vi "TC.vi"() -> ()   [LabVIEW 2013]
uses:
  lib/Lib.llb/CS mode.ctl
  lib/Lib.llb/R.ctl
  lib/Lib.llb/T.ctl
  lib/Lib.llb/Calibrations.ctl
  lib/Lib.llb/CS.lvclass
  lib/Lib.llb/PID Settings.ctl
  lib/Lib.llb/AVS_exc_n_ranges.ctl
  lib/Lib.llb/AVS_excitation.ctl
  lib/Lib.llb/AVS47_range.ctl
  lib/Lib.llb/Ch descriptions.ctl
  lib/Lib.llb/Cursor Controls.ctl
  lib/Lib.llb/DataArray.ctl
  lib/Lib.llb/Unit.ctl
  lib/Lib.llb/Control 6.ctl
  lib/Lib.llb/Control 4.ctl
  lib/Lib.llb/Control 8.ctl
  lib/Lib.llb/VI FPO Ref.ctl
  lib/Lib.llb/Class ID ENUM.ctl
  lib/Lib.llb/Type Descriptor Enumeration__ogtk.ctl
  lib/Lib.llb/Refnum Subtype Enum__ogtk.ctl
  lib/Lib.llb/Waveform Subtype Enum__ogtk.ctl
  lib/Lib.llb/LV Data cluster.ctl
  lib/Lib.llb/Action.ctl
  Leiden to DSC/TC to DSC/Typedefs/TC-cluster.ctl
  lib/Lib.llb/TCS.lvclass
  lib/Lib.llb/QCS.lvclass
  lib/Lib.llb/CS Emulation.lvclass
  lib/Lib.llb/PCS.lvclass
  lib/Lib.llb/Byte Params.ctl
panel:
  out "R_array":dbl[](array[numeric])
  out "SetControl":T1
  out "ControlNames":string[](array[string])
  out "VIRef":T2 {"Array DataType" format="%.0x"; "WaveForm Type" format="%.0x"; "RefNum Type" format="%.0x"; "DataType" format="%.0x"}
  out "zConfig":path=path "C:/Users/Sasha/Dropbox/Labview/LC Software/ImpSoft-V5.2.2-multithreaded/ImpBridgeLabview/ImpBridgeDll.dll"
  out "VI called?":bool=TRUE
  out "Error code":u8
  out "Set #":u8 caption="zBridge set nr."
  out "zDll":path=path "C:/Users/Sasha/Dropbox/Labview/LC Software/ImpSoft-V5.2.2-multithreaded/ImpBridgeLabview/ImpBridgeDll.dll"
  in  "String":string="^ Click the Run button to start the program "
  in  "Toolbar":enum32{"Page 1", "Page 2"}(tab)
  in  "Load config":bool
  in  "Start":bool
  in  "Load Data":bool
  in  "Pause":bool
  in  "Stop":bool
  in  "Copy to Clipboard":bool
  in  "Save to Cal Log":bool
  in  "Save config":bool
  in  "Clear all plots":bool
  in  "ColorBox":enum32{"Page 1", "Page 2"}(tab)
  in  "Colors":picture
  out "Color":u32(colorbox)
  in  "LogFileCreationTime":timestamp=timestamp(2742897600 s since 1904-01-01)
  out "Calib path":path=path "C:/avs-47/aaaa"
  out "Log path":path
  out "TCS port":i32(ring)=3 items=["COM1", "COM2", "COM3", "COM4", "COM5", "COM6", "COM7", "COM8", "COM9", "PRN1", "PRN2", "PRN3", "PRN4"]
  out "AVS VISA session":refnum<visa-resource-name>="COM3"
  in  "Minimize 2":bool
  out "Revision":string="TC" caption="V"
  in  "Minimize":bool
  out "Current1flow":bool
  out "Current2flow":bool
  in  "Tab Control":enum32{"AVS"}(tab)
  in  "Graph controls":enum32{"Page 1"}(tab)
  in  "Mode Buttons":T7
  in  "Erase all":bool
  in  "Plot-Save All":bool
  in  "Plot-save-screen":bool
  in  "Channel Controls":T8(tab)=enum."All"
  out "T0":dbl=nan caption="T" format="%#.2p"
  out "R0":dbl caption="R" format="%.3p"
  out "R-Plot 0":cluster{dbl[], dbl[]}(graph) caption="R-Plot"
  out "T1":dbl=nan caption="T" format="%#.2p"
  out "R1":dbl caption="R" format="%.3p"
  out "R-Plot 1":cluster{dbl[], dbl[]}(graph) caption="R-Plot"
  out "T2":dbl=nan caption="T" format="%#.2p"
  out "R2":dbl caption="R" format="%.3p"
  out "R-Plot 2":cluster{dbl[], dbl[]}(graph) caption="R-Plot"
  out "T3":dbl=nan caption="T" format="%#.2p"
  out "R3":dbl caption="R" format="%.3p"
  out "R-Plot 3":cluster{dbl[], dbl[]}(graph) caption="R-Plot"
  out "T4":dbl=nan caption="T" format="%#.2p"
  out "R4":dbl caption="R" format="%.3p"
  out "R-Plot 4":cluster{dbl[], dbl[]}(graph) caption="R-Plot"
  out "T5":dbl=nan caption="T" format="%#.2p"
  out "R5":dbl caption="R" format="%.3p"
  out "R-Plot 5":cluster{dbl[], dbl[]}(graph) caption="R-Plot"
  out "T6":dbl=nan caption="T" format="%#.2p"
  out "R6":dbl caption="R" format="%.3p"
  out "R-Plot 6":cluster{dbl[], dbl[]}(graph) caption="R-Plot"
  out "T7":dbl=nan caption="T" format="%#.2p"
  out "R7":dbl caption="R" format="%.3p"
  out "R-Plot 7":cluster{dbl[], dbl[]}(graph) caption="R-Plot"
  out "T8":dbl=nan caption="T" format="%#.2p"
  out "R8":dbl caption="R" format="%.3p"
  out "R-Plot 8":cluster{dbl[], dbl[]}(graph) caption="R-Plot"
  out "T9":dbl=nan caption="T" format="%#.2p"
  out "R9":dbl caption="R" format="%.3p"
  out "R-Plot 9":cluster{dbl[], dbl[]}(graph) caption="R-Plot"
  out "T":T9 {"T0 3" format="%.2p"; "T0 2" format="%.2p"; "T0" format="%.2p"; "T0" format="%.2p"; "T0" format="%.2p"; "T0" format="%.2p"; "T0" format="%.2p"; "T0" format="%.2p"; "T0" format="%.2p"; "T0" format="%.2p"}
  in  "AVS names":T10={"AVS Name 0"="3K", "AVS Name 1"="Still", "AVS Name 2"="50 mK", "AVS Name 3"="MC", "AVS Name 4"="MC", "AVS Name 5"="", "AVS Name 6"="", "AVS Name 7"="", "AVS Name 8"="", "AVS Name 9"=""}
  in  "Edit Calibrations":T11
  in  "Thermometer":T12 {"Select sensor 10" items=["No Calibration.vi"]; "Select sensor 9" items=["No Calibration.vi"]; "Select sensor 8" items=["No Calibration.vi"]; "Select sensor 7" items=["No Calibration.vi"]; "Select sensor 6" items=["No Calibration.vi"]; "Select sensor 5" items=["No Calibration.vi"]; "Select sensor 4" items=["No Calibration.vi"]; "Select sensor 3" items=["No Calibration.vi"]; "Select sensor 2" items=["No Calibration.vi"]; "Select sensor 1" items=["No Calibration.vi"]}
  out "Units":T13
  out "R":T14={"R0"=0.0, "R1"=0.0, "R2"=-0.0, "R3"=0.0, "R4"=0.0, "R5"=0.0, "R6"=0.0, "R7"=0.0, "R6 2"=0.0, "R7 2"=0.0} {"R7 2" format="%.3p"; "R6 2" format="%.3p"; "R7" format="%.3p"; "R6" format="%.3p"; "R5" format="%.3p"; "R4" format="%.3p"; "R3" format="%.3p"; "R2" format="%.3p"; "R1" format="%.3p"; "R0" format="%.3p"}
  in  "Scan Parameters":enum32{"Page 1", "Page 2"}(tab)
  in  "Exc&Ranges":T15={"Excitationl 0"=4, "Excitationl 0"=4, "Excitationl 0"=3, "Excitationl 0"=3, "Excitationl 0"=3, "Excitationl 0"=3, "Excitationl 0"=3, "Excitationl 0"=3, "Range 0"=5, "Range 0"=5, "Range 0"=5, "Range 0"=5, "Range 0"=5, "Range 0"=5, "Range 0"=5, "Range 0"=5} {"Range 0" items=["n.a."=-1, "open"=0, "2 Ohm"=1, "20 Ohm"=2, "200 Ohm"=3, "2k Ohm"=4, "20k Ohm"=5, "200k Ohm"=6, "2M Ohm"=7]; "Range 0" items=["n.a."=-1, "open"=0, "2 Ohm"=1, "20 Ohm"=2, "200 Ohm"=3, "2k Ohm"=4, "20k Ohm"=5, "200k Ohm"=6, "2M Ohm"=7]; "Range 0" items=["n.a."=-1, "open"=0, "2 Ohm"=1, "20 Ohm"=2, "200 Ohm"=3, "2k Ohm"=4, "20k Ohm"=5, "200k Ohm"=6, "2M Ohm"=7]; "Range 0" items=["n.a."=-1, "open"=0, "2 Ohm"=1, "20 Ohm"=2, "200 Ohm"=3, "2k Ohm"=4, "20k Ohm"=5, "200k Ohm"=6, "2M Ohm"=7]; "Range 0" items=["n.a."=-1, "open"=0, "2 Ohm"=1, "20 Ohm"=2, "200 Ohm"=3, "2k Ohm"=4, "20k Ohm"=5, "200k Ohm"=6, "2M Ohm"=7]; "Range 0" items=["n.a."=-1, "open"=0, "2 Ohm"=1, "20 Ohm"=2, "200 Ohm"=3, "2k Ohm"=4, "20k Ohm"=5, "200k Ohm"=6, "2M Ohm"=7]; "Range 0" items=["n.a."=-1, "open"=0, "2 Ohm"=1, "20 Ohm"=2, "200 Ohm"=3, "2k Ohm"=4, "20k Ohm"=5, "200k Ohm"=6, "2M Ohm"=7]; "Range 0" items=["n.a."=-1, "open"=0, "2 Ohm"=1, "20 Ohm"=2, "200 Ohm"=3, "2k Ohm"=4, "20k Ohm"=5, "200k Ohm"=6, "2M Ohm"=7]; "Excitationl 0" items=["none", "3 µV", "10 µV", "30 µV", "100 µV", "300 µV", "1 mV", "3 mV"]; "Excitationl 0" items=["none", "3 µV", "10 µV", "30 µV", "100 µV", "300 µV", "1 mV", "3 mV"]; "Excitationl 0" items=["none", "3 µV", "10 µV", "30 µV", "100 µV", "300 µV", "1 mV", "3 mV"]; "Excitationl 0" items=["none", "3 µV", "10 µV", "30 µV", "100 µV", "300 µV", "1 mV", "3 mV"]; "Excitationl 0" items=["none", "3 µV", "10 µV", "30 µV", "100 µV", "300 µV", "1 mV", "3 mV"]; "Excitationl 0" items=["none", "3 µV", "10 µV", "30 µV", "100 µV", "300 µV", "1 mV", "3 mV"]; "Excitationl 0" items=["none", "3 µV", "10 µV", "30 µV", "100 µV", "300 µV", "1 mV", "3 mV"]; "Excitationl 0" items=["none", "3 µV", "10 µV", "30 µV", "100 µV", "300 µV", "1 mV", "3 mV"]}
  out "Status":T18
  out "zBridge params":T19
  out "uPlots":T20
  in  "Autorange":bool=TRUE
  out "Active":T21={"active Channel 0"=TRUE, "active Channel 1"=TRUE, "active Channel 2"=TRUE, "active Channel 3"=FALSE, "active Channel 4"=FALSE, "active Channel 5"=FALSE, "active Channel 6"=FALSE, "active Channel 7"=FALSE, "active Channel 8"=FALSE, "active Channel 9"=FALSE}
  out "Waveform Chart":T22(graph)
  in  "HW Address":u32
  in  "Edit calibration":bool
  in  "Convert":bool
  out "T7":dbl caption="T=" format="%#.2p"
  in  "QuickR":dbl caption="R=" format="%_6g"
  in  "Select sensor 1":u16(ring) items=["No Calibration.vi"]
  out "I_list[i]":T23[](array[typedef]) min=-1.0
  out "I_in":T23[](array[typedef]) min=-1.0
  in  "Tab Control 5":enum32{"Page 1", "Page 2"}(tab)
  in  "Data History":enum32{"History", "Settings"}(tab)=enum."Settings"
  out "AVS names small":T10={"AVS Name 0"="3K", "AVS Name 1"="Still", "AVS Name 2"="50 mK", "AVS Name 3"="MC", "AVS Name 4"="MC", "AVS Name 5"="", "AVS Name 6"="", "AVS Name 7"="", "AVS Name 8"="", "AVS Name 9"=""}
  out "Active channel":T24
  out "Small T":T25 caption="T" {"R1" format="%#.2p"; "R1" format="%#.2p"; "R1" format="%#.2p"; "R1" format="%#.2p"; "R1" format="%#.2p"; "R1" format="%#.2p"; "R1" format="%#.2p"; "R1" format="%#.2p"; "R1" format="%#.2p"; "R1" format="%#.2p"}
  out "Small R":T26 caption="R" {"R1 2" format="%#_5p"; "R1 2" format="%#_5p"; "R1 2" format="%#_5p"; "R1 2" format="%#_5p"; "R1 2" format="%#_5p"; "R1 2" format="%#_5p"; "R1 2" format="%#_5p"; "R1 2" format="%#_5p"; "R1 2" format="%#_5p"; "R1 2" format="%#_5p"}
  out "Time":dbl format="%<%X\n%x>T"
  in  "Runtime Settings":T27={"Read AVS channels from"=0, "Last Channel"=7, "Delay Between Scans"=0, "Stabilisation Delay"=5.0, "Averages"=2, "Data Memory"=25000, "Filter graphs:"=FALSE, "Y_min"=0.0, "Y_max"=2000000.0, "Plot type"=enum."T vs Time", "Allow neg R"=TRUE, "Data Memory 2"=30.0} {"Data Memory 2" min=0.0; "Delay Between Scans" format="%.0f s"; "Averages" min=1 max=1000; "Stabilisation Delay" min=0.5; "Last Channel" min=0 max=7 step=1; "Read AVS channels from" min=0 max=7 step=1; "Y_max" format="%#_6f"; "Y_min" min=0.0 format="%#_6f"; "Data Memory" min=3 max=30000}
  in  "Numeric":dbl
  out "I":dbl[](array[numeric])
  in  "Data":T28=[{"R"=[], "T"=[], "Time"=[]}, {"R"=[0.0, 2.0], "T"=[], "Time"=[]}]
  out "Int":dbl=10.0 format="%#.2f"
  out "T_array":dbl[](array[numeric])
  in  "Data array":dbl[](array[numeric])
  out "I3_SetPnt":dbl
  out "Currents changed":bool
  in  "Excitations":T29={"Excitationl 0"=4, "Excitation 1"=4, "Excitation 2"=3, "Excitation 3"=3, "Excitation 4"=3, "Excitation 5"=3, "Excitation 6"=3, "Excitation 7"=3} {"Excitation 7" items=["none", "3 µV", "10 µV", "30 µV", "100 µV", "300 µV", "1 mV", "3 mV"]; "Excitation 6" items=["none", "3 µV", "10 µV", "30 µV", "100 µV", "300 µV", "1 mV", "3 mV"]; "Excitation 5" items=["none", "3 µV", "10 µV", "30 µV", "100 µV", "300 µV", "1 mV", "3 mV"]; "Excitation 4" items=["none", "3 µV", "10 µV", "30 µV", "100 µV", "300 µV", "1 mV", "3 mV"]; "Excitation 3" items=["none", "3 µV", "10 µV", "30 µV", "100 µV", "300 µV", "1 mV", "3 mV"]; "Excitation 2" items=["none", "3 µV", "10 µV", "30 µV", "100 µV", "300 µV", "1 mV", "3 mV"]; "Excitation 1" items=["none", "3 µV", "10 µV", "30 µV", "100 µV", "300 µV", "1 mV", "3 mV"]; "Excitationl 0" items=["none", "3 µV", "10 µV", "30 µV", "100 µV", "300 µV", "1 mV", "3 mV"]}
  in  "Ranges":T29={"Excitationl 0"=5, "Excitation 1"=5, "Excitation 2"=5, "Excitation 3"=5, "Excitation 4"=5, "Excitation 5"=5, "Excitation 6"=5, "Excitation 7"=5} {"Excitation 7" items=["n.a."=-1, "open"=0, "2 Ohm"=1, "20 Ohm"=2, "200 Ohm"=3, "2k Ohm"=4, "20k Ohm"=5, "200k Ohm"=6, "2M Ohm"=7]; "Excitation 6" items=["n.a."=-1, "open"=0, "2 Ohm"=1, "20 Ohm"=2, "200 Ohm"=3, "2k Ohm"=4, "20k Ohm"=5, "200k Ohm"=6, "2M Ohm"=7]; "Excitation 5" items=["n.a."=-1, "open"=0, "2 Ohm"=1, "20 Ohm"=2, "200 Ohm"=3, "2k Ohm"=4, "20k Ohm"=5, "200k Ohm"=6, "2M Ohm"=7]; "Excitation 4" items=["n.a."=-1, "open"=0, "2 Ohm"=1, "20 Ohm"=2, "200 Ohm"=3, "2k Ohm"=4, "20k Ohm"=5, "200k Ohm"=6, "2M Ohm"=7]; "Excitation 3" items=["n.a."=-1, "open"=0, "2 Ohm"=1, "20 Ohm"=2, "200 Ohm"=3, "2k Ohm"=4, "20k Ohm"=5, "200k Ohm"=6, "2M Ohm"=7]; "Excitation 2" items=["n.a."=-1, "open"=0, "2 Ohm"=1, "20 Ohm"=2, "200 Ohm"=3, "2k Ohm"=4, "20k Ohm"=5, "200k Ohm"=6, "2M Ohm"=7]; "Excitation 1" items=["n.a."=-1, "open"=0, "2 Ohm"=1, "20 Ohm"=2, "200 Ohm"=3, "2k Ohm"=4, "20k Ohm"=5, "200k Ohm"=6, "2M Ohm"=7]; "Excitationl 0" items=["n.a."=-1, "open"=0, "2 Ohm"=1, "20 Ohm"=2, "200 Ohm"=3, "2k Ohm"=4, "20k Ohm"=5, "200k Ohm"=6, "2M Ohm"=7]}
  out "CS ref":refnum<class "CS.lvclass">
  out "start 2":bool
  in  "Current indicators":enum32{"Page 1", "Page 2"}(tab)
  out "Automatic mode 0":bool
  out "Automatic mode 1":bool
  out "Map Channel 0 to 2":T30(ring) caption="Output to"
  in  "uA 0":u32
  in  "CS Names":T31={"CS Name 0"="N.C.", "CS Name 1"="3K", "CS Name 2"="Still", "CS Name 3"="MC"}
  out "I0":T32={"uA"="000", "ON"=FALSE, "Gated"=FALSE, "current flows"=FALSE, "Error"=FALSE} caption="Ch0 -"
  in  "uA 3":u32
  in  "uA 2":u32
  in  "uA 1":u32
  out "Automatic mode 3":bool
  out "Automatic mode 2":bool
  out "I3":T32={"uA"="000", "ON"=FALSE, "Gated"=FALSE, "current flows"=FALSE, "Error"=FALSE} caption="Chn 3"
  out "I2":T32={"uA"="000", "ON"=FALSE, "Gated"=FALSE, "current flows"=FALSE, "Error"=FALSE} caption="Chn 2"
  out "I1":T32={"uA"="000", "ON"=FALSE, "Gated"=FALSE, "current flows"=FALSE, "Error"=FALSE} caption="Chn 1"
  out "I_0":dbl=10.0
  out "vi reference":refnum<vi>
  out "Small I":cluster{"I1":dbl, "I2":dbl, "I3":dbl, "I4":dbl} caption="I" {"I1" format="%#.2f"; "I2" format="%#.2p"; "I3" format="%#.2p"; "I4" format="%#.2p"}
  out "Actual I":dbl[](array[numeric])
  in  "Save Data 2":bool
  in  "Show PID graph?":bool
  in  "Set Color":bool
  out "Unit":string
  out "Par/Err":string caption="zBridge params/Error"
  out "CurCalibrations":T33
  out "LMB Down":bool
  in  "Tab Control 2":T34(tab)
  in  "Refresh Calibrations":bool
  in  "zBridge settings":bool
  out "ID":string
  out "CS status":errorcluster
  out "General":errorcluster caption="General status"
  in  "Bridge settings":T35={"AVS type"=enum."AVS47A (GPIB interface)", "AVS_SPort"="COM5", "Address"="GPIB0::20::INSTR", "AVS_CalFolder"=path "E:/Dropbox/Labview/LC Software/All Calibrations"}
  in  "Current source settings":T36={"TCS_Port"="COM1", "TCS_Imax"=5, "CS type"=enum."TCS", "QCS/PCS Device"=0}
  in  "Data logging":T37={"AVS_Path"=path "C:/avs-47", "AVS_FName"="LogAVS", "CAL_FName"="calibration", "Filenames suffix"="_%Y-%m-%d-%H-%M-%S", "Delimeter"="\t", "NewFevery"=7, "Time Units"=enum."Days", "Date/Time Format"="%Y-%m-%d %H:%M:%S", "External VI path"=path "C:/Users/User1/Dropbox/Labview/LC Software/TempControl/OnTempStabilized Ext VI Laurens.vi", "Ask on start?"=FALSE, "Run description"="\n"}
  out "Bridge status":errorcluster
  in  "I0 output to":T38(ring) caption="Set Channel 0 output to"
  in  "CS Mode":T39 caption="CS mode"
  out "Time Old":dbl format="%#_16g"
  in  "CS modes":T40(tab)=enum."Automatic 1"
  in  "C_I0 4":T41={"Toggle ON/OFF"=FALSE, "Toggle Gated"=FALSE, "I"=0, "Range"=enum."x1 uA"} caption="Chn 3" {"I" max=100000 step=1}
  in  "C_I0 3":T41={"Toggle ON/OFF"=FALSE, "Toggle Gated"=FALSE, "I"=0, "Range"=enum."x1 uA"} caption="Chn 2" {"I" max=100000 step=1}
  in  "C_I0 2":T41={"Toggle ON/OFF"=FALSE, "Toggle Gated"=FALSE, "I"=0, "Range"=enum."x1 uA"} caption="Chn 1" {"I" max=100000 step=1}
  in  "C_I0":T41={"Toggle ON/OFF"=FALSE, "Toggle Gated"=FALSE, "I"=0, "Range"=enum."x1 uA"} caption="Chn 0" {"I" max=100000 step=1}
  in  "Mode1 ON":bool
  in  "I_list":T23[][](array[typedef]) min=-1.0
  out "T Channel":T42[](array[typedef])
  out "I_selection":T43[](array[typedef])=[TRUE, FALSE, FALSE, FALSE, FALSE, FALSE, FALSE, FALSE, FALSE, FALSE]
  out "SP reached?":bool
  out "Error":dbl=10.0 format="%#_6f"
  out "Slope":dbl format="%#_3g %"
  out "Timer":dbl format="%<%H:%M:%S>t"
  out "I_list_idx_max":i32=10 caption="/"
  out "I_list_idx":i32=10 caption="Point #"
  in  "Next step":bool
  in  "Reset PID":bool
  in  "PID setup":T44={"Current limit, [uA]"=10000.0, "Proportional Gain"=3.0, "Integral Gain"=3.0, "Derivative Gain"=1.0, "SP tolerance"=0.1, "Feed Fwd Gain [uA/mK]"=0.0, "Integral Gain Bandwidth"=10.0, "Integral Gain Background"=1.0, "FB on 2"=enum."1"} {"Integral Gain Background" format="%#.6g"; "Integral Gain Bandwidth" format="%#.6g"; "Feed Fwd Gain [uA/mK]" format="%#.5g"; "SP tolerance" format="%#.5g"; "Derivative Gain" format="%#.6g"; "Integral Gain" format="%#.6g"; "Proportional Gain" format="%#.6g"; "Current limit, [uA]" format="%#.5g"}
  in  "Automode 2":bool=TRUE caption="Enable automatic sweeping/list iteration"
  in  "Automode Settings 2":T45={"AVS Channel"=0, "N averages"=10, "Delay Time"=10.0, "T stability"=0.3, "FB on"=enum."Temperature"} {"Delay Time" min=0.0 format="%#_g min"; "AVS Channel" min=-1 max=9 step=1}
  in  "Call ext. VI":bool
  out "- state":T46(ring)
  in  "Trigger other running TC instances":bool
  in  "I_prev":bool
  in  "I_next":bool
  in  "I_tofirst":bool
  in  "Save to file":bool
  in  "Load from file":bool
  in  "Write to log":bool
  in  "I3 as temp":cluster{"I3 as temp 2":bool}
  in  "I_Clear":bool
  in  "Mode2 ON":bool
  in  "FB on":enum16{"Resistance", "Temperature"}(ring)=enum."Temperature" caption="Read"
  in  "AVS Channel":i32 caption="on channel" min=-1 max=9 step=1
  in  "Add Range":bool
  in  "Array":dbl[](array[numeric])=[0.0, 0.0, 0.0, 0.0, 0.0, 0.0] caption="New range" min=-1.0
  in  "I_list 2":dbl[][](array[numeric])=[[0.0, 0.0, 0.0, 0.0, 0.0, inf]] min=-1.0
  out "I_selection 2":T43[](array[typedef])=[TRUE, FALSE, FALSE, FALSE, FALSE, FALSE, FALSE, FALSE, FALSE, FALSE]
  in  "CS Ch3 mode":enum32{"Page 1", "Page 2"}(tab)=enum."Page 2"
  in  "T Sweep":T47={"Start value"=200.0, "End value"=250.0, "Step"=10.0, "Current"=0.0, "I_next"=FALSE, "I_prev"=FALSE, "Interrrupt Sweep"=FALSE, "Start"=FALSE, "Boolean"=TRUE} {"Step" min=0.0; "End value" min=0.0; "Start value" min=0.0}
  # "Quick convert R->T:"
  # "Ohm"
  # "mK"
  # "Ch#"
  # "Miniplot"
  # "Channel parameters"
  # "Impedance"
  # "Unit"
  # "Type of sensor"
  # "T [mK]"
  # "Description"
  # "0"
  # "1"
  # "2"
  # "3"
  # "4"
  # "5"
  # "6"
  # "7"
  # "8"
  # "9"
  # "0"
  # "1"
  # "2"
  # "3"
  # "4"
  # "5"
  # "7"
  # "8"
  # "9"
  # "6"
  # "auto"
  # "auto"
  # "auto"
  # "auto"
  # "gated"
  # "gated"
  # "gated"
  # "gated"
  # "Status"
  # "Current source mode"
  # "Current source manual control"
  # "Current source automatic mode #1"
  # "Currents List"
  # "Settings"
  # "I0"
  # "I1"
  # "I2"
  # "I3"
  # "Status"
  # "On temperature stabilized"
  # "Current source automatic mode #2"
  # "Currents List"
  # "Settings"
  # "T0"
  # "T1"
  # "I0"
  # "I1"
  # "I2"
  # "I3"
  # "T0"
  # "T1"
  # "I0"
  # "I1"
  # "I2"
  # "I3"
  # "Ch3"
types:
  T1 = typedef "LV Data cluster.ctl" = cluster{"Name":string, "Scalar":string, "Array":string[][]}
  T2 = typedef "VI FPO Ref.ctl" = cluster{"Control Ref ID":refnum<vi>[], "Full Name":string[], "ClassID":T3[], "Short Name":string[], "DataType":T4[], "RefNum Type":T5[], "WaveForm Type":T6[], "Parent":i32[], "Array DataType":T4[], "Owning VI":refnum<vi>[], "Active?":bool[]}
  T3 = typedef "Class ID ENUM.ctl" = enum16{"<Null>", "1", "2", "Generic", "Decoration", "Text", "Control", "ColorBox", "Boolean", "RefNum", "Variant", "Path", "ListBox", "Table", "Array", "Picture", "ActiveXContainer", "Numeric", "Digital", "NamedNumeric", "ColorRamp", "Slide", "GraphOrChart", "WaveformChart", "WaveformGraph", "IntensityChart", "IntensityGraph", "String", "IOName", "ComboBox", "Cluster", "Panel", "Knob", "NumWithScale", "Ring", "Enum", "GObject", "Plot", "Cursor", "NumericText", "Scale", "ColorScale", "GraphScale", "ColorGraphScale", "TypedRefNum", "OldKnobScale", "MCListbox", "MeasureData", "BVTag", "DAQName", "VISAName", "IVIName", "SlideScale", "TabControl", "Page", "TabArrayTabControl", "ConPane", "57", "58", "59", "60", "61", "62", "63", "64", "SubPanel", "TreeControl", "67", "68", "69", "70", "71", "72", "73", "74", "75", "SplitterBar"}
  T4 = typedef "Type Descriptor Enumeration__ogtk.ctl" = enum8{"<Null>", "I8", "I16", "I32", "I64", "U8", "U16", "U32", "U64", "SGL", "DBL", "EXT", "CSG", "CDB", "CXT", "0x0F", "0x10", "0x11", "0x12", "0x13", "0x14", "Enum U8", "Enum U16", "Enum U32", "Enum U64", "SGL PQ", "DBL PQ", "EXT PQ", "CSG PQ", "CDB PQ", "CXT PQ", "0x1F", "0x20", "Boolean", "0x22", "0x23", "0x24", "0x25", "0x26", "0x27", "0x28", "0x29", "0x2A", "0x2B", "0x2C", "0x2D", "0x2E", "0x2F", "String", "0x31", "Path", "Pict", "0x34", "0x35", "0x36", "DAQ", "0x38", "0x39", "0x3A", "0x3B", "0x3C", "0x3D", "0x3E", "0x3F", "Array", "0x41", "0x42", "0x43", "0x44", "0x45", "0x46", "0x47", "0x48", "0x49", "0x4A", "0x4B", "0x4C", "0x4D", "0x4E", "0x4F", "Cluster", "0x51", "0x52", "Variant", "Waveform", "0x55", "0x56", "0x57", "0x58", "0x59", "0x5A", "0x5B", "0x5C", "0x5D", "0x5E", "0x5F", "0x60", "0x61", "0x62", "0x63", "0x64", "0x65", "0x66", "0x67", "0x68", "0x69", "0x6A", "0x6B", "0x6C", "0x6D", "0x6E", "0x6F", "Refnum"}
  T5 = typedef "Refnum Subtype Enum__ogtk.ctl" = enum8{"Generic", "Datalog File Refnum", "Byte Stream File Refnum", "Device Refnum", "Occurence Refnum", "TCP Connection Refnum", "VISA Refnum (Obsolete)", "Automation Renum", "VI Server Refnum", "Menu Refnum", "IVI Refnum (Obsolete)", "IMAQ Session", "0x0C", "Datasocket Refnum", "VISA Resource", "IVI Logical Name", "UDP Connection Refnum", "Notifier Refnum", "Queue Refnum", "IrDA Refnum", "Hardware Plugin Refnum", "Hardware Plugin Tag Refnum", "DAQmx Refnum", "Event Registration Refnum", ".NET Refnum", "User Event Refnum", "0x1A", "Event Callback", "0x1C", "0x1D", "Only Used Internal to LabVIEW", "Bluetooth", "Data Value References", "RT FIFO", "TDM Streaming"}
  T6 = typedef "Waveform Subtype Enum__ogtk.ctl" = enum8{"<Not a Waveform Type>", "0x01", "Analog 16-bit signed", "Analog Double-Precision", "0x04", "Analog Single Precision", "Timestamp", "Digital Data", "Digital Waveform", "Dynamic Data", "Analog Extended-Precision", "Analog 8-bit unsigned", "Analog 16-bit unsigned", "Analog 32-bit unsigned", "Analog 8-bit signed", "Analog 32-bit signed", "Analog Complex Single-Precision", "Analog Complex Double-Precision", "Analog Complex Extended Precision", "Analog 64-bit signed", "Analog 64-bit unsigned"}
  T7 = typedef "Cursor Controls.ctl" = enum32{"No Selection", "Cursor mode", "Erase point", "Erase range"}
  T8 = enum32{"0", "1", "2", "3", "4", "5", "6", "7", "8", "9", "All", "PID loop"}
  T9 = typedef "T.ctl" = cluster{"T0":dbl, "T0":dbl, "T0":dbl, "T0":dbl, "T0":dbl, "T0":dbl, "T0":dbl, "T0":dbl, "T0 2":dbl, "T0 3":dbl}
  T10 = typedef "Ch descriptions.ctl" = cluster{"AVS Name 0":string, "AVS Name 1":string, "AVS Name 2":string, "AVS Name 3":string, "AVS Name 4":string, "AVS Name 5":string, "AVS Name 6":string, "AVS Name 7":string, "AVS Name 8":string, "AVS Name 9":string}
  T11 = cluster{"Boolean":bool, "Boolean 2":bool, "Boolean 3":bool, "Boolean 4":bool, "Boolean 5":bool, "Boolean 6":bool, "Boolean 7":bool, "Boolean 8":bool, "Boolean 9":bool, "Boolean 10":bool}
  T12 = typedef "Calibrations.ctl" = cluster{"Select sensor 1":u16, "Select sensor 2":u16, "Select sensor 3":u16, "Select sensor 4":u16, "Select sensor 5":u16, "Select sensor 6":u16, "Select sensor 7":u16, "Select sensor 8":u16, "Select sensor 9":u16, "Select sensor 10":u16}
  T13 = typedef "Unit.ctl" = cluster{"AVS Name 0":string, "AVS Name 1":string, "AVS Name 2":string, "AVS Name 3":string, "AVS Name 4":string, "AVS Name 5":string, "AVS Name 6":string, "AVS Name 7":string, "AVS Name 8":string, "AVS Name 9":string}
  T14 = typedef "R.ctl" = cluster{"R0":dbl, "R1":dbl, "R2":dbl, "R3":dbl, "R4":dbl, "R5":dbl, "R6":dbl, "R7":dbl, "R6 2":dbl, "R7 2":dbl}
  T15 = typedef "AVS_exc_n_ranges.ctl" = cluster{"Excitationl 0":T16, "Excitationl 0":T16, "Excitationl 0":T16, "Excitationl 0":T16, "Excitationl 0":T16, "Excitationl 0":T16, "Excitationl 0":T16, "Excitationl 0":T16, "Range 0":T17, "Range 0":T17, "Range 0":T17, "Range 0":T17, "Range 0":T17, "Range 0":T17, "Range 0":T17, "Range 0":T17}
  T16 = typedef "AVS_excitation.ctl" = i16
  T17 = typedef "AVS47_range.ctl" = i16
  T18 = cluster{"Numeric":dbl, "Numeric":dbl, "Numeric":dbl, "Numeric":dbl, "Numeric":dbl, "Numeric":dbl, "Numeric":dbl, "Numeric":dbl, "Numeric":dbl, "Numeric":dbl}
  T19 = cluster{"AVS Name 0":string, "AVS Name 1":string, "AVS Name 2":string, "AVS Name 3":string, "AVS Name 4":string, "AVS Name 5":string, "AVS Name 6":string, "AVS Name 7":string, "AVS Name 8":string, "AVS Name 9":string}
  T20 = cluster{"uPlot 0":cluster{dbl[], dbl[]}, "uPlot 1":cluster{dbl[], dbl[]}, "uPlot 2":cluster{dbl[], dbl[]}, "uPlot 3":cluster{dbl[], dbl[]}, "uPlot 4":cluster{dbl[], dbl[]}, "uPlot 5":cluster{dbl[], dbl[]}, "uPlot 6":cluster{dbl[], dbl[]}, "uPlot 7":cluster{dbl[], dbl[]}, "uPlot 8":cluster{dbl[], dbl[]}, "uPlot 9":cluster{dbl[], dbl[]}}
  T21 = cluster{"active Channel 0":bool, "active Channel 1":bool, "active Channel 2":bool, "active Channel 3":bool, "active Channel 4":bool, "active Channel 5":bool, "active Channel 6":bool, "active Channel 7":bool, "active Channel 8":bool, "active Channel 9":bool}
  T22 = cluster{"Ip":dbl, "Ii":dbl, "Id":dbl, "Iff":dbl, "I_tot":dbl}
  T23 = typedef "Control 4.ctl" = dbl
  T24 = cluster{"Boolean 5":bool, "Boolean 5":bool, "Boolean 5":bool, "Boolean 5":bool, "Boolean 5":bool, "Boolean 5":bool, "Boolean 5":bool, "Boolean 5":bool, "Boolean 5":bool, "Boolean 5":bool}
  T25 = cluster{"R1":dbl, "R1":dbl, "R1":dbl, "R1":dbl, "R1":dbl, "R1":dbl, "R1":dbl, "R1":dbl, "R1":dbl, "R1":dbl}
  T26 = cluster{"R1 2":dbl, "R1 2":dbl, "R1 2":dbl, "R1 2":dbl, "R1 2":dbl, "R1 2":dbl, "R1 2":dbl, "R1 2":dbl, "R1 2":dbl, "R1 2":dbl}
  T27 = cluster{"Read AVS channels from":i8, "Last Channel":i8, "Delay Between Scans":u32, "Stabilisation Delay":dbl, "Averages":u16, "Data Memory":u16, "Filter graphs:":bool, "Y_min":dbl, "Y_max":dbl, "Plot type":enum16{"R vs Time", "T vs Time"}, "Allow neg R":bool, "Data Memory 2":dbl}
  T28 = typedef "DataArray.ctl" = cluster{"R":dbl[], "T":dbl[], "Time":dbl[]}[]
  T29 = cluster{"Excitationl 0":i16, "Excitation 1":i16, "Excitation 2":i16, "Excitation 3":i16, "Excitation 4":i16, "Excitation 5":i16, "Excitation 6":i16, "Excitation 7":i16}
  T30 = enum16{"Chn 0", "Aux 0", "Aux 1", "Aux 2", "Aux 3"}
  T31 = cluster{"CS Name 0":string, "CS Name 1":string, "CS Name 2":string, "CS Name 3":string}
  T32 = cluster{"uA":string, "ON":bool, "Gated":bool, "current flows":bool, "Error":bool}
  T33 = cluster{"[0]":string, "[1]":string, "[2]":string, "[3]":string, "[4]":string, "[5]":string, "[6]":string, "[7]":string, "[8]":string, "[9]":string}
  T34 = enum32{"Devices Settings", "Current source control"}
  T35 = cluster{"AVS type":enum16{"AVS47A (GPIB interface)", "AVS47B (RS232 interface)", "AVS48SI (RS232 interface)", "AVS Emulation", "Impedance Bridge", "Disabled"}, "AVS_SPort":refnum<visa-resource-name>, "Address":refnum<visa-resource-name>, "AVS_CalFolder":path}
  T36 = cluster{"TCS_Port":refnum<visa-resource-name>, "TCS_Imax":i32, "CS type":enum16{"TCS", "QCS v1", "PCS (n.a.)", "CS Emulation", "Disabled"}, "QCS/PCS Device":u16}
  T37 = cluster{"AVS_Path":path, "AVS_FName":string, "CAL_FName":string, "Filenames suffix":string, "Delimeter":string, "NewFevery":u32, "Time Units":enum16{"Minutes", "Hours", "Days"}, "Date/Time Format":string, "External VI path":path, "Ask on start?":bool, "Run description":string}
  T38 = enum16{"Channel 0", "Aux 0", "Aux 1", "Aux 2", "Aux 3"}
  T39 = typedef "CS mode.ctl" = enum16{"Manual", "Mode 1", "Mode2"}
  T40 = enum32{"Manual", "Automatic 1", "Automatic 2", "Automatic 3"}
  T41 = cluster{"Toggle ON/OFF":bool, "Toggle Gated":bool, "I":u32, "Range":enum8{"Auto", "x1 uA", "x10 uA", "x100 uA", "x1 mA"}}
  T42 = typedef "Control 8.ctl" = bool
  T43 = typedef "Control 6.ctl" = bool
  T44 = typedef "PID Settings.ctl" = cluster{"Current limit, [uA]":dbl, "Proportional Gain":dbl, "Integral Gain":dbl, "Derivative Gain":dbl, "SP tolerance":dbl, "Feed Fwd Gain [uA/mK]":dbl, "Integral Gain Bandwidth":dbl, "Integral Gain Background":dbl, "FB on 2":enum16{"0", "1", "2", "3"}}
  T45 = cluster{"AVS Channel":i32, "N averages":i32, "Delay Time":dbl, "T stability":dbl, "FB on":enum16{"Resistance", "Temperature"}}
  T46 = enum32{"Bad", "Idle", "Run top level", "Running"}
  T47 = cluster{"Start value":dbl, "End value":dbl, "Step":dbl, "Current":dbl, "I_next":bool, "I_prev":bool, "Interrrupt Sweep":bool, "Start":bool, "Boolean":bool}
  T48 = cluster{"UpdateChannelInfo":refnum<user-event>, "UpdateValuesAVS":refnum<user-event>, "UpdateCalibrations":refnum<user-event>, "UpdateLogFilePath":refnum<user-event>, "TempStabilized":refnum<user-event>, "Reset PID loop":refnum<user-event>, "UpdateValuesZBridge":refnum<user-event>, "CS Automode":refnum<user-event>, "CallExtVI":refnum<user-event>, "Data Array":refnum<user-event>}
  T49 = enum32{"Page Enabled", "Page Disabled", "Page Disabled & Grayed"}
  T50 = cluster{"error":bool, "code":i32, "source":string}
  T51 = typedef "Action.ctl" = enum16{"Init", "Write", "Read"}
  T52 = enum16{"AVS47A (GPIB interface)", "AVS47B (RS232 interface)", "AVS48", "AVS Emulation", "Impedance Bridge", "Disabled"}
  T53 = typedef "TC-cluster.ctl" = cluster{"R":dbl[], "T":dbl[], "I":dbl[], "AVS type":enum16{"AVS47A (GPIB interface)", "AVS47B (RS232 interface)", "AVS48", "AVS Emulation", "Impedance Bridge", "Disabled"}, "AVS names":cluster{"AVS Name 0":string, "AVS Name 1":string, "AVS Name 2":string, "AVS Name 3":string, "AVS Name 4":string, "AVS Name 5":string, "AVS Name 6":string, "AVS Name 7":string, "AVS Name 8":string, "AVS Name 9":string}, "Calibration":refnum<vi>[]}
  T54 = enum32{"No Selection", "Cursor mode", "Erase point", "Erase range"}
  T55 = enum16{"TCS", "QCS v1", "PCS (n.a.)", "CS Emulation", "Disabled"}
  T56 = enum8{"Auto", "x1 uA", "x10 uA", "x100 uA", "x1 mA"}
  T57 = cluster{"Cluster":cluster{"Time":dbl[], "T":dbl[]}, "Cluster":cluster{"Time":dbl[], "T":dbl[]}, "Cluster":cluster{"Time":dbl[], "T":dbl[]}, "Cluster":cluster{"Time":dbl[], "T":dbl[]}, "Cluster":cluster{"Time":dbl[], "T":dbl[]}, "Cluster":cluster{"Time":dbl[], "T":dbl[]}, "Cluster":cluster{"Time":dbl[], "T":dbl[]}, "Cluster":cluster{"Time":dbl[], "T":dbl[]}, "Cluster":cluster{"Time":dbl[], "T":dbl[]}, "Cluster":cluster{"Time":dbl[], "T":dbl[]}}
  T58 = enum32{"HKEY_CLASSES_ROOT", "HKEY_CURRENT_USER", "HKEY_LOCAL_MACHINE", "HKEY_USERS", "HKEY_PERFORMANCE_DATA", "HKEY_CURRENT_CONFIG", "HKEY_DYN_DATA"}
  T59 = enum32{"invalid app kind", "Development System", "Run Time System", "Student Edition", "Embedded LabVIEW", "Evaluation", "Custom"}
  T60 = enum16{"AVS47A (GPIB interface)", "AVS47B (RS232 interface)", "AVS48SI (RS232 interface)", "AVS Emulation", "Impedance Bridge", "Disabled"}
  T61 = cluster{"[0]":dbl, "[1]":dbl, "[2]":dbl, "[3]":dbl, "[4]":dbl, "[5]":dbl, "[6]":dbl, "[7]":dbl, "[8]":dbl, "[9]":dbl}
  T62 = cluster{"Temperature[0]":dbl, "Temperature[1]":dbl, "Temperature[2]":dbl, "Temperature[3]":dbl, "Temperature[4]":dbl, "Temperature[5]":dbl, "Temperature[6]":dbl, "Temperature[7]":dbl, "Temperature[8]":dbl, "Temperature[9]":dbl}
  T63 = cluster{"Current Time (double)":dbl, "R":dbl[], "T":dbl[]}
  T64 = typedef "File Info Record__ogtk.ctl" = cluster{"type":string, "creator":string, "permissions":i32, "data size":i32, "res size":i32, "creation date":u32, "modification date":u32, "bFolder":bool, "bInvisible":bool, "location":cluster{"vertical":i16, "horizontal":i16}, "owner":string, "group":string}
  T65 = cluster{"Units[0]":string, "Units[1]":string, "Units[2]":string, "Units[3]":string, "Units[4]":string, "Units[5]":string, "Units[6]":string, "Units[7]":string, "Units[8]":string, "Units[9]":string}
  T66 = cluster{"zBridge params[0]":string, "zBridge params[1]":string, "zBridge params[2]":string, "zBridge params[3]":string, "zBridge params[4]":string, "zBridge params[5]":string, "zBridge params[6]":string, "zBridge params[7]":string, "zBridge params[8]":string, "zBridge params[9]":string}
  T67 = cluster{"date/time string":string, "Value":dbl[], "Value":dbl[], "Value":dbl[]}
  T68 = typedef "imagedata.ctl" = cluster{"image type":i32, "image depth":i32, "image":u8[], "mask":u8[], "colors":u32[], "Rectangle":cluster{"left":i16, "top":i16, "right":i16, "bottom":i16}}
  T69 = typedef "LVPoint32TypeDef.ctl" = cluster{"Horizontal":i32, "Vertical":i32}
  T70 = cluster{"Shift":bool, "Ctrl":bool, "Alt":bool, "Cmd":bool, "Opt":bool}
  T71 = cluster{"Output Array":dbl[], "array w/ subset deleted":dbl[], "array w/ subset deleted":dbl[]}
  T72 = typedef "LVRectTypeDef.ctl" = cluster{"Left":i16, "Top":i16, "Right":i16, "Bottom":i16}
  T73 = typedef "Exc_n_Ranges.ctl" = cluster{"Excitationl 0":i16, "Excitation 1":i16, "Excitation 2":i16, "Excitation 3":i16, "Excitation 4":i16, "Excitation 5":i16, "Excitation 6":i16, "Excitation 7":i16, "Range 0":i16, "Range 1":i16, "Range 2":i16, "Range 3":i16, "Range 4":i16, "Range 5":i16, "Range 6":i16, "Range 7":i16}
  T74 = typedef "Byte Params.ctl" = enum8{"Active", "Channel Type", "Channel No", "Reference No", "RLC select", "Save Data", "L Inverted", "Menu Active"}
  T75 = typedef "LVPositionTypeDef.ctl" = cluster{"Left":i32, "Top":i32}
  T76 = cluster{"Range 0":i16, "Range 1":i16, "Range 2":i16, "Range 3":i16, "Range 4":i16, "Range 7":i16, "Range 5":i16, "Range 6":i16}
  T77 = cluster{"Range 0":i16, "Range 1":i16, "Range 2":i16, "Range 3":i16, "Range 4":i16, "Range 5":i16, "Range 6":i16, "Range 7":i16}
  T78 = cluster{"RANGE 0":u16, "RANGE 1":u16, "RANGE 2":u16, "RANGE 3":u16, "RANGE 4":u16, "RANGE 5":u16, "RANGE 6":u16, "RANGE 7":u16}
  T79 = typedef "LCR Channel parameters.ctl" = cluster{"Set_number":u8, "Set_char":u16, "Ch_number":u8, "Ch_type":u8, "Freq":dbl, "T_int":dbl, "I_exc":dbl, "V_exc":dbl, "SNR":dbl, "Vnoise":dbl, "P_diss":dbl}
  T80 = typedef "CS Data.ctl" = cluster{"Range":u8, "Current":dbl, "Current (string)":string, "On?":bool, "G?":bool, "I?":bool, "Err?":bool}
  T81 = typedef "TCS indicator.ctl" = cluster{"uA":string, " ON":bool, "Gated":bool, "current flows":bool, "Error":bool}
  T82 = cluster{"Toggle ON/OFF":bool, "Toggle Gated":bool}
  T83 = cluster{"Current":u32, "Range":enum16{"Auto", "x1 uA", "x10 uA", "x100 uA", "x1 mA"}}
  T84 = typedef "TCS manual control.ctl" = cluster{"Toggle ON/OFF":bool, "Toggle Gated":bool, "Current":u32, "Range":enum8{"Auto", "x1 uA", "x10 uA", "x100 uA", "x1 mA"}}
  T85 = cluster{"Status[0]":i32, "Status[1]":i32, "Status[2]":i32, "Status[3]":i32, "Status[4]":i32, "Status[5]":i32, "Status[6]":i32, "Status[7]":i32, "Status[8]":i32, "Status[9]":i32}
  T86 = cluster{"Active":bool, "Active":bool, "Active":bool, "Active":bool, "Active":bool, "Active":bool, "Active":bool, "Active":bool, "Active":bool, "Active":bool}
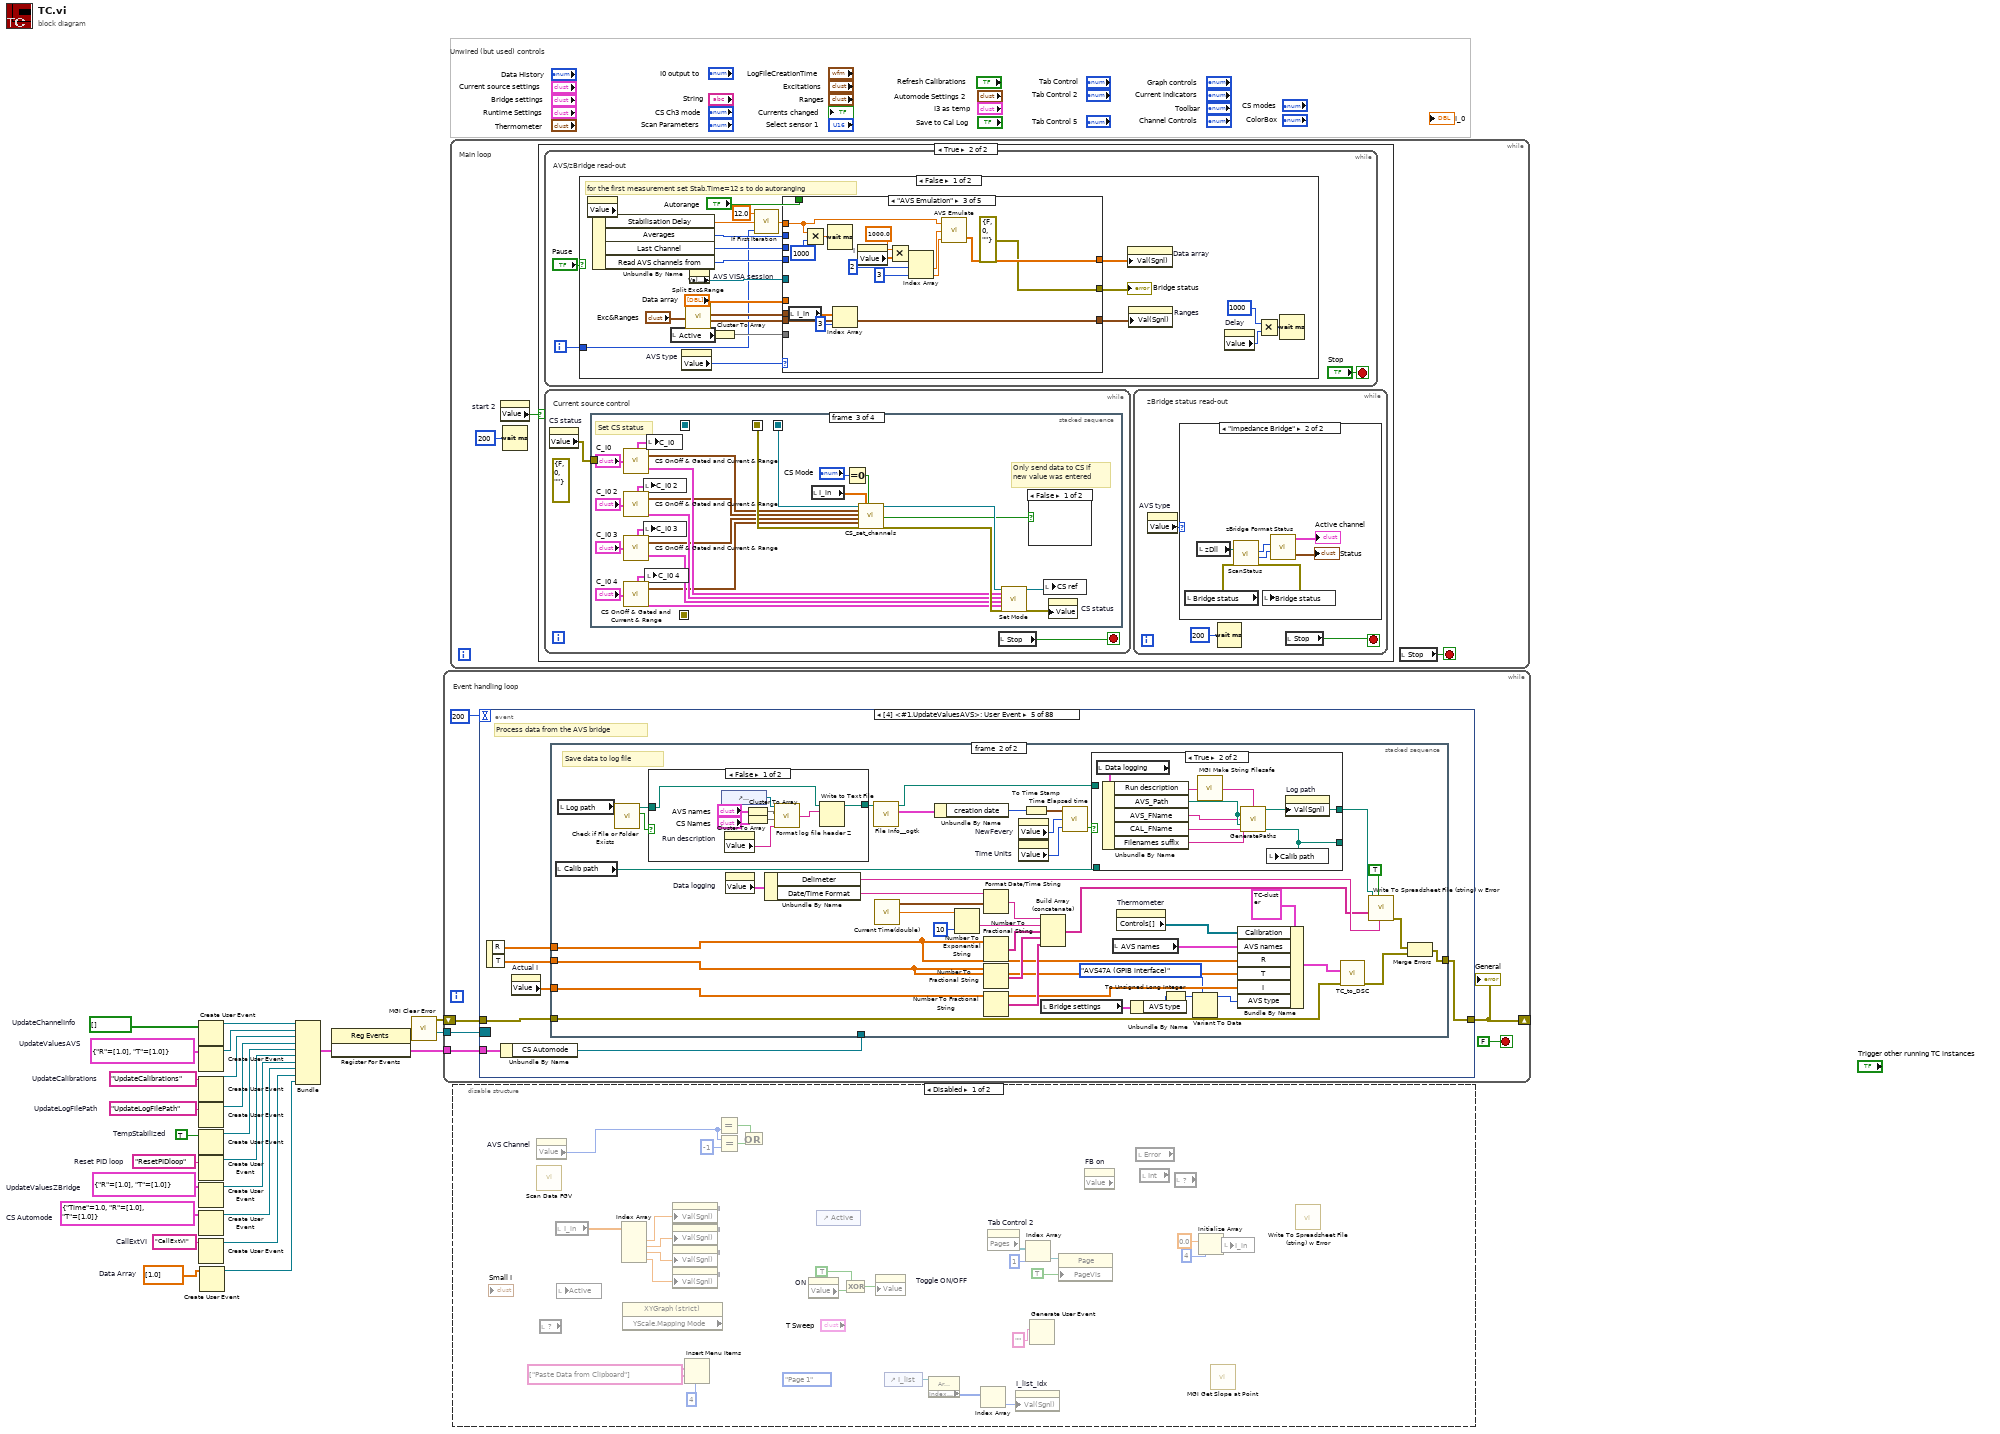
[diagram p0: block diagram]
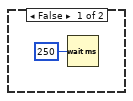
[diagram p3: hidden frame]
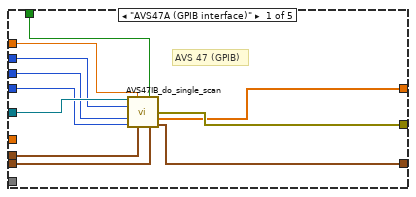
[diagram p5: hidden frame]
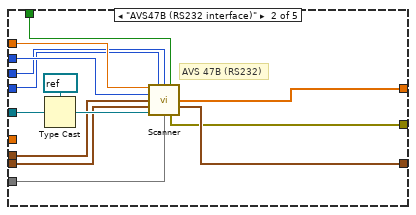
[diagram p6: hidden frame]
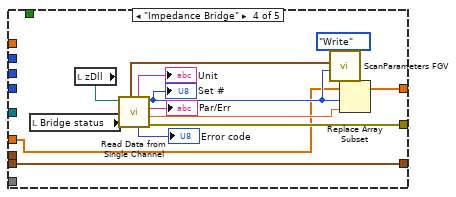
[diagram p7: hidden frame]
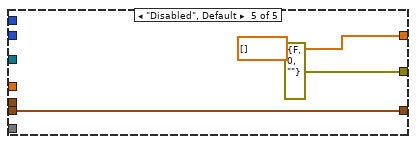
[diagram p8: hidden frame]
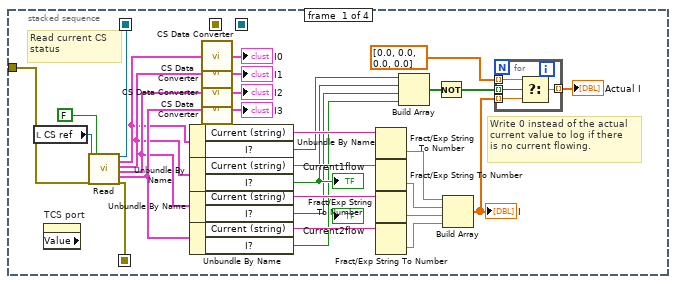
[diagram p10: hidden frame]
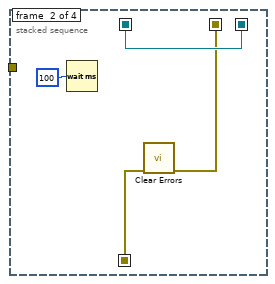
[diagram p11: hidden frame]
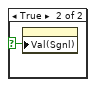
[diagram p12: hidden frame]
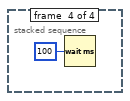
[diagram p13: hidden frame]
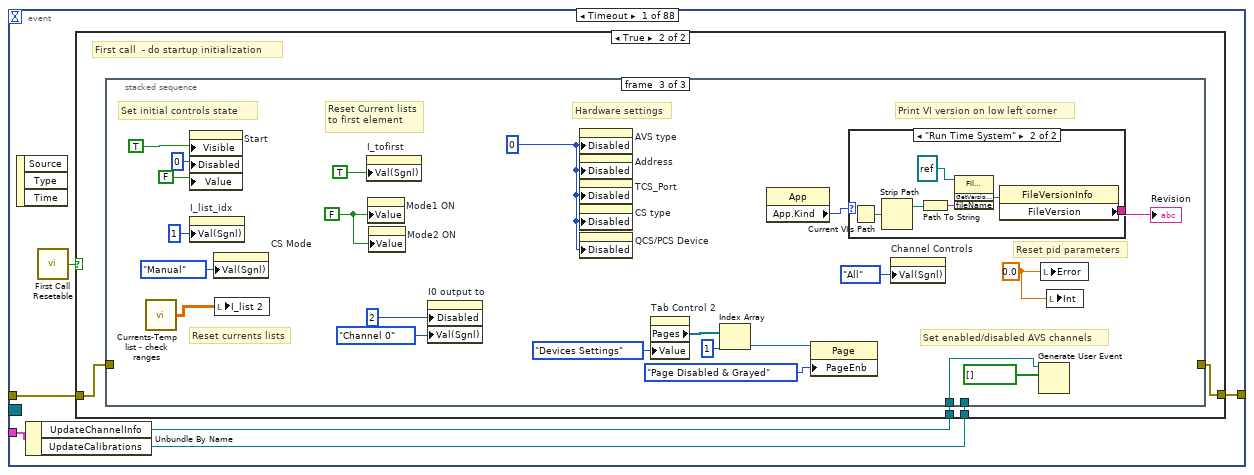
[diagram p14: hidden frame]
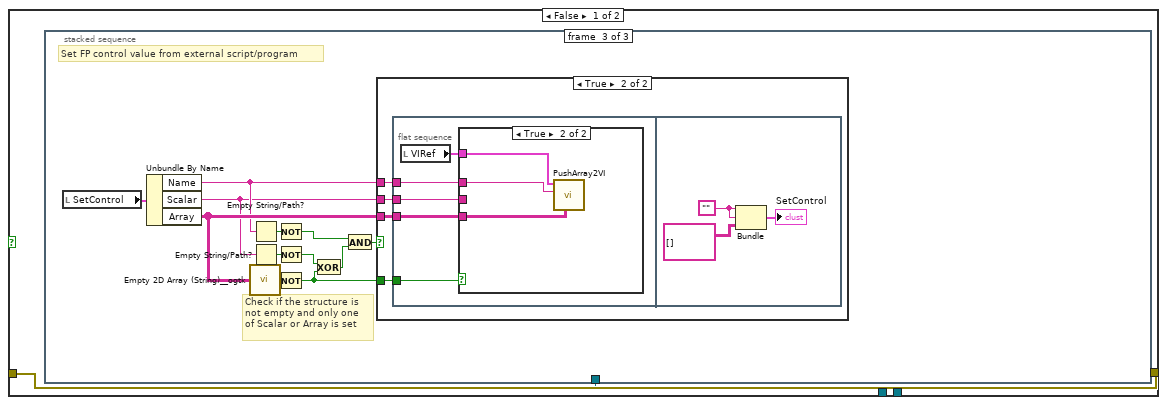
[diagram p15: hidden frame]
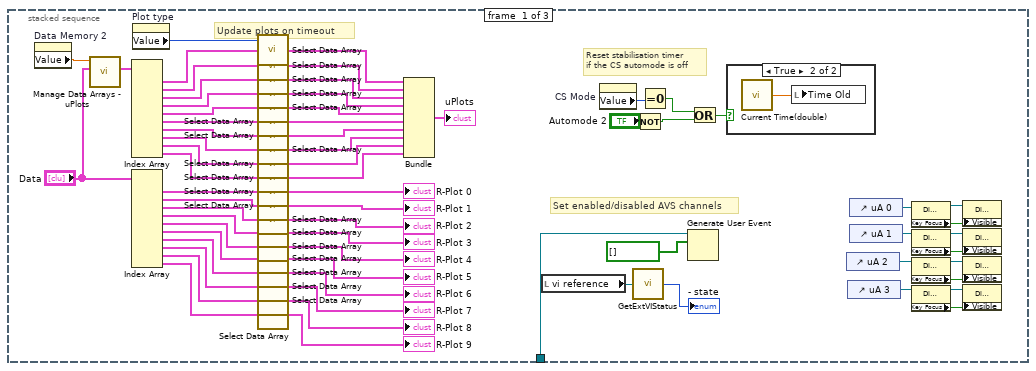
[diagram p16: hidden frame]
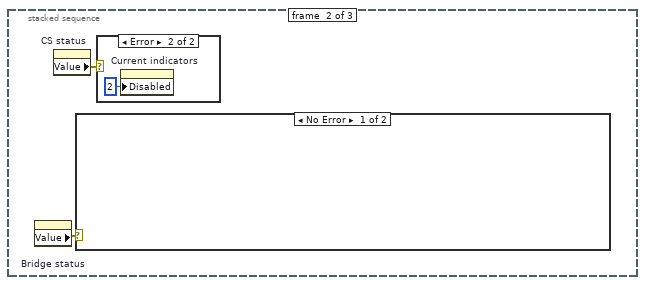
[diagram p18: hidden frame]
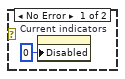
[diagram p19: hidden frame]
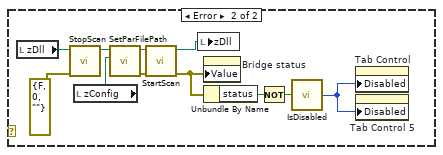
[diagram p20: hidden frame]
diagram:
  w1 = dbl[] [1.0]  # Data Array
  w15 = "CallExtVI"  # CallExtVI
  w16 = bool[] []  # UpdateChannelInfo
  w17 = cluster{"Time":dbl, "R":dbl[], "T":dbl[]} {"Time"=1.0, "R"=[1.0], "T"=[1.0]}  # CS Automode
  w18 = cluster{"R":dbl[], "T":dbl[]} {"R"=[1.0], "T"=[1.0]}  # UpdateValuesAVS
  w19 = cluster{"R":dbl[], "T":dbl[]} {"R"=[1.0], "T"=[1.0]}  # UpdateValuesZBridge
  w20 = "ResetPIDloop"  # Reset PID loop
  w21 = TRUE  # TempStabilized
  w22 = "UpdateLogFilePath"  # UpdateLogFilePath
  w23 = "UpdateCalibrations"  # UpdateCalibrations
  # "Unwired (but used) controls"
  n1 = Create User Event(user event datatype=w16) -> (user event=w13:refnum<user-event>)  [unwired: 1 in, 1 out]
  n2 = Create User Event(user event datatype=w18) -> (user event=w12:refnum<user-event>)  [unwired: 1 in, 1 out]
  n3 = Create User Event(user event datatype=w23) -> (user event=w11:refnum<user-event>)  [unwired: 1 in, 1 out]
  n4 = Create User Event(user event datatype=w22) -> (user event=w10:refnum<user-event>)  [unwired: 1 in, 1 out]
  n5 = Create User Event ("TempStabilized")(user event datatype=w21) -> (user event=w9:refnum<user-event>)  [unwired: 1 in, 1 out]
  n6 = Create User Event(user event datatype=w20) -> (user event=w8:refnum<user-event>)  [unwired: 1 in, 1 out]
  n7 = Create User Event(user event datatype=w19) -> (user event=w7:refnum<user-event>)  [unwired: 1 in, 1 out]
  n8 = Create User Event(user event datatype=w17) -> (user event=w6:refnum<user-event>)  [unwired: 1 in, 1 out]
  n9 = Create User Event(user event datatype=w15) -> (user event=w5:refnum<user-event>)  [unwired: 1 in, 1 out]
  n10 = Create User Event(user event datatype=w1) -> (user event=w2:refnum<user-event>)  [unwired: 1 in, 1 out]
  n11 = Bundle("UpdateChannelInfo"=w13, "UpdateValuesAVS"=w12, "UpdateCalibrations"=w11, "UpdateLogFilePath"=w10, "TempStabilized"=w9, "Reset PID loop"=w8, "UpdateValuesZBridge"=w7, "CS Automode"=w6, "CallExtVI"=w5, "Data Array"=w2) -> (w4:T48)  [unwired: 1 in]
  n12 = register-events(w4) -> (reference out=w14:refnum<event-registration>)  [unwired: 2 in, 1 out]
  n13 = call "MGI Clear Error.vi"() -> ("Error Out"=w3:errorcluster)  [unwired: 7 in]
  n14 = while {
    tunnel: w14 -> [w28]
    shift-right: [w25] -> _
    shift-left: w3 -> [w26]
    tunnel: w4 -> [w24]
    stop <- FALSE stop-if-true
    # "Event handling loop"
    n15 = event shown="[4] <#1.UpdateValuesAVS>: User Event" {
      selector: w28 -> [_ _ _ _ _ _ _ _ _ _ _ _ _ _ _ _ _ _ _ _ _ _ _ _ _ _ _ _ _ _ _ _ _ _ _ _ _ _ _ _ _ _ _ _ _ _ _ _ _ _ _ _ _ _ _ _ _ _ _ _ _ _ _ _ _ _ _ _ _ _ _ _ _ _ _ _ _ _ _ _ _ _ _ _ _ _ _ _]
      dyn-events: _ -> [_ _ _ _ _ _ _ _ _ _ _ _ _ _ _ _ _ _ _ _ _ _ _ _ _ _ _ _ _ _ _ _ _ _ _ _ _ _ _ _ _ _ _ _ _ _ _ _ _ _ _ _ _ _ _ _ _ _ _ _ _ _ _ _ _ _ _ _ _ _ _ _ _ _ _ _ _ _ _ _ _ _ _ _ _ _ _ _]
      timeout: 200 -> [_ _ _ _ _ _ _ _ _ _ _ _ _ _ _ _ _ _ _ _ _ _ _ _ _ _ _ _ _ _ _ _ _ _ _ _ _ _ _ _ _ _ _ _ _ _ _ _ _ _ _ _ _ _ _ _ _ _ _ _ _ _ _ _ _ _ _ _ _ _ _ _ _ _ _ _ _ _ _ _ _ _ _ _ _ _ _ _]
      tunnel: w26 -> [w35 _ _ w444 w492 w574 _ _ w772 _ _ w869 w877 _ _ _ _ _ _ _ _ _ w1115 _ w1122 _ _ _ _ _ _ _ _ _ w1221 _ _ _ _ _ _ _ _ _ _ _ _ _ _ _ _ _ _ _ _ _ _ _ _ _ _ _ w1663 w1682 _ _ _ _ _ w1815 _ _ _ _ _ _ _ _ _ _ _ _ _ _ _ _ _ _]
      tunnel: [w34 _ _ w447 w491 w569 _ _ w770 _ _ w868 w877 _ _ _ _ _ _ _ _ _ w1115 _ w1122 _ _ _ _ _ _ _ _ _ w1221 _ _ _ _ _ _ _ _ _ _ _ _ _ _ _ _ _ _ _ _ _ _ _ _ _ _ _ w1662 w1681 _ _ _ _ _ w1815 _ _ _ _ _ _ _ _ _ _ _ _ _ _ _ _ _ _] -> w25
      tunnel: w24 -> [w32 _ _ w429 w487 w571 w666 w752 _ _ _ _ _ _ _ _ _ _ _ _ _ _ _ _ _ w1152 w1173 _ _ _ _ _ w1209 _ w1219 _ w1252 _ _ _ _ _ w1350 _ _ _ _ _ _ _ _ _ w1529 _ _ _ _ _ _ _ _ _ _ w1676 _ w1753 w1766 _ _ _ w1817 _ _ _ _ _ _ _ _ _ _ _ w1887 _ _ _ _ _]
      event Timeout {
        n16 = event-data() -> ()  [unwired: 1 in, 3 out]
        n17 = Unbundle By Name(w32) -> ("UpdateChannelInfo"=w30:refnum<user-event>, "UpdateCalibrations"=w31:refnum<user-event>)
        n18 = call "First Call Resetable.vi"() -> ("First Call?"=w33:bool)
        n19 = case shown="True" w33 {
          tunnel: w35 -> [w37 w153]
          tunnel: [w37 w151] -> w34
          tunnel: w31 -> [_ w152]
          tunnel: w30 -> [w36 w150]
          frame False {
            n20 = stacked-sequence {
              tunnel: w36 -> [w38 _ _]
              frame #0 {
                # "Update plots on timeout"
                # "Set enabled/disabled AVS channels"
                # "Reset stabilisation timer\nif the CS automode is off"
                n21 = property on="Data Memory 2" class="DigNum (strict)"() -> ("Value"=w99:dbl)  [unwired: 2 in, 2 out]
                n22 = call "Manage Data Arrays - uPlots.vi"("Data In"="Data", "Data Memory"=w99) -> ("Data Out"=w54:T28)  [unwired: 7 in]
                n23 = Index Array(array=w54) -> (element #1=w69:cluster{"R":dbl[], "T":dbl[], "Time":dbl[]}, element #2=w70:cluster{"R":dbl[], "T":dbl[], "Time":dbl[]}, element #3=w71:cluster{"R":dbl[], "T":dbl[], "Time":dbl[]}, element #4=w72:cluster{"R":dbl[], "T":dbl[], "Time":dbl[]}, element #5=w73:cluster{"R":dbl[], "T":dbl[], "Time":dbl[]}, element #6=w74:cluster{"R":dbl[], "T":dbl[], "Time":dbl[]}, element #7=w75:cluster{"R":dbl[], "T":dbl[], "Time":dbl[]}, element #8=w76:cluster{"R":dbl[], "T":dbl[], "Time":dbl[]}, element #9=w77:cluster{"R":dbl[], "T":dbl[], "Time":dbl[]}, element #10=w78:cluster{"R":dbl[], "T":dbl[], "Time":dbl[]})  [unwired: 10 in]
                n24 = Index Array(array="Data") -> (element #1=w98:cluster{"R":dbl[], "T":dbl[], "Time":dbl[]}, element #2=w97:cluster{"R":dbl[], "T":dbl[], "Time":dbl[]}, element #3=w96:cluster{"R":dbl[], "T":dbl[], "Time":dbl[]}, element #4=w95:cluster{"R":dbl[], "T":dbl[], "Time":dbl[]}, element #5=w94:cluster{"R":dbl[], "T":dbl[], "Time":dbl[]}, element #6=w93:cluster{"R":dbl[], "T":dbl[], "Time":dbl[]}, element #7=w92:cluster{"R":dbl[], "T":dbl[], "Time":dbl[]}, element #8=w91:cluster{"R":dbl[], "T":dbl[], "Time":dbl[]}, element #9=w90:cluster{"R":dbl[], "T":dbl[], "Time":dbl[]}, element #10=w89:cluster{"R":dbl[], "T":dbl[], "Time":dbl[]})  [unwired: 10 in]
                n25 = property on="Plot type" class="Enum (strict)"() -> ("Value"=w57:enum16{"R vs Time", "T vs Time"})  [unwired: 2 in, 2 out]
                n26 = call "Select Data Array.vi"("Cluster 2"=w69, "Value"=w57) -> ("Cluster"=w79:cluster{"Time":dbl[], "T":dbl[]})
                n27 = call "Select Data Array.vi"("Cluster 2"=w70, "Value"=w57) -> ("Cluster"=w80:cluster{"Time":dbl[], "T":dbl[]})
                n28 = call "Select Data Array.vi"("Cluster 2"=w71, "Value"=w57) -> ("Cluster"=w81:cluster{"Time":dbl[], "T":dbl[]})
                n29 = call "Select Data Array.vi"("Cluster 2"=w72, "Value"=w57) -> ("Cluster"=w82:cluster{"Time":dbl[], "T":dbl[]})
                n30 = call "Select Data Array.vi"("Cluster 2"=w73, "Value"=w57) -> ("Cluster"=w88:cluster{"Time":dbl[], "T":dbl[]})
                n31 = call "Select Data Array.vi"("Cluster 2"=w74, "Value"=w57) -> ("Cluster"=w83:cluster{"Time":dbl[], "T":dbl[]})
                n32 = call "Select Data Array.vi"("Cluster 2"=w75, "Value"=w57) -> ("Cluster"=w84:cluster{"Time":dbl[], "T":dbl[]})
                n33 = call "Select Data Array.vi"("Cluster 2"=w76, "Value"=w57) -> ("Cluster"=w85:cluster{"Time":dbl[], "T":dbl[]})
                n34 = call "Select Data Array.vi"("Cluster 2"=w77, "Value"=w57) -> ("Cluster"=w86:cluster{"Time":dbl[], "T":dbl[]})
                n35 = call "Select Data Array.vi"("Cluster 2"=w78, "Value"=w57) -> ("Cluster"=w87:cluster{"Time":dbl[], "T":dbl[]})
                n36 = call "Select Data Array.vi"("Cluster 2"=w98, "Value"=w57) -> ("Cluster"=→"R-Plot 0":cluster{"Time":dbl[], "T":dbl[]})
                n37 = call "Select Data Array.vi"("Cluster 2"=w97, "Value"=w57) -> ("Cluster"=→"R-Plot 1":cluster{"Time":dbl[], "T":dbl[]})
                n38 = call "Select Data Array.vi"("Cluster 2"=w96, "Value"=w57) -> ("Cluster"=→"R-Plot 2":cluster{"Time":dbl[], "T":dbl[]})
                n39 = call "Select Data Array.vi"("Cluster 2"=w95, "Value"=w57) -> ("Cluster"=→"R-Plot 3":cluster{"Time":dbl[], "T":dbl[]})
                n40 = call "Select Data Array.vi"("Cluster 2"=w94, "Value"=w57) -> ("Cluster"=→"R-Plot 4":cluster{"Time":dbl[], "T":dbl[]})
                n41 = call "Select Data Array.vi"("Cluster 2"=w93, "Value"=w57) -> ("Cluster"=→"R-Plot 5":cluster{"Time":dbl[], "T":dbl[]})
                n42 = call "Select Data Array.vi"("Cluster 2"=w92, "Value"=w57) -> ("Cluster"=→"R-Plot 6":cluster{"Time":dbl[], "T":dbl[]})
                n43 = call "Select Data Array.vi"("Cluster 2"=w91, "Value"=w57) -> ("Cluster"=→"R-Plot 7":cluster{"Time":dbl[], "T":dbl[]})
                n44 = call "Select Data Array.vi"("Cluster 2"=w90, "Value"=w57) -> ("Cluster"=→"R-Plot 8":cluster{"Time":dbl[], "T":dbl[]})
                n45 = call "Select Data Array.vi"("Cluster 2"=w89, "Value"=w57) -> ("Cluster"=→"R-Plot 9":cluster{"Time":dbl[], "T":dbl[]})
                n46 = Bundle("Cluster"=w79, "Cluster"=w80, "Cluster"=w81, "Cluster"=w82, "Cluster"=w88, "Cluster"=w83, "Cluster"=w84, "Cluster"=w85, "Cluster"=w86, "Cluster"=w87) -> (→"uPlots":T57)  [unwired: 1 in]
                n47 = local read "vi reference"() -> (w53:refnum<vi>)
                n48 = property on="CS Mode" class="Enum (strict)"() -> ("Value"=w102:T39)  [unwired: 2 in, 2 out]
                n49 = call "GetExtVIStatus.vi"("vi reference in"=w53) -> ("Exec.State"=→"- state":T46)  [unwired: 2 out]
                n50 = Not(x="Automode 2") -> (.not. x?=w101:bool)
                n51 = Equal To 0?(x=w102) -> (x = 0?=w51:bool)
                n52 = Generate User Event(user event=w38, event data cluster=bool[] [] ("event data")) -> ()  [unwired: 2 in, 2 out]
                n53 = Or(x=w51, y=w101) -> (x .or. y?=w100:bool)
                n54 = case shown="True" w100 {
                  frame False {
                  }
                  frame True {
                    n55 = call "Current Time(double).vi"() -> ("Current Time (double)"=w104:dbl)  [unwired: 6 in, 1 out]
                    n56 = local write "Time Old"(w104) -> ()
                  }
                }
                n57 = control-ref of="uA 2"() -> (w39:refnum<vi>)
                n58 = control-ref of="uA 3"() -> (w40:refnum<vi>)
                n59 = control-ref of="uA 0"() -> (w50:refnum<vi>)
                n60 = control-ref of="uA 1"() -> (w46:refnum<vi>)
                n61 = property class="DigNum (strict)"(reference=w50) -> (reference out=w49:refnum<vi>, "Key Focus"=w48:bool)  [unwired: 1 in, 1 out]
                n62 = property class="DigNum (strict)"(reference=w46) -> (reference out=w47:refnum<vi>, "Key Focus"=w45:bool)  [unwired: 1 in, 1 out]
                n63 = property class="DigNum (strict)"(reference=w39) -> (reference out=w41:refnum<vi>, "Key Focus"=w42:bool)  [unwired: 1 in, 1 out]
                n64 = property class="DigNum (strict)"(reference=w40) -> (reference out=w43:refnum<vi>, "Key Focus"=w44:bool)  [unwired: 1 in, 1 out]
                n65 = property class="DigNum (strict)"(reference=w49, "Visible"=w48) -> ()  [unwired: 1 in, 2 out]
                n66 = property class="DigNum (strict)"(reference=w47, "Visible"=w45) -> ()  [unwired: 1 in, 2 out]
                n67 = property class="DigNum (strict)"(reference=w41, "Visible"=w42) -> ()  [unwired: 1 in, 2 out]
                n68 = property class="DigNum (strict)"(reference=w43, "Visible"=w44) -> ()  [unwired: 1 in, 2 out]
              }
              frame #1 {
                n69 = property on="Bridge status" class="Clust (strict)"() -> ("Value"=w106:errorcluster)  [unwired: 2 in, 2 out]
                n70 = property on="CS status" class="Clust (strict)"() -> ("Value"=w105:errorcluster)  [unwired: 2 in, 2 out]
                n71 = case shown="No Error" w106 {
                  frame No Error {
                  }
                  frame Error {
                    n72 = local read "zDll"() -> (w119:path)
                    n73 = call "StopScan.vi"("error in (no error)"=errorcluster {"status"=FALSE, "code"=0, "source"=""}, "path in"=w119) -> ("path out"=w115:path)  [unwired: 8 in, 1 out]
                    n74 = local read "zConfig"() -> (w118:path)
                    n75 = call "SetParFilePath.vi"("path"=w118, "zDll"=w115) -> ("error out"=w117:errorcluster, "zDll out"=w116:path)  [unwired: 8 in]
                    n76 = call "StartScan.vi"("error in (no error)"=w117, "path in"=w116) -> ("error out"=w112:errorcluster, "path out"=w113:path)  [unwired: 8 in]
                    n77 = local write "zDll"(w113) -> ()
                    n78 = property on="Bridge status" class="Clust (strict)"("Value"=w112) -> ()  [unwired: 2 in, 2 out]
                    n79 = Unbundle By Name(w112) -> ("status"=w110:bool)
                    n80 = Not(x=w110) -> (.not. x?=w111:bool)
                    n81 = call "IsDisabled.vi"("Enabled?"=w111) -> ("Numeric"=w109:i16)
                    n82 = property on="Tab Control" class="TabCtl (strict)"("Disabled"=w109) -> ()  [unwired: 2 in, 2 out]
                    n83 = property on="Tab Control 5" class="TabCtl (strict)"("Disabled"=w109) -> ()  [unwired: 2 in, 2 out]
                  }
                }
                n84 = case shown="Error" w105 {
                  frame No Error {
                    n85 = property on="Current indicators" class="TabCtl (strict)"("Disabled"=u8 0) -> ()  [unwired: 2 in, 2 out]
                  }
                  frame Error {
                    n86 = property on="Current indicators" class="TabCtl (strict)"("Disabled"=u8 2) -> ()  [unwired: 2 in, 2 out]
                  }
                }
              }
              frame #2 {
                # "Check if the structure is \nnot empty and only one\nof Scalar or Array is set"
                # "Set FP control value from external script/program"
                n87 = local read "SetControl"() -> (w120:T1)
                n88 = Unbundle By Name(w120) -> ("Name"=w122:string, "Scalar"=w121:string, "Array"=w130:string[][])
                n89 = call "Empty 2D Array (String)__ogtk.vi"("Array"=w130) -> ("Empty Array?"=w127:bool)  [unwired: 8 in]
                n90 = Empty String/Path?(string/path=w122) -> (empty?=w126:bool)
                n91 = Empty String/Path?(string/path=w121) -> (empty?=w125:bool)
                n92 = Not(x=w126) -> (.not. x?=w124:bool)
                n93 = Not(x=w125) -> (.not. x?=w128:bool)
                n94 = Not(x=w127) -> (.not. x?=w131:bool)
                n95 = Exclusive Or(1:w131, 2:w128) -> (0:w129:bool)
                n96 = And(x=w124, y=w129) -> (x .and. y?=w123:bool)
                n97 = case shown="True" w123 {
                  tunnel: w122 -> [_ w135]
                  tunnel: w121 -> [_ w134]
                  tunnel: w130 -> [_ w133]
                  tunnel: w131 -> [_ w132]
                  frame False {
                  }
                  frame True {
                    n98 = flat-sequence {
                      tunnel: w135 -> [w139]
                      tunnel: w134 -> [w138]
                      tunnel: w133 -> [w136]
                      tunnel: w132 -> [w137]
                      frame #0 {
                        n99 = local read "VIRef"() -> (w140:T2)
                        n100 = case shown="True" w137 {
                          tunnel: w140 -> [w143 w146]
                          tunnel: w139 -> [w142 w145]
                          tunnel: w138 -> [w141 _]
                          tunnel: w136 -> [_ w144]
                          frame False {
                            n101 = call "Push2VI.vi"("New Value"=w141, "element"=w142, "VIRef"=w143) -> ()  [unwired: 8 in, 1 out]
                          }
                          frame True {
                            n102 = call "PushArray2VI.vi"("Str"=w144, "element"=w145, "VIRef"=w146) -> ()  [unwired: 8 in, 1 out]
                          }
                        }
                      }
                      frame #1 {
                        w148 = ""
                        n103 = Bundle(w148, w148, "Array"=string[][] []) -> (→"SetControl":cluster{string, string, "Array":string[][]})  [unwired: 1 in]
                      }
                    }
                  }
                }
              }
            }
          }
          frame True {
            # "First call  - do startup initialization"
            n104 = stacked-sequence {
              tunnel: w153 -> [_ w179 _]
              tunnel: [_ w170 _] -> w151
              tunnel: w152 -> [_ w169 _]
              tunnel: w150 -> [_ _ w233]
              frame #0 {
                w154 = u8 0 ("Disabled")
                n105 = property on="Tab Control 5" class="TabCtl (strict)"("Disabled"=w154) -> ()  [unwired: 2 in, 2 out]
                n106 = property on="Tab Control" class="TabCtl (strict)"("Disabled"=w154) -> ()  [unwired: 2 in, 2 out]
                n107 = property on="Current indicators" class="TabCtl (strict)"("Disabled"=w154) -> ()  [unwired: 2 in, 2 out]
                n108 = property on="Tab Control 2" class="TabCtl (strict)"("Disabled"=w154) -> ()  [unwired: 2 in, 2 out]
                n109 = property on="Toolbar" class="TabCtl (strict)"("Disabled"=w154) -> ()  [unwired: 2 in, 2 out]
                n110 = call "Current VIs Reference__ogtk.vi"() -> ("Current VI's reference"=w157:refnum<vi>)  [unwired: 5 in]
                n111 = call "Current VIs Parent Directory__ogtk.vi"("Relative path (.)"=path "Calibrations" ("Library Path")) -> ("Parent Directory (+ Relative)"=w162:path)  [unwired: 4 in]
                n112 = call "Current VIs Parent Directory__ogtk.vi"("Relative path (.)"=path "data/Temp Control.lvlib" ("Library Path")) -> ("Parent Directory (+ Relative)"=w164:path)  [unwired: 4 in]
                n113 = call "Current VIs Parent Directory__ogtk.vi"("Relative path (.)"=path "data/ImpBridgeDll.dll" ("Library Path")) -> ("Parent Directory (+ Relative)"=→"zDll":path)  [unwired: 4 in]
                n114 = call "Current VIs Parent Directory__ogtk.vi"("Relative path (.)"=path "data" ("Library Path")) -> ("Parent Directory (+ Relative)"=→"zConfig":path)  [unwired: 4 in]
                n115 = call "GetFrontPanelControls.vi"("Ref to VI"=w157) -> ("VIRef"=w156:T2)  [unwired: 9 in, 1 out]
                "VIRef" <- w156
                n116 = property on="AVS_CalFolder" class="Path"("Value"=w162) -> ()  [unwired: 2 in, 2 out]
                n117 = invoke class="App" method="Library.Deploy Library"("libPath"=w164) -> ()  [unwired: 4 in, 5 out]
                n118 = Unbundle By Name(w156) -> ("Full Name"=→"ControlNames":string[])
                n119 = property on="String" class="Str"("Visible"=FALSE) -> ()  [unwired: 2 in, 2 out]
                n120 = property on="I_0" class="DigNum (strict)"("Value"=0.0 ("I3")) -> ()  [unwired: 2 in, 2 out]
                n121 = disable-structure shown="Enabled" {
                  frame Enabled {
                    n122 = property on="Minimize" class="Bool (strict)"("Val(Sgnl)"=FALSE ("Value (Signaling)")) -> ()  [unwired: 2 in, 2 out]
                  }
                  frame Disabled {
                  }
                }
              }
              frame #1 {
                # "Read settings from registry"
                n123 = flat-sequence {
                  tunnel: [w193] -> w178
                  tunnel: w179 -> [w192]
                  tunnel: [w190] -> w177
                  tunnel: w178 -> [w199]
                  tunnel: [w199] -> w176
                  tunnel: [w197] -> w175
                  tunnel: w177 -> [w197]
                  tunnel: [w204] -> w174
                  tunnel: w176 -> [w203]
                  tunnel: [w201] -> w173
                  tunnel: w175 -> [w201]
                  tunnel: w174 -> [w210]
                  tunnel: [w210] -> w172
                  tunnel: [w208] -> w171
                  tunnel: w173 -> [w208]
                  tunnel: w172 -> [w214]
                  tunnel: [w213] -> w170
                  tunnel: w171 -> [w212]
                  tunnel: w169 -> [w211]
                  frame #0 {
                    n124 = call "Current VIs Parent Directory__ogtk.vi"("Relative path (.)"=path "data/config.ini") -> ("Parent Directory (+ Relative)"=w190:path)  [unwired: 4 in]
                    n125 = control-ref of="Active"() -> (w182:refnum<vi>)
                    n126 = control-ref of="Automode Settings 2"() -> (w180:refnum<vi>)
                    n127 = control-ref of="Current source settings"() -> (w183:refnum<vi>)
                    n128 = control-ref of="Bridge settings"() -> (w194:refnum<vi>)
                    n129 = control-ref of="Runtime Settings"() -> (w189:refnum<vi>)
                    n130 = control-ref of="I3 as temp"() -> (w181:refnum<vi>)
                    n131 = control-ref of="Data logging"() -> (w188:refnum<vi>)
                    n132 = control-ref of="PID setup"() -> (w187:refnum<vi>)
                    n133 = control-ref of="CS Names"() -> (w186:refnum<vi>)
                    n134 = control-ref of="CurCalibrations"() -> (w184:refnum<vi>)
                    n135 = control-ref of="AVS names"() -> (w185:refnum<vi>)
                    n136 = Build Array(w182, w183, w194, w189, w188, w187, w186, w185, w184, w181, w180) -> (w196:refnum<vi>[])
                    n137 = call "Save Load Settings to File by Ref with path.vi"("Array of Cluster References"=w196, "Action"=enum8{"Load", "Save"}."Load", "error in (no error)"=w192, "configuration file path"=w190) -> ("error out"=w193:errorcluster)  [unwired: 5 in]
                  }
                  frame #1 {
                    n138 = Wait (ms)(milliseconds to wait=250) -> ()  [unwired: 1 out]
                  }
                  frame #2 {
                    n139 = control-ref of="Thermometer"() -> (w202:refnum<vi>)
                    n140 = control-ref of="CurCalibrations"() -> (w200:refnum<vi>)
                    n141 = control-ref of="CurCalibrations"() -> ()  [unwired: 1 out]
                    n142 = control-ref of="AVS_CalFolder"() -> (w206:refnum<vi>)
                    n143 = control-ref of="Select sensor 1"() -> (w207:refnum<vi>)
                    n144 = control-ref of="Select sensor 1"() -> (w205:refnum<vi>)
                    n145 = call "ReloadCalibrations.vi"("error in (no error)"=w203, "Quick convert sensors"=w205, "CurCalibrations"=w200, "Calibration files path"=w206, "Channel1 sensors"=w207, "Channels list"=w202) -> ("error out"=w204:errorcluster)  [unwired: 1 in]
                  }
                  frame #3 {
                    n146 = Wait (ms)(milliseconds to wait=250) -> ()  [unwired: 1 out]
                  }
                  frame #4 {
                    n147 = disable-structure shown="Disabled" {
                      disable-tunnel: w214 -> [w217 w222]
                      disable-tunnel: [w216 w224] -> w213
                      disable-tunnel: w212 -> [w215 _]
                      disable-tunnel: w211 -> [_ w221]
                      frame Disabled {
                        (unwired) "SOFTWARE\\Leiden Cryogenics\\TC" ("subkey 2")
                        (unwired) T58."HKEY_CURRENT_USER" ("root key (HKEY_LOCAL_MACHINE) 2")
                        n148 = control-ref of="Thermometer"() -> (w219:refnum<vi>)
                        n149 = Build Array(w219) -> (w218:refnum<vi>[])
                        n150 = call "Save Load Settings to File by Ref with path.vi"("Array of Cluster References"=w218, "Action"=enum8{"Load", "Save"}."Load", "error in (no error)"=w217, "configuration file path"=w215) -> ("error out"=w216:errorcluster)  [unwired: 5 in]
                      }
                      frame Enabled {
                        n151 = Generate User Event(user event=w221, event data cluster="" ("event data"), error in=w222) -> (error out=w224:errorcluster)  [unwired: 1 in, 1 out]
                      }
                    }
                  }
                }
              }
              frame #2 {
                w225 = FALSE ("Mode1 ON")
                w235 = 0.0 ("T_error")
                w243 = u8 0 ("Disabled")
                # "Set enabled/disabled AVS channels"
                # "Reset pid parameters"
                # "Print VI version on low left corner"
                # "Reset Current lists\nto first element"
                # "Hardware settings"
                # "Reset currents lists"
                # "Set initial controls state"
                n152 = call "Currents-Temp list - check ranges.vi"() -> ("I_list out"=w236:dbl[][])  [unwired: 5 in]
                n153 = property on="Start" class="Bool (strict)"("Visible"=TRUE, "Disabled"=u8 0, "Value"=FALSE ("start")) -> ()  [unwired: 2 in, 2 out]
                n154 = property on="I_list_idx" class="DigNum (strict)"("Val(Sgnl)"=1 ("Value (Signaling)")) -> ()  [unwired: 2 in, 2 out]
                n155 = property on="CS Mode" class="Enum (strict)"("Val(Sgnl)"=CS_mode."Manual" ("CS Mode")) -> ()  [unwired: 2 in, 2 out]
                n156 = local write "I_list 2"(w236) -> ()
                n157 = property on="I_tofirst" class="Bool (strict)"("Val(Sgnl)"=TRUE ("Value (Signaling)")) -> ()  [unwired: 2 in, 2 out]
                n158 = property on="Mode1 ON" class="Bool (strict)"("Value"=w225) -> ()  [unwired: 2 in, 2 out]
                n159 = property on="Mode2 ON" class="Bool (strict)"("Value"=w225) -> ()  [unwired: 2 in, 2 out]
                n160 = property on="I0 output to" class="Enum (strict)"("Disabled"=u8 2, "Val(Sgnl)"=T38."Channel 0" ("Map Channel 0 to")) -> ()  [unwired: 2 in, 2 out]
                n161 = property on="AVS type" class="Enum (strict)"("Disabled"=w243) -> ()  [unwired: 2 in, 2 out]
                n162 = property on="Address" class="VISAName"("Disabled"=w243) -> ()  [unwired: 2 in, 2 out]
                n163 = property on="TCS_Port" class="VISAName"("Disabled"=w243) -> ()  [unwired: 2 in, 2 out]
                n164 = property on="CS type" class="Enum (strict)"("Disabled"=w243) -> ()  [unwired: 2 in, 2 out]
                n165 = property on="QCS/PCS Device" class="DigNum (strict)"("Disabled"=w243) -> ()  [unwired: 2 in, 2 out]
                n166 = property on="Tab Control 2" class="TabCtl (strict)"("Value"=T34."Devices Settings" ("Tab Control 2")) -> ("Pages"=w230:refnum<vi>[])  [unwired: 2 in, 2 out]
                n167 = Index Array(array=w230, index=1) -> (element=w227:refnum<vi>)
                n168 = property class="App"() -> ("App.Kind"=w239:T59)  [unwired: 2 in, 2 out]
                n169 = property class="Page"(reference=w227, "PageEnb"=T49."Page Disabled & Grayed" ("Page Enabled State")) -> ()  [unwired: 1 in, 2 out]
                n170 = case shown="\"Run Time System\"" w239 {
                  tunnel: [w248 w259] -> w240
                  frame "invalid app kind", Default {
                    n171 = control-ref of="This VI"() -> (w255:refnum<vi>)
                    n172 = property class="VI"(reference=w255) -> ("Hist.Revision"=w254:u32)  [unwired: 1 in, 2 out]
                    n173 = Divide(x=w254, y=1000.0 ("x")) -> (x/y=w250:dbl)
                    n174 = Number To Fractional String(use system decimal point (T)=FALSE, number=w250, precision (6)=i16 2) -> (F-format string=w249:string)  [unwired: 1 in]
                    n175 = Concatenate Strings("" ("string"), w249) -> (w248:string)
                  }
                  frame "Run Time System" {
                    n176 = Current VI's Path() -> (path=w261:path)
                    n177 = Strip Path(path=w261) -> (stripped path=w260:path)  [unwired: 1 out]
                    n178 = Path To String(path=w260) -> (string=w258:string)
                    n179 = invoke class="FileVersionInfo" method="GetVersionInfo"(reference=refnum<k24> refnum (".NET object"), "fileName"=w258) -> ("GetVersionInfo"=w257:refnum<k24>)  [unwired: 2 in, 3 out]
                    n180 = property class="FileVersionInfo"(reference=w257) -> ("FileVersion"=w259:string)  [unwired: 1 in, 2 out]
                  }
                }
                "Revision" <- w240
                n181 = property on="Channel Controls" class="TabCtl (strict)"("Val(Sgnl)"=T8."All" ("Value (Signaling)")) -> ()  [unwired: 2 in, 2 out]
                n182 = Generate User Event(user event=w233, event data cluster=bool[] [] ("event data")) -> ()  [unwired: 2 in, 2 out]
                n183 = local write "Error"(w235) -> ()
                n184 = local write "Int"(w235) -> ()
              }
            }
          }
        }
      }
      event "Start": Value Change {
        # "\"Start\" button clicked -> start measuring"
        n185 = event-data() -> ()  [unwired: 1 in, 6 out]
        n186 = stacked-sequence {
          frame #0 {
            n187 = property on="Run description" class="Str"() -> ("Value"=w264:string)  [unwired: 2 in, 2 out]
            n188 = property on="Ask on start?" class="Bool (strict)"() -> ("Value"=w263:bool)  [unwired: 2 in, 2 out]
            n189 = Not(x=w263) -> (.not. x?=w262:bool)
            n190 = call "Run Reference DLG.vi"("Enable"=w263, "Run Reference"=w264, "Dont' ask again"=w262) -> ("Dont' ask again"=w266:bool, "Run Reference"=w267:string, "OK"=w268:bool)  [unwired: 13 in, 1 out]
            n191 = Not(x=w266) -> (.not. x?=w265:bool)
            n192 = case shown="True" w268 {
              tunnel: w267 -> [_ w270]
              tunnel: w265 -> [_ w269]
              frame False {
              }
              frame True {
                n193 = property on="Run description" class="Str"("Val(Sgnl)"=w270) -> ()  [unwired: 2 in, 2 out]
                n194 = property on="Ask on start?" class="Bool (strict)"("Val(Sgnl)"=w269) -> ()  [unwired: 2 in, 2 out]
              }
            }
          }
          frame #1 {
            (unwired) T58."HKEY_CURRENT_USER" ("root key (HKEY_LOCAL_MACHINE) 2")
            # "Save new settings to config file"
            n195 = control-ref of="Active"() -> (w274:refnum<vi>)
            n196 = control-ref of="I3 as temp"() -> (w273:refnum<vi>)
            n197 = control-ref of="Automode Settings 2"() -> (w272:refnum<vi>)
            n198 = control-ref of="Automode Settings 2"() -> (w271:refnum<vi>)
            n199 = control-ref of="CS Names"() -> (w279:refnum<vi>)
            n200 = control-ref of="AVS names"() -> (w278:refnum<vi>)
            n201 = control-ref of="CurCalibrations"() -> (w275:refnum<vi>)
            n202 = control-ref of="Bridge settings"() -> (w285:refnum<vi>)
            n203 = control-ref of="Runtime Settings"() -> (w286:refnum<vi>)
            n204 = control-ref of="Current source settings"() -> (w284:refnum<vi>)
            n205 = control-ref of="Thermometer"() -> (w287:refnum<vi>)
            n206 = control-ref of="PID setup"() -> (w288:refnum<vi>)
            n207 = control-ref of="Data logging"() -> (w283:refnum<vi>)
            n208 = Build Array(w274, w285, w286, w284, w283, w287, w288, w279, w278, w275, w273, w272, w271) -> (w281:refnum<vi>[])
            n209 = call "Current VIs Parent Directory__ogtk.vi"("Relative path (.)"=path "data/config.ini") -> ("Parent Directory (+ Relative)"=w276:path)  [unwired: 4 in]
            n210 = call "Save Load Settings to File by Ref with path.vi"("Array of Cluster References"=w281, "subkey"="SOFTWARE\\Leiden Cryogenics\\TC" ("subkey 2"), "Action"=enum8{"Load", "Save"}."Save", "configuration file path"=w276) -> ()  [unwired: 5 in, 1 out]
          }
          frame #2 {
            w304 = u8 2 ("Disabled")
            # "Reset stop button"
            # "Hide Disable Start button"
            # "Load external calibration VI"
            # "Set controls\nInitialize data for run"
            # "Lock hardware settings"
            n211 = property on="AVS type" class="Enum (strict)"("Disabled"=w304) -> ()  [unwired: 2 in, 2 out]
            n212 = property on="Address" class="VISAName"("Disabled"=w304) -> ()  [unwired: 2 in, 2 out]
            n213 = property on="AVS_SPort" class="VISAName"("Disabled"=w304) -> ()  [unwired: 2 in, 2 out]
            n214 = property on="TCS_Port" class="VISAName"("Disabled"=w304) -> ()  [unwired: 2 in, 2 out]
            n215 = property on="CS type" class="Enum (strict)"("Disabled"=w304) -> ()  [unwired: 2 in, 2 out]
            n216 = property on="QCS/PCS Device" class="DigNum (strict)"("Disabled"=w304) -> ()  [unwired: 2 in, 2 out]
            n217 = property on="I0 output to" class="Enum (strict)"("Disabled"=u8 0) -> ()  [unwired: 2 in, 2 out]
            n218 = call "Current Time(double).vi"() -> ("Current Time (double)"=w293:dbl)  [unwired: 6 in, 1 out]
            n219 = local write "Time Old"(w293) -> ()
            n220 = property on="External VI path" class="Path"() -> ("Value"=w303:path)  [unwired: 2 in, 2 out]
            n221 = vi-ref "OnTempStabilizedRef.vi"() -> (w302:refnum<vi>)
            n222 = Open VI Reference(type specifier VI Refnum (for type only)=w302, vi path=w303) -> (vi reference=→"vi reference":refnum<vi>)  [unwired: 4 in, 1 out]
            n223 = local write "VI called?"(FALSE ("VI called?")) -> ()
            n224 = property on="Start" class="Bool (strict)"("Visible"=TRUE, "Disabled"=u8 2) -> ()  [unwired: 2 in, 2 out]
            n225 = Initialize Array(cluster{"R":dbl[], "T":dbl[], "Time":dbl[]} {"R"=[], "T"=[], "Time"=[]}, 10 ("dimension size")) -> (w297:cluster{"R":dbl[], "T":dbl[], "Time":dbl[]}[])
            n226 = disable-structure shown="Enabled" {
              frame Enabled {
                n227 = property on="Stop" class="Bool (strict)"("Value"=FALSE ("MainStopButton")) -> ()  [unwired: 2 in, 2 out]
              }
              frame Disabled {
              }
            }
            n228 = local write "Data"(w297) -> ()
            n229 = property on="Tab Control 2" class="TabCtl (strict)"() -> ("Pages"=w292:refnum<vi>[])  [unwired: 2 in, 2 out]
            n230 = Index Array(array=w292, index=1) -> (element=w290:refnum<vi>)
            n231 = property class="Page"(reference=w290, "PageEnb"=T49."Page Enabled" ("Page Enabled State")) -> ()  [unwired: 1 in, 2 out]
          }
          frame #3 {
            # "Initialize CS"
            n232 = local read "CS ref"() -> (w316:refnum<class "CS.lvclass">)
            n233 = call-dynamic "Initialize.vi"("CS in"=w316, "HW Address"="HW Address", "error in (no error)"=T50 {"error"=FALSE, "code"=0, "source"=""} ("error in")) -> ("CS out"=w309:refnum<class "CS.lvclass">, "Instrument ID"=→"ID":string, "error out"=w308:errorcluster)  [unwired: 10 in]
            n234 = call-dynamic "Get Currents & Ranges.vi"("CS.lvclass in"=w309, "error in (no error)"=w308) -> ("CS.lvclass out"=w317:refnum<class "CS.lvclass">, "I0"=w318:cluster{"Value":dbl, "Range":dbl}, "I1"=w310:cluster{"Value":dbl, "Range":dbl}, "I2"=w311:cluster{"Value":dbl, "Range":dbl}, "I3"=w312:cluster{"Value":dbl, "Range":dbl}, "error out"=w314:errorcluster)  [unwired: 12 in]
            "CS status" <- w314
            n235 = local write "CS ref"(w317) -> ()
            n236 = Unbundle By Name(w314) -> ("status"=w306:bool)
            n237 = case shown="False" w306 {
              tunnel: w310 -> [w330 _]
              tunnel: w311 -> [w329 _]
              tunnel: w312 -> [w328 _]
              tunnel: w318 -> [w322 _]
              frame False {
                n238 = Unbundle By Name(w322) -> ("Value"=w321:dbl, "Range"=w320:dbl)
                n239 = Unbundle By Name(w330) -> ("Value"=w327:dbl, "Range"=w326:dbl)
                n240 = Unbundle By Name(w329) -> ("Value"=w325:dbl, "Range"=w324:dbl)
                n241 = Unbundle By Name(w328) -> ("Value"=w319:dbl, "Range"=w323:dbl)
                n242 = property on="I" class="DigNum (strict)"("Value"=w321) -> ()  [unwired: 2 in, 2 out]
                n243 = property on="I" class="DigNum (strict)"("Value"=w327) -> ()  [unwired: 2 in, 2 out]
                n244 = property on="I" class="DigNum (strict)"("Value"=w325) -> ()  [unwired: 2 in, 2 out]
                n245 = property on="I" class="DigNum (strict)"("Value"=w319) -> ()  [unwired: 2 in, 2 out]
                n246 = property on="Range" class="Enum (strict)"("Value"=w320) -> ()  [unwired: 2 in, 2 out]
                n247 = property on="Range" class="Enum (strict)"("Value"=w326) -> ()  [unwired: 2 in, 2 out]
                n248 = property on="Range" class="Enum (strict)"("Value"=w324) -> ()  [unwired: 2 in, 2 out]
                n249 = property on="Range" class="Enum (strict)"("Value"=w323) -> ()  [unwired: 2 in, 2 out]
                n250 = property on="I_0" class="DigNum (strict)"("Value"=w319) -> ()  [unwired: 2 in, 2 out]
              }
              frame True {
              }
            }
          }
          frame #4 {
            # "Initialize AVS/zBridge"
            n251 = property on="AVS type" class="Enum (strict)"() -> ("Value"=w335:T60)  [unwired: 2 in, 2 out]
            n252 = case shown="\"Impedance Bridge\"" w335 {
              tunnel: [w343 w352 w369 refnum<visa-resource-name> refnum ("dup VISA session") refnum<visa-resource-name> refnum ("dup VISA session")] -> w334
              tunnel: [w342 w355 _ w378 errorcluster {"status"=FALSE, "code"=0, "source"=""} ("error out")] -> w333
              tunnel: [TRUE ("start 2") TRUE ("start 2") TRUE ("start 2") TRUE ("start 2") TRUE ("start 2")] -> w336
              tunnel: [_ _ w368 _ _] -> _
              frame "AVS47A (GPIB interface)" {
                # "Set default Parameters,\n enable Autoranging"
                n253 = property on="Address" class="VISAName"() -> ("Value"=w337:refnum<visa-resource-name>)  [unwired: 2 in, 2 out]
                n254 = call "AVS47IB Initialize.vi"("Instr. Descriptor (GPIB::)"=w337) -> ("VISA session"=w351:refnum<visa-resource-name>, "error out"=w338:errorcluster)  [unwired: 13 in]
                n255 = call "AVS47IB Stop.vi"("VISA session"=w351, "error in (no error)"=w338) -> ("dup VISA session"=w349:refnum<visa-resource-name>, "error out"=w341:errorcluster)  [unwired: 12 in]
                n256 = call "AVS47IB Go Remote.vi"("VISA session"=w349, "error in (no error)"=w341) -> ("dup VISA session"=w350:refnum<visa-resource-name>, "error out"=w340:errorcluster)  [unwired: 12 in]
                n257 = call "AVS47IB Configure 47IB.vi"("VISA session"=w350, "Printer Enabled (-1:no change)"=i8 0, "Buffer Enabled (-1:no change)"=i8 0, "Message Headers Included  (-1:no change)"=i8 0, "Autoranging Enabled (-1:no change)"=i8 1, "Stabilisation Delay (-1:no change)"=i8 15, "error in (no error)"=w340) -> ("dup VISA session"=w343:refnum<visa-resource-name>, "error out"=w342:errorcluster)  [unwired: 7 in]
              }
              frame "AVS47B (RS232 interface)" {
                n258 = property on="Bridge settings" class="Clust (strict)"() -> ("Value"=w360:T35)  [unwired: 2 in, 2 out]
                n259 = Unbundle By Name(w360) -> ("AVS_SPort"=w359:refnum<visa-resource-name>)
                n260 = call "InitPort_b.vi"("VISA resource"=w359) -> ("error out"=w354:errorcluster, "dup VISA resource"=w358:refnum<visa-resource-name>)  [unwired: 5 in]
                n261 = Type Cast(type=refnum<visa-resource-name> refnum ("dup VISA session"), x=w358) -> (*(type *) &x=w353:refnum<visa-resource-name>)
                n262 = case shown="Error" w354 {
                  selector: w354 -> [w361 w364]
                  tunnel: w353 -> [w362 w366]
                  tunnel: [w361 w365] -> w355
                  tunnel: [w362 refnum<visa-resource-name> refnum ("dup VISA session")] -> w352
                  frame No Error {
                  }
                  frame Error {
                    n263 = VISA Close(VISA resource name=w366, error in (no error)=w364) -> (error out=w365:errorcluster)
                  }
                }
              }
              frame "AVS48SI (RS232 interface)" {
                n264 = property on="Bridge settings" class="Clust (strict)"() -> ("Value"=w373:T35)  [unwired: 2 in, 2 out]
                n265 = Unbundle By Name(w373) -> ("AVS_SPort"=w370:refnum<visa-resource-name>)
                n266 = call "Configure Hardware.vi"("VISA RESOURCE NAME"=w370) -> ("THREAD OUT"=w367:string)  [unwired: 14 in]
                n267 = call "Configure Sensor Wiring of CHs.vi"("THREAD IN"=w367) -> ("THREAD OUT"=w368:string)  [unwired: 10 in]
                n268 = Type Cast(type=refnum<visa-resource-name> refnum ("dup VISA session"), x=w370) -> (*(type *) &x=w369:refnum<visa-resource-name>)
              }
              frame "Impedance Bridge" {
                n269 = local read "zConfig"() -> (w377:path)
                n270 = local read "zDll"() -> (w374:path)
                n271 = call "SetParFilePath.vi"("path"=w377, "zDll"=w374) -> ("error out"=w376:errorcluster, "zDll out"=w375:path)  [unwired: 8 in]
                n272 = call "StartScan.vi"("error in (no error)"=w376, "path in"=w375) -> ("error out"=w378:errorcluster)  [unwired: 8 in, 1 out]
              }
              frame "Disabled", Default {
              }
            }
            "AVS VISA session" <- w334
            "start 2" <- w336
            n273 = property on="Bridge status" class="Clust (strict)"("Value"=w333) -> ()  [unwired: 2 in, 2 out]
            n274 = property on="Data array" class="Arr (strict)"("Value"=dbl[] [0.0, 0.0, 0.0, 0.0, 0.0, 0.0, 0.0, 0.0, 0.0, 0.0] ("R_array")) -> ()  [unwired: 2 in, 2 out]
            n275 = call "ScanParameters FGV.vi"("Action"=Action."Init") -> ()  [unwired: 10 in, 1 out]
          }
          frame #5 {
            # "Generate paths for log files"
            n276 = Unbundle By Name("Data logging") -> ("Run description"=w387:string, "Filenames suffix"=w388:string, "AVS_Path"=w385:path, "AVS_FName"=w391:string, "CAL_FName"=w390:string)
            n277 = call "Create Dir if Non-Existant__ogtk.vi"("Directory Path"=w385) -> ("dup Directory Path"=w384:path)  [unwired: 8 in, 2 out]
            n278 = call "MGI Make String Filesafe.vi"("String In"=w387) -> ("Filesafe String Out"=w386:string)
            n279 = call "GeneratePaths.vi"("Filename Suffix"=w388, "Run description"=w386, "AVS_Path"=w384, "AVS_FName"=w391, "CAL_Path"=w384, "CAL_FName"=w390) -> ("Generated Log path"=w389:path, "Generated Calib path"=→"Calib path":path)  [unwired: 8 in]
            n280 = property on="Log path" class="Path"("Val(Sgnl)"=w389) -> ()  [unwired: 2 in, 2 out]
          }
        }
      }
      event "Stop": Value Change; Application Instance Close {
        # "\"Stop\" button pressed -> Stop measuring."
        n281 = event-data() -> ()  [unwired: 1 in, 3 out]
        n282 = flat-sequence {
          frame #0 {
            (unwired) T58."HKEY_CURRENT_USER" ("root key (HKEY_LOCAL_MACHINE) 2")
            # "Save settings to config file"
            n283 = control-ref of="Active"() -> (w396:refnum<vi>)
            n284 = control-ref of="Bridge settings"() -> (w405:refnum<vi>)
            n285 = control-ref of="Runtime Settings"() -> (w404:refnum<vi>)
            n286 = control-ref of="Current source settings"() -> (w406:refnum<vi>)
            n287 = control-ref of="Data logging"() -> (w407:refnum<vi>)
            n288 = control-ref of="Thermometer"() -> (w403:refnum<vi>)
            n289 = control-ref of="PID setup"() -> (w402:refnum<vi>)
            n290 = control-ref of="CS Names"() -> (w401:refnum<vi>)
            n291 = control-ref of="AVS names"() -> (w400:refnum<vi>)
            n292 = control-ref of="CurCalibrations"() -> (w397:refnum<vi>)
            n293 = control-ref of="I3 as temp"() -> (w395:refnum<vi>)
            n294 = control-ref of="Automode Settings 2"() -> (w394:refnum<vi>)
            n295 = call "Current VIs Parent Directory__ogtk.vi"("Relative path (.)"=path "data/config.ini") -> ("Parent Directory (+ Relative)"=w398:path)  [unwired: 4 in]
            n296 = Build Array(w396, w405, w404, w406, w407, w403, w402, w401, w400, w397, w395, w394) -> (w409:refnum<vi>[])
            n297 = call "Save Load Settings to File by Ref with path.vi"("Array of Cluster References"=w409, "subkey"="SOFTWARE\\Leiden Cryogenics\\TC" ("subkey 2"), "Action"=enum8{"Load", "Save"}."Save", "configuration file path"=w398) -> ()  [unwired: 5 in, 1 out]
          }
          frame #1 {
            # "Free serial ports"
            n298 = control-ref of="AVS VISA session"() -> (w412:refnum<vi>)
            n299 = control-ref of="TCS_Port"() -> (w417:refnum<vi>)
            n300 = local read "zDll"() -> (w411:path)
            n301 = call "StopScan.vi"("path in"=w411) -> ()  [unwired: 9 in, 2 out]
            n302 = property class="VISAName"(reference=w412) -> (error out=w414:errorcluster, "Value"=w413:refnum<visa-resource-name>)  [unwired: 1 in, 1 out]
            n303 = property class="VISAName"(reference=w417) -> (error out=w415:errorcluster, "Value"=w416:refnum<visa-resource-name>)  [unwired: 1 in, 1 out]
            n304 = VISA Close(VISA resource name=w413, error in (no error)=w414) -> ()  [unwired: 1 out]
            n305 = VISA Close(VISA resource name=w416, error in (no error)=w415) -> ()  [unwired: 1 out]
          }
          frame #2 {
            w420 = u8 0 ("Disabled")
            # "Reset controls state"
            n306 = property on="AVS type" class="Enum (strict)"("Disabled"=w420) -> ()  [unwired: 2 in, 2 out]
            n307 = property on="Address" class="VISAName"("Disabled"=w420) -> ()  [unwired: 2 in, 2 out]
            n308 = property on="AVS_SPort" class="VISAName"("Disabled"=w420) -> ()  [unwired: 2 in, 2 out]
            n309 = property on="TCS_Port" class="VISAName"("Disabled"=w420) -> ()  [unwired: 2 in, 2 out]
            n310 = property on="CS type" class="Enum (strict)"("Disabled"=w420) -> ()  [unwired: 2 in, 2 out]
            n311 = property on="QCS/PCS Device" class="DigNum (strict)"("Disabled"=w420) -> ()  [unwired: 2 in, 2 out]
            n312 = property on="Start" class="Bool (strict)"("Visible"=TRUE, "Disabled"=u8 0, "Value"=FALSE ("start")) -> ()  [unwired: 2 in, 2 out]
            n313 = property on="Stop" class="Bool (strict)"("Value"=FALSE ("MainStopButton")) -> ()  [unwired: 2 in, 2 out]
            n314 = property on="start 2" class="Bool (strict)"("Value"=FALSE ("start 2")) -> ()  [unwired: 2 in, 2 out]
          }
          frame #3 {
            w424 = u8 2 ("Disabled")
            # "Disable UI"
            n315 = property on="Toolbar" class="TabCtl (strict)"("Disabled"=w424) -> ()  [unwired: 2 in, 2 out]
            n316 = property on="Tab Control" class="TabCtl (strict)"("Disabled"=w424) -> ()  [unwired: 2 in, 2 out]
            n317 = property on="Current indicators" class="TabCtl (strict)"("Disabled"=w424) -> ()  [unwired: 2 in, 2 out]
            n318 = property on="Tab Control 2" class="TabCtl (strict)"("Disabled"=w424) -> ()  [unwired: 2 in, 2 out]
            n319 = property on="Tab Control 5" class="TabCtl (strict)"("Disabled"=w424) -> ()  [unwired: 2 in, 2 out]
            n320 = property on="String" class="Str"("Visible"=TRUE) -> ()  [unwired: 2 in, 2 out]
          }
          frame #4 {
            # "Stop execution"
            n321 = Stop(stop? (T)=TRUE) -> ()
          }
        }
      }
      event "Data array": Value Change {
        # "Convert 8 elements AVS\narray to 10 elements"
        # "Received new data from AVS/zBridge. Do general tasks - update indicators, calculate temperature and pass the data further to \nAVS/zBridge specific processing"
        n322 = event-data() -> ("NewVal"=w441:dbl[])  [unwired: 1 in]
        n323 = Unbundle By Name(w429) -> ("UpdateValuesAVS"=w427:refnum<user-event>, "UpdateValuesZBridge"=w428:refnum<user-event>)
        n324 = for {
          tunnel: w441 -> [w471] mode=indexing
          tunnel: [w469] -> w437 mode=indexing
          n325 = Less?(x=w471, y=1e+25) -> (x < y?=w472:bool)
          n326 = Select(t=w471, s=w472, f=inf) -> (s? t:f=w469:dbl)
        }
        n327 = Index Array(array=w437) -> (element #1=→"R0":dbl, element #2=→"R1":dbl, element #3=→"R2":dbl, element #4=→"R3":dbl, element #5=→"R4":dbl, element #6=→"R5":dbl, element #7=→"R6":dbl, element #8=→"R7":dbl, element #9=→"R8":dbl, element #10=→"R9":dbl)  [unwired: 10 in]
        n328 = Array To Cluster(array=w437) -> (cluster=w431:T61)
        "R" <- w431
        n329 = Cluster To Array(cluster=w431) -> (array=w430:dbl[])
        n330 = Absolute Value(x=w430) -> (abs(x)=w438:dbl[])
        n331 = property on="Allow neg R" class="Bool (strict)"() -> ("Value"=w436:bool)  [unwired: 2 in, 2 out]
        n332 = Select(t=w430, s=w436, f=w438) -> (s? t:f=w435:dbl[])
        "R_array" <- w435
        n333 = local read "CurCalibrations"() -> (w443:T33)
        n334 = property on="AVS_CalFolder" class="Path"() -> ("Value"=w451:path)  [unwired: 2 in, 2 out]
        n335 = Cluster To Array(cluster=w443) -> (array=w442:string[])
        n336 = call "Resistance to Temp no Ext.vi"("error in"=w444, "Path"=w451, "CurCalibrations"=w442, "Resistance"=w435) -> ("Temperature"=w433:dbl[])  [unwired: 1 in, 3 out]
        "T_array" <- w433
        n337 = Array To Cluster(array=w433) -> (cluster=w449:T62)
        "T" <- w449
        n338 = Unbundle(w449) -> ("Temperature[0]"=→"T0":dbl, "Temperature[1]"=→"T1":dbl, "Temperature[2]"=→"T2":dbl, "Temperature[3]"=→"T3":dbl, "Temperature[4]"=→"T4":dbl, "Temperature[5]"=→"T5":dbl, "Temperature[6]"=→"T6":dbl, "Temperature[7]"=→"T7":dbl, "Temperature[8]"=→"T8":dbl, "Temperature[9]"=→"T9":dbl)
        n339 = property on="Mode Buttons" class="RadioBtnsControl (strict)"() -> ("Value"=w448:T7)  [unwired: 2 in, 2 out]
        n340 = Array To Cluster(array=w435) -> (cluster=w434:T61)
        n341 = Array To Cluster(array=w433) -> (cluster=w432:T62)
        n342 = case shown="\"No Selection\", Default" w448 {
          tunnel: w432 -> [w484 _]
          tunnel: w434 -> [w485 _]
          frame "No Selection", Default {
            n343 = call "Current Time(double).vi"() -> ("Current Time (double)"=→"Time":dbl)  [unwired: 6 in, 1 out]
            "Small R" <- w485
            "Small T" <- w484
          }
          frame "Cursor mode" {
          }
        }
        n344 = Bundle(w435, "Temperature"=w433) -> (w446:cluster{dbl[], "Temperature":dbl[]})  [unwired: 1 in]
        n345 = property on="AVS type" class="Enum (strict)"() -> ("Value"=w445:T60)  [unwired: 2 in, 2 out]
        n346 = case shown="\"AVS47B (RS232 interface)\", Default" w445 {
          tunnel: [w477 w478 w481] -> w447
          tunnel: w444 -> [w476 w478 w482]
          tunnel: w446 -> [w475 _ w480]
          tunnel: w428 -> [_ _ w479]
          tunnel: w427 -> [w474 _ _]
          frame "AVS47B (RS232 interface)", Default {
            n347 = Generate User Event(user event=w474, event data cluster=w475, error in=w476) -> (error out=w477:errorcluster)  [unwired: 1 in, 1 out]
          }
          frame "Disabled" {
          }
          frame "Impedance Bridge" {
            n348 = Generate User Event(user event=w479, event data cluster=w480, error in=w482) -> (error out=w481:errorcluster)  [unwired: 1 in, 1 out]
          }
        }
      }
      event User Event {
        # "Process data from the AVS bridge"
        n349 = event-data() -> ("R"=w489:dbl[], "T"=w488:dbl[])  [unwired: 1 in]
        n350 = Unbundle By Name(w487) -> ("CS Automode"=w486:refnum<user-event>)
        n351 = property on="Actual I" class="Arr (strict)"() -> ("Value"=w490:dbl[])  [unwired: 2 in, 2 out]
        n352 = stacked-sequence {
          tunnel: w492 -> [_ w515]
          tunnel: [_ w537] -> w491
          tunnel: w490 -> [_ w518]
          tunnel: w489 -> [w496 w520]
          tunnel: w488 -> [w495 w519]
          tunnel: w486 -> [w493 _]
          frame #0 {
            # "Filter data and add it to the data array. \nDo PID"
            n353 = property on="Runtime Settings" class="Clust (strict)"() -> ("Value"=w500:T27)  [unwired: 2 in, 2 out]
            n354 = Unbundle By Name(w500) -> ("Y_max"=w503:dbl, "Y_min"=w502:dbl, "Filter graphs:"=w501:bool)
            n355 = local read "Data"() -> (w498:T28)
            n356 = property on="Data Memory" class="DigNum (strict)"() -> ("Value"=w505:u16)  [unwired: 2 in, 2 out]
            n357 = call "Current Time(double).vi"() -> ("Current Time (double)"=w494:dbl)  [unwired: 6 in, 1 out]
            n358 = call "Manage Data Arrays - AVS.vi"("Y_max"=w503, "Y_min"=w502, "Filter Graph Results"=w501, "Append New Data"=TRUE, "Data In"=w498, "Curr R"=w496, "Curr T"=w495, "Curr Time"=w494, "Data Memory"=w505) -> ("Data Out"=w499:T28)  [unwired: 10 in]
            n359 = Bundle("Current Time (double)"=w494, "R"=w496, "T"=w495) -> (w506:T63)  [unwired: 1 in]
            n360 = local write "Data"(w499) -> ()
            n361 = Generate User Event(user event=w493, event data cluster=w506) -> ()  [unwired: 2 in, 2 out]
            n362 = local write "Units"(T19 {"AVS Name 0"="O\u0000h\u0000m\u0000\u0000\u0000\u0000\u0000\u0000\u0000\u0000\u0000\u0000\u0000\u0000\u0000\u0000\u0000", "AVS Name 1"="O\u0000h\u0000m\u0000\u0000\u0000\u0000\u0000\u0000\u0000\u0000\u0000\u0000\u0000\u0000\u0000\u0000\u0000", "AVS Name 2"="O\u0000h\u0000m\u0000\u0000\u0000\u0000\u0000\u0000\u0000\u0000\u0000\u0000\u0000\u0000\u0000\u0000\u0000", "AVS Name 3"="O\u0000h\u0000m\u0000\u0000\u0000\u0000\u0000\u0000\u0000\u0000\u0000\u0000\u0000\u0000\u0000\u0000\u0000", "AVS Name 4"="O\u0000h\u0000m\u0000\u0000\u0000\u0000\u0000\u0000\u0000\u0000\u0000\u0000\u0000\u0000\u0000\u0000\u0000", "AVS Name 5"="O\u0000h\u0000m\u0000\u0000\u0000\u0000\u0000\u0000\u0000\u0000\u0000\u0000\u0000\u0000\u0000\u0000\u0000", "AVS Name 6"="O\u0000h\u0000m\u0000\u0000\u0000\u0000\u0000\u0000\u0000\u0000\u0000\u0000\u0000\u0000\u0000\u0000\u0000", "AVS Name 7"="O\u0000h\u0000m\u0000\u0000\u0000\u0000\u0000\u0000\u0000\u0000\u0000\u0000\u0000\u0000\u0000\u0000\u0000", "AVS Name 8"="O\u0000h\u0000m\u0000\u0000\u0000\u0000\u0000\u0000\u0000\u0000\u0000\u0000\u0000\u0000\u0000\u0000\u0000", "AVS Name 9"="O\u0000h\u0000m\u0000\u0000\u0000\u0000\u0000\u0000\u0000\u0000\u0000\u0000\u0000\u0000\u0000\u0000\u0000"} ("Units")) -> ()
          }
          frame #1 {
            # "Save data to log file"
            n363 = local read "Calib path"() -> (w536:path)
            n364 = local read "Log path"() -> (w535:path)
            n365 = call <vilib>:"Check if File or Folder Exists.vi"("path"=w535) -> ("file or folder exists?"=w527:bool, "dup path"=w528:path)  [unwired: 8 in, 1 out]
            n366 = case shown="False" w527 {
              tunnel: w528 -> [w561 w568]
              tunnel: [w561 w568] -> w529
              frame False {
                n367 = control-ref of="Thermometer"() -> (w564:refnum<vi>)
                n368 = property on="Run description" class="Str"() -> ("Value"=w560:string)  [unwired: 2 in, 2 out]
                n369 = Cluster To Array(cluster="AVS names") -> (array=w566:string[])
                n370 = Cluster To Array(cluster="CS Names") -> (array=w567:string[])
                n371 = call "Format log file header Z.vi"("Thermometer"=w564, "AVS names"=w566, "CS Names"=w567, "Run description"=w560) -> ("String"=w562:string)  [unwired: 1 in]
                n372 = Write to Text File(file (use dialog)=w561, text=w562) -> ()  [unwired: 2 in, 3 out]
              }
              frame True {
              }
            }
            n373 = property on="Data logging" class="Clust (strict)"() -> ("Value"=w547:T37)  [unwired: 2 in, 2 out]
            n374 = Unbundle By Name(w547) -> ("Delimeter"=w548:string, "Date/Time Format"=w546:string)
            n375 = call "File Info__ogtk.vi"("file"=w529) -> ("file info"=w525:T64, "file out"=w534:path)  [unwired: 5 in, 1 out]
            n376 = call "Current Time(double).vi"() -> ("Current Time"=w522:timestamp, "Current Time (double)"=w523:dbl)  [unwired: 6 in]
            n377 = Unbundle By Name(w525) -> ("creation date"=w526:u32)
            n378 = Number To Exponential String(number=w523, precision (6)=i16 10) -> (E-format string=w540:string)  [unwired: 2 in]
            n379 = Format Date/Time String(time format string (%c)=w546, seconds (now)=w522) -> (date/time string=w543:string)  [unwired: 1 in]
            n380 = Number To Fractional String(number=w520) -> (F-format string=w545:string[])  [unwired: 3 in]
            n381 = Number To Fractional String(number=w519) -> (F-format string=w544:string[])  [unwired: 3 in]
            n382 = Number To Fractional String(number=w518) -> (F-format string=w542:string[])  [unwired: 3 in]
            n383 = property on="NewFevery" class="DigNum (strict)"() -> ("Value"=w530:u32)  [unwired: 2 in, 2 out]
            n384 = property on="Time Units" class="Enum (strict)"() -> ("Value"=w531:enum16{"Minutes", "Hours", "Days"})  [unwired: 2 in, 2 out]
            n385 = To Time Stamp(1:w526) -> (0:w532:timestamp)
            n386 = Build Array (concatenate)(w543, w540, w545, w544, w542) -> (w512:string[])
            n387 = local read "Bridge settings"() -> (w516:T35)
            n388 = call "Time Elapsed time.vi"("Time Units"=w531, "Delay Time"=w530, "Time Old In"=w532) -> ("T>dT?"=w533:bool)  [unwired: 2 out]
            n389 = case shown="True" w533 {
              tunnel: [w550 w553] -> w524
              tunnel: [w549 w554] -> _
              tunnel: w534 -> [w550 _]
              tunnel: w536 -> [w549 _]
              frame False {
              }
              frame True {
                n390 = local read "Data logging"() -> (w555:T37)
                n391 = Unbundle By Name(w555) -> ("Run description"=w551:string, "AVS_Path"=w559:path, "AVS_FName"=w557:string, "CAL_FName"=w558:string, "Filenames suffix"=w556:string)
                n392 = call "MGI Make String Filesafe.vi"("String In"=w551) -> ("Filesafe String Out"=w552:string)
                n393 = call "GeneratePaths.vi"("Filename Suffix"=w556, "Run description"=w552, "AVS_Path"=w559, "AVS_FName"=w557, "CAL_Path"=w559, "CAL_FName"=w558) -> ("Generated Log path"=w553:path, "Generated Calib path"=w554:path)  [unwired: 8 in]
                n394 = local write "Calib path"(w554) -> ()
                n395 = property on="Log path" class="Path"("Val(Sgnl)"=w553) -> ()  [unwired: 2 in, 2 out]
              }
            }
            n396 = local read "AVS names"() -> (w517:T10)
            n397 = property on="Thermometer" class="Clust (strict)"() -> ("Controls[]"=w513:refnum<vi>[])  [unwired: 2 in, 2 out]
            n398 = Unbundle By Name(w516) -> ("AVS type"=w511:T60)
            n399 = To Unsigned Long Integer(number=w511) -> (unsigned 32bit integer=w508:u32)
            n400 = Variant To Data(type=T52."AVS47A (GPIB interface)" ("AVS type"), Variant=w508) -> (data=w509:T52)  [unwired: 1 in, 1 out]
            n401 = Bundle By Name(cluster=T53 {"R"=[], "T"=[], "I"=[], "AVS type"=enum."AVS47A (GPIB interface)", "AVS names"={"AVS Name 0"="", "AVS Name 1"="", "AVS Name 2"="", "AVS Name 3"="", "AVS Name 4"="", "AVS Name 5"="", "AVS Name 6"="", "AVS Name 7"="", "AVS Name 8"="", "AVS Name 9"=""}, "Calibration"=[]} ("TC Cluster"), "Calibration"=w513, "AVS names"=w517, "R"=w520, "T"=w519, "I"=w518, "AVS type"=w509) -> (w507:T53)
            n402 = call "TC_to_DSC.vi"("error in (no error)"=w515, "TC Cluster"=w507) -> ("error out"=w514:errorcluster)  [unwired: 9 in]
            n403 = call "Write To Spreadsheet File (string) w Error.vi"("delimiter (\\t)"=w548, "append to file? (new file:F)"=TRUE, "1D data"=w512, "file path (dialog if empty)"=w524) -> ("error out"=w538:errorcluster)  [unwired: 6 in, 1 out]
            n404 = Merge Errors(w538, w514) -> (w537:errorcluster)
          }
        }
      }
      event User Event {
        # "Process data from the zBridge bridge"
        n405 = event-data() -> ("R"=w577:dbl[], "T"=w576:dbl[])  [unwired: 1 in, 4 out]
        n406 = Unbundle By Name(w571) -> ("CS Automode"=w570:refnum<user-event>)
        n407 = local read "Par/Err"() -> (w572:string)
        n408 = local read "Set #"() -> (w578:u8)
        n409 = property on="Actual I" class="Arr (strict)"() -> ("Value"=w575:dbl[])  [unwired: 2 in, 2 out]
        n410 = local read "Unit"() -> (w573:string)
        n411 = stacked-sequence {
          tunnel: w572 -> [w599 _]
          tunnel: w578 -> [w584 w605]
          tunnel: w577 -> [w582 w631]
          tunnel: w576 -> [w581 w630]
          tunnel: w575 -> [_ w629]
          tunnel: w574 -> [_ w628]
          tunnel: [_ w627] -> w569
          tunnel: w573 -> [w586 _]
          tunnel: w570 -> [w583 _]
          frame #0 {
            # "Only do PID after measuring\non selected channel( or any \nchannel if -1 is selected)"
            n412 = local read "zBridge params"() -> (w585:T19)
            n413 = local read "Units"() -> (w587:T13)
            n414 = Cluster To Array(cluster=w587) -> (array=w590:string[])
            n415 = Cluster To Array(cluster=w585) -> (array=w600:string[])
            n416 = Replace Array Subset(array=w590, new element=w586, index=w584) -> (w589:string[])
            n417 = Replace Array Subset(array=w600, new element=w599, index=w584) -> (w601:string[])
            n418 = Array To Cluster(array=w589) -> (cluster=→"Units":T65)
            n419 = Array To Cluster(array=w601) -> (cluster=→"zBridge params":T66)
            n420 = property on="Runtime Settings" class="Clust (strict)"() -> ("Value"=w593:T27)  [unwired: 2 in, 2 out]
            n421 = Unbundle By Name(w593) -> ("Y_max"=w596:dbl, "Y_min"=w595:dbl, "Filter graphs:"=w594:bool)
            n422 = local read "Data"() -> (w591:T28)
            n423 = property on="Data Memory" class="DigNum (strict)"() -> ("Value"=w598:u16)  [unwired: 2 in, 2 out]
            n424 = call "Current Time(double).vi"() -> ("Current Time (double)"=w579:dbl)  [unwired: 6 in, 1 out]
            n425 = call "Manage Data Arrays - zBridge.vi"("Y_max"=w596, "Y_min"=w595, "Filter Graph Results"=w594, "Append New Data"=TRUE, "Data In"=w591, "Curr R"=w582, "Curr T"=w581, "Curr Time"=w579, "Channel"=w584, "Data Memory"=w598) -> ("Data Out"=w592:T28)  [unwired: 9 in]
            n426 = local write "Data"(w592) -> ()
            n427 = Bundle("Current Time (double)"=w579, "R"=w582, "T"=w581) -> (w580:T63)  [unwired: 1 in]
            n428 = Generate User Event(user event=w583, event data cluster=w580) -> ()  [unwired: 2 in, 2 out]
          }
          frame #1 {
            n429 = local read "Log path"() -> (w608:path)
            n430 = local read "Data logging"() -> (w626:T37)
            n431 = call "Strip Path Extension - Path__ogtk.vi"("path"=w608) -> ("root"=w609:string, "extension"=w612:string)
            n432 = Format Into String(format string="_%d", initial string=w609, w605) -> (resulting string=w610:string)  [unwired: 1 in, 1 out]
            n433 = Unbundle By Name(w626) -> ("Delimeter"=w642:string, "Date/Time Format"=w641:string)
            n434 = Concatenate Strings(w610, "." ("string"), w612) -> (w607:string)
            n435 = String To Path(string=w607) -> (path=w606:path)
            n436 = call <vilib>:"Check if File or Folder Exists.vi"("path"=w606) -> ("file or folder exists?"=w617:bool, "dup path"=w618:path)  [unwired: 8 in, 1 out]
            n437 = case shown="False" w617 {
              tunnel: w618 -> [w659 w662]
              tunnel: [w659 w662] -> w619
              frame False {
                n438 = local read "AVS names"() -> (w658:T10)
                n439 = local read "CS Names"() -> (w657:T31)
                n440 = control-ref of="Thermometer"() -> (w661:refnum<vi>)
                n441 = property on="Run description" class="Str"() -> ("Value"=w654:string)  [unwired: 2 in, 2 out]
                n442 = Cluster To Array(cluster=w658) -> (array=w655:string[])
                n443 = Cluster To Array(cluster=w657) -> (array=w656:string[])
                n444 = call "Format log file header Z.vi"("Thermometer"=w661, "AVS names"=w655, "CS Names"=w656, "Run description"=w654) -> ("String"=w660:string)  [unwired: 1 in]
                n445 = Write to Text File(file (use dialog)=w659, text=w660) -> ()  [unwired: 2 in, 3 out]
              }
              frame True {
              }
            }
            n446 = call "Current Time(double).vi"() -> ("Current Time"=w603:timestamp, "Current Time (double)"=w604:dbl)  [unwired: 6 in]
            n447 = Number To Exponential String(number=w604, precision (6)=i16 10) -> (E-format string=w634:string)  [unwired: 2 in]
            n448 = Format Date/Time String(time format string (%c)=w641, seconds (now)=w603) -> (date/time string=w638:string)  [unwired: 1 in]
            n449 = Number To Exponential String(number=w631) -> (E-format string=w640:string[])  [unwired: 3 in]
            n450 = Number To Engineering String(4:w630) -> (0:w639:string[])  [unwired: 3 in]
            n451 = Number To Fractional String(number=w629) -> (F-format string=w637:string[])  [unwired: 3 in]
            n452 = call "File Info__ogtk.vi"("file"=w619) -> ("file info"=w615:T64, "file out"=w624:path)  [unwired: 5 in, 1 out]
            n453 = Unbundle By Name(w615) -> ("creation date"=w616:u32)
            n454 = Build Array (concatenate)(w638, w634, w640, w639, w637) -> (w636:string[])
            n455 = local read "Calib path"() -> (w625:path)
            n456 = property on="NewFevery" class="DigNum (strict)"() -> ("Value"=w620:u32)  [unwired: 2 in, 2 out]
            n457 = property on="Time Units" class="Enum (strict)"() -> ("Value"=w621:enum16{"Minutes", "Hours", "Days"})  [unwired: 2 in, 2 out]
            n458 = To Time Stamp(1:w616) -> (0:w622:timestamp)
            n459 = call "Time Elapsed time.vi"("Time Units"=w621, "Delay Time"=w620, "Time Old In"=w622) -> ("T>dT?"=w623:bool)  [unwired: 2 out]
            n460 = case shown="True" w623 {
              tunnel: [w644 w647] -> w614
              tunnel: [w643 w649] -> _
              tunnel: w624 -> [w644 _]
              tunnel: w625 -> [w643 _]
              frame False {
              }
              frame True {
                n461 = local read "Data logging"() -> (w650:T37)
                n462 = Unbundle By Name(w650) -> ("Run description"=w646:string, "Filenames suffix"=w648:string, "AVS_Path"=w653:path, "AVS_FName"=w651:string, "CAL_FName"=w652:string)
                n463 = call "MGI Make String Filesafe.vi"("String In"=w646) -> ("Filesafe String Out"=w645:string)
                n464 = call "GeneratePaths.vi"("Filename Suffix"=w648, "Run description"=w645, "AVS_Path"=w653, "AVS_FName"=w651, "CAL_Path"=w653, "CAL_FName"=w652) -> ("Generated Log path"=w647:path, "Generated Calib path"=w649:path)  [unwired: 8 in]
                n465 = local write "Calib path"(w649) -> ()
                n466 = property on="Log path" class="Path"("Val(Sgnl)"=w647) -> ()  [unwired: 2 in, 2 out]
              }
            }
            n467 = call "Write To Spreadsheet File (string) w Error.vi"("delimiter (\\t)"=w642, "append to file? (new file:F)"=TRUE, "1D data"=w636, "file path (dialog if empty)"=w614) -> ("error out"=w632:errorcluster)  [unwired: 6 in, 1 out]
            n468 = Merge Errors(w632, w628) -> (w627:errorcluster)
          }
        }
      }
      event User Event {
        # "Current source automatic mode"
        n469 = event-data() -> ("R"=w668:dbl[], "T"=w669:dbl[], "Time"=w663:dbl)  [unwired: 1 in, 4 out]
        n470 = local read "CS Mode"() -> (w667:T39)
        n471 = Unbundle By Name(w666) -> ("CallExtVI"=w665:refnum<user-event>, "TempStabilized"=w664:refnum<user-event>)
        n472 = case shown="\"Mode 1\"" w667 {
          tunnel: w669 -> [_ w673 w746]
          tunnel: w668 -> [_ w674 w747]
          tunnel: w665 -> [_ w676 _]
          tunnel: w664 -> [_ w675 _]
          tunnel: w663 -> [_ w672 _]
          frame "Manual", Default {
          }
          frame "Mode 1" {
            n473 = call "MGI Change Detector (T).vi"("Value"="Mode1 ON") -> ("Changed?"=w670:bool)
            n474 = case shown="True" "Mode1 ON" {
              tunnel: w676 -> [_ w689]
              tunnel: w675 -> [_ w688]
              tunnel: w674 -> [_ w687]
              tunnel: w673 -> [_ w686]
              tunnel: w672 -> [_ w683]
              tunnel: w670 -> [_ w677]
              frame False {
              }
              frame True {
                # "Check if PID error (SP-PV)==0"
                # "Check if temperature\nis stabilized"
                # "T sabilized?"
                # "If TCS auto mode enabled and temperature is not changing => fire TempStabilized event to save log and set new CS point. Otherwise do PID (if enabled)."
                # "Check if stabilization delay time \nis elapsed"
                n475 = property on="R/T?" class="Enum (strict)"() -> ("Value"=w685:enum16{"Resistance", "Temperature"})  [unwired: 2 in, 2 out]
                n476 = case shown="\"Temperature\"" w685 {
                  tunnel: [w704 w705] -> w681
                  tunnel: w687 -> [w704 _]
                  tunnel: w686 -> [_ w705]
                  frame "Resistance", Default {
                  }
                  frame "Temperature" {
                  }
                }
                n477 = property on="AVS Channel" class="DigNum (strict)"() -> ("Value"=w680:i32)  [unwired: 2 in, 2 out]
                n478 = Index Array(array=w681, index=w680) -> (element=w679:dbl)
                n479 = local read "Error"() -> (w696:dbl)
                n480 = local read "Time Old"() -> (w702:dbl)
                n481 = local read "I_list[i]"() -> (w690:T23[])
                n482 = property on="Delay Time" class="DigNum (strict)"() -> ("Value"=w692:dbl)  [unwired: 2 in, 2 out]
                n483 = property on="N averages" class="DigNum (strict)"() -> ("Value"=w678:i32)  [unwired: 2 in, 2 out]
                n484 = property on="T stability" class="DigNum (strict)"() -> ("Value"=w691:dbl)  [unwired: 2 in, 2 out]
                n485 = property on="PID on Ch#" class="Enum (strict)"() -> ("Value"=w682:enum16{"0", "1", "2", "3"})  [unwired: 2 in, 2 out]
                n486 = Equal To 0?(x=w696) -> (x = 0?=w694:bool)
                n487 = call "Derivatives Pt by Pt.vi"("initialize"=w677, "accuracy (%)"=w691, "Time"=w683, "Data"=w679, "Points to avg"=w678) -> ("Stable?"=w695:bool, "Stability (%)"=→"Slope":dbl, "dt (s)"=w699:dbl)  [unwired: 2 in]
                n488 = Index Array(array=w690, index=w682) -> (element=w703:T23)
                n489 = call "Time Elapsed dbl.vi"("Delay Time"=w692, "Time Old In"=w702) -> ("T>dT?"=w684:bool, "Delta T"=→"Timer":dbl, "Time New Out"=w701:dbl)  [unwired: 1 in]
                n490 = Compound Arithmetic op=AND(w684, w694, w695) -> (w697:bool)
                "SP reached?" <- w697
                n491 = property on="Enable PID" class="Bool (strict)"() -> ("Value"=w693:bool)  [unwired: 2 in, 2 out]
                n492 = case shown="False" w697 {
                  tunnel: w701 -> [_ w725]
                  tunnel: w699 -> [w721 _]
                  tunnel: w693 -> [w710 _]
                  tunnel: w703 -> [w718 _]
                  tunnel: w690 -> [w715 _]
                  tunnel: w682 -> [w708 _]
                  tunnel: w689 -> [_ w723]
                  tunnel: w688 -> [_ w722]
                  tunnel: w679 -> [w707 _]
                  frame False {
                    # "Temperature is not stable. If enabled, do PID regulation"
                    n493 = local read "I"() -> (w712:dbl[])
                    n494 = Index Array(array=w712, index=w708) -> (element=w713:dbl)
                    n495 = Multiply(x=1000.0, y=w713) -> (x*y=w711:dbl)
                    n496 = call "PID control incremental.vi"("Process Variable"=w707, "dt"=w721, "Setpoint"=w718, "PID Settings"="PID setup", "I in"=w711, "PID Enabled"=w710) -> ("PID output I"=→"Waveform Chart":T22, "err out"=→"Error":dbl, "int out"=→"Int":dbl, "I out"=w717:dbl)  [unwired: 10 in]
                    n497 = Replace Array Subset(array=w715, new element=w717, index=w708) -> (→"I_in":T23[])
                  }
                  frame True {
                    # "Temperature is stable & automode is on"
                    n498 = case shown="False" "Call ext. VI" {
                      tunnel: w725 -> [w728 _]
                      tunnel: w723 -> [_ w729]
                      tunnel: w722 -> [w726 _]
                      frame False {
                        # "External VI call disabled -> proceed\nwith automode"
                        n499 = local write "Time Old"(w728) -> ()
                        n500 = Generate User Event(user event=w726, event data cluster=TRUE ("event data")) -> ()  [unwired: 2 in, 2 out]
                      }
                      frame True {
                        # "Call external VI"
                        n501 = Generate User Event(user event=w729, event data cluster="" ("event data")) -> ()  [unwired: 2 in, 2 out]
                      }
                    }
                  }
                }
              }
            }
          }
          frame "Mode2" {
            n502 = case shown="\"Resistance\", Default" "FB on" {
              tunnel: [w749 w750] -> w743
              tunnel: w747 -> [w749 _]
              tunnel: w746 -> [_ w750]
              frame "Resistance", Default {
              }
              frame "Temperature" {
              }
            }
            n503 = Index Array(array=w743, index="AVS Channel") -> (element=w742:dbl)
            n504 = local read "I_list 2"() -> (w741:dbl[][])
            n505 = call "Currents-Temp list  - T in range?.vi"("T0 index"=0, "T1 index"=1, "T"=w742, "List in"=w741) -> ("I_out"=w734:dbl[], "List index"=w735:i32)  [unwired: 1 out]
            n506 = case shown="True" "Mode2 ON" {
              tunnel: w734 -> [_ w748]
              frame False {
              }
              frame True {
                n507 = local write "I_in"(w748) -> ()
              }
            }
            n508 = Initialize Array(FALSE, 16 ("dimension size")) -> (w738:bool[])
            n509 = Replace Array Subset(array=w738, new element=TRUE ("new element/subarray"), index=w735) -> (→"I_selection 2":bool[])
          }
        }
      }
      event User Event {
        n510 = event-data() -> ()  [unwired: 1 in, 5 out]
        n511 = Unbundle By Name(w752) -> ("TempStabilized"=w751:refnum<user-event>)
        n512 = local read "vi reference"() -> (w756:refnum<vi>)
        n513 = call "GetExtVIStatus.vi"("vi reference in"=w756) -> ("vi reference out"=w753:refnum<vi>, "Exec.State"=w755:T46, "Finished?"=w754:bool)
        n514 = case shown="\"Idle\"" w755 {
          tunnel: w754 -> [_ _]
          tunnel: w753 -> [_ w758]
          tunnel: w751 -> [_ w757]
          frame "Bad", Default {
          }
          frame "Idle" {
            n515 = local read "VI called?"() -> (w759:bool)
            n516 = case shown="False" w759 {
              tunnel: w758 -> [w761 _]
              tunnel: w757 -> [_ w768]
              frame False {
                n517 = property on="Data array" class="Arr (strict)"() -> ("Value"=w764:dbl[])  [unwired: 2 in, 2 out]
                n518 = property on="T_array" class="Arr (strict)"() -> ("Value"=w765:dbl[])  [unwired: 2 in, 2 out]
                n519 = property on="I" class="Arr (strict)"() -> ("Value"=w766:dbl[])  [unwired: 2 in, 2 out]
                n520 = Format Date/Time String() -> (date/time string=w763:string)  [unwired: 3 in]
                n521 = Bundle("date/time string"=w763, "Value"=w764, "Value"=w765, "Value"=w766) -> (w762:T67)  [unwired: 1 in]
                n522 = call "CallExtVI.vi"("vi reference in"=w761, "Cluster"=w762) -> ()  [unwired: 1 out]
                "VI called?" <- TRUE ("VI called?")
              }
              frame True {
                n523 = call "Current Time(double).vi"() -> ("Current Time (double)"=w767:dbl)  [unwired: 6 in, 1 out]
                n524 = Generate User Event(user event=w768, event data cluster=TRUE ("event data")) -> ()  [unwired: 2 in, 2 out]
                n525 = local write "Time Old"(w767) -> ()
              }
            }
          }
        }
      }
      event User Event {
        # "CS automode\nT is stabilized"
        n526 = event-data() -> ("TempStabilized"=w771:bool)  [unwired: 1 in, 4 out]
        n527 = stacked-sequence {
          tunnel: w772 -> [w778 _]
          tunnel: [w779 _] -> w770
          tunnel: w771 -> [_ w799]
          frame #0 {
            # "Step1: Save R,T,I values to calibration file. Make screenshot when creating the calibration file."
            n528 = property on="Calib path" class="Path"() -> ("Value"=w774:path)  [unwired: 2 in, 2 out]
            n529 = call "File Exists - Scalar__ogtk.vi"("file path"=w774) -> ("exists"=w775:bool)  [unwired: 6 in, 1 out]
            n530 = case shown="False" w775 {
              tunnel: w774 -> [w788 w798]
              tunnel: [w788 w798] -> w773
              frame False {
                n531 = local read "AVS names"() -> (w795:T10)
                n532 = local read "CS Names"() -> (w794:T31)
                n533 = control-ref of="Thermometer"() -> (w797:refnum<vi>)
                n534 = property on="Run description" class="Str"() -> ("Value"=w791:string)  [unwired: 2 in, 2 out]
                n535 = Cluster To Array(cluster=w795) -> (array=w792:string[])
                n536 = Cluster To Array(cluster=w794) -> (array=w793:string[])
                n537 = call "Format log file header Z.vi"("Thermometer"=w797, "AVS names"=w792, "CS Names"=w793, "Run description"=w791) -> ("String"=w796:string)  [unwired: 1 in]
                n538 = Write to Text File(file (use dialog)=w788, text=w796) -> ()  [unwired: 2 in, 3 out]
                n539 = control-ref of="This VI"() -> (w790:refnum<vi>)
                n540 = invoke class="VI" method="FP.Get Image"(reference=w790) -> ("image data"=w789:T68)  [unwired: 5 in, 5 out]
                n541 = call "Convert File Extension (Path)__ogtk.vi"("new ending (none)"="png" ("name or relative path"), "file name"=w788) -> ("new filename"=w787:path)  [unwired: 1 out]
                n542 = call <vilib>:"Write PNG File.vi"("image data"=w789, "path to PNG file"=w787) -> ()  [unwired: 8 in, 2 out]
              }
              frame True {
              }
            }
            n543 = local write "VI called?"(FALSE ("VI called?")) -> ()
            n544 = property on="Data logging" class="Clust (strict)"() -> ("Value"=w782:T37)  [unwired: 2 in, 2 out]
            n545 = Unbundle By Name(w782) -> ("Date/Time Format"=w783:string, "Delimeter"=w780:string)
            n546 = property on="R" class="Clust (strict)"() -> ("Value"=w781:T14)  [unwired: 2 in, 2 out]
            n547 = property on="T" class="Clust (strict)"() -> ("Value"=w785:T9)  [unwired: 2 in, 2 out]
            n548 = property on="I" class="Arr (strict)"() -> ("Value"=w784:dbl[])  [unwired: 2 in, 2 out]
            n549 = call "Write to cal log file.vi"("Value 2"=w784, "Date/Time Format"=w783, "Value 3"=w785, "Value"=w781, "Delimeter"=w780, "Value 4"=w773) -> ("error out"=w777:errorcluster)  [unwired: 1 out]
            n550 = Merge Errors(w777, w778) -> (w779:errorcluster)
          }
          frame #1 {
            # "Step 2: Sweep through the currents list"
            n551 = case shown="True" w799 {
              frame False {
              }
              frame True {
                n552 = local read "I_list_idx_max"() -> (w801:i32)
                n553 = local read "I_list_idx"() -> (w802:i32)
                n554 = Less?(x=w802, y=w801) -> (x < y?=w800:bool)
                n555 = case shown="False" w800 {
                  frame False {
                    n556 = property on="CS Mode" class="Enum (strict)"("Val(Sgnl)"=CS_mode."Manual" ("CS Mode")) -> ()  [unwired: 2 in, 2 out]
                  }
                  frame True {
                    n557 = property on="I_next" class="Bool (strict)"("Val(Sgnl)"=TRUE) -> ()  [unwired: 2 in, 2 out]
                  }
                }
              }
            }
          }
        }
      }
      event User Event {
        # "Disable controls for disabled channels"
        n558 = event-data() -> ()  [unwired: 1 in, 5 out]
        n559 = property on="AVS type" class="Enum (strict)"() -> ("Value"=w812:T60)  [unwired: 2 in, 2 out]
        n560 = case shown="\"Impedance Bridge\"" w812 {
          tunnel: [w822 w833 w842] -> w811
          frame Default {
            n561 = property on="Runtime Settings" class="Clust (strict)"() -> ("Value"=w826:T27)  [unwired: 2 in, 2 out]
            n562 = Unbundle By Name(w826) -> ("Read AVS channels from"=w824:i8, "Last Channel"=w825:i8)
            n563 = for {
              N: 10 -> [_]
              tunnel: w825 -> [w828]
              tunnel: w824 -> [w829]
              tunnel: [w827] -> w822 mode=indexing
              i -> [w830]
              n564 = Less Or Equal?(x=w829, y=w830) -> (x <= y?=w832:bool)
              n565 = Less Or Equal?(x=w830, y=w828) -> (x <= y?=w831:bool)
              n566 = And(x=w832, y=w831) -> (x .and. y?=w827:bool)
            }
          }
          frame "Impedance Bridge" {
            n567 = local read "zDll"() -> (w834:path)
            n568 = for {
              N: 10 -> [_]
              tunnel: [w837] -> w835 mode=indexing
              tunnel: w834 -> [w838]
              i -> [w840]
              n569 = call "GetByteParam.vi"("ParNo"=u8 0, "SetNo"=w840, "zDll"=w838) -> ("return type"=w837:u8)  [unwired: 6 in, 2 out]
            }
            n570 = Greater Than 0?(x=w835) -> (x > 0?=w833:bool[])
          }
          frame "AVS47B (RS232 interface)" {
            n571 = local read "Active"() -> (w841:T21)
            n572 = Cluster To Array(cluster=w841) -> (array=w842:bool[])
          }
        }
        n573 = control-ref of="Active"() -> (w818:refnum<vi>)
        n574 = control-ref of="Exc&Ranges"() -> (w814:refnum<vi>)
        n575 = control-ref of="R"() -> (w819:refnum<vi>)
        n576 = control-ref of="Thermometer"() -> (w820:refnum<vi>)
        n577 = control-ref of="T"() -> (w821:refnum<vi>)
        n578 = control-ref of="uPlots"() -> (w815:refnum<vi>)
        n579 = control-ref of="AVS names"() -> (w813:refnum<vi>)
        n580 = control-ref of="zBridge params"() -> (w810:refnum<vi>)
        n581 = control-ref of="Status"() -> (w809:refnum<vi>)
        n582 = control-ref of="Units"() -> (w808:refnum<vi>)
        n583 = control-ref of="AVS names small"() -> (w807:refnum<vi>)
        n584 = control-ref of="Small R"() -> (w806:refnum<vi>)
        n585 = control-ref of="Small T"() -> (w805:refnum<vi>)
        n586 = Build Array(w818, w814, w819, w820, w821, w815, w813, w810, w809, w808, w807, w806, w805) -> (w816:refnum<vi>[])
        n587 = Array Size(array=w816) -> (size(s)=w817:i32)
        n588 = for {
          N: w817 -> [_]
          tunnel: w816 -> [w846] mode=indexing
          tunnel: w811 -> [w843]
          n589 = property class="Clust"(reference=w846) -> ("Controls[]"=w844:refnum<vi>[])  [unwired: 1 in, 2 out]
          n590 = Array Size(array=w844) -> (size(s)=w845:i32)
          n591 = for {
            N: w845 -> [_]
            tunnel: w844 -> [w848] mode=indexing
            tunnel: w843 -> [w847] mode=indexing
            n592 = case shown="True" w847 {
              tunnel: w848 -> [w849 w854]
              frame False {
                n593 = property class="Ctl"(reference=w849, "Disabled"=u8 2) -> ("ClassName"=w850:string)  [unwired: 1 in, 2 out]
                n594 = case shown="\"Boolean\"" w850 {
                  tunnel: w849 -> [_ w853 _]
                  frame "False", Default {
                  }
                  frame "Boolean" {
                    n595 = property class="Ctl"(reference=w853, "Value"=FALSE) -> ()  [unwired: 1 in, 2 out]
                  }
                  frame "Ring" {
                  }
                }
              }
              frame True {
                n596 = property class="Ctl"(reference=w854, "Disabled"=u8 0) -> ("ClassName"=w855:string)  [unwired: 1 in, 2 out]
                n597 = case shown="\"Boolean\"" w855 {
                  tunnel: w854 -> [_ w858]
                  frame "False", Default {
                  }
                  frame "Boolean" {
                    n598 = property class="Ctl"(reference=w858, "Value"=TRUE) -> ()  [unwired: 1 in, 2 out]
                  }
                }
              }
            }
          }
        }
      }
      event "Log path": Value Change {
        # "Modify window title to show measurement information"
        n599 = event-data() -> ("NewVal"=w865:path)  [unwired: 1 in, 5 out]
        n600 = property on="Run description" class="Str"() -> ("Value"=w859:string)  [unwired: 2 in, 2 out]
        n601 = property on="AVS type" class="Enum (strict)"() -> ("RingText.Text"=w860:string)  [unwired: 2 in, 2 out]
        n602 = property on="CS type" class="Enum (strict)"() -> ("RingText.Text"=w863:string)  [unwired: 2 in, 2 out]
        n603 = Path To String(path=w865) -> (string=w862:string)
        n604 = Format Into String(format string="%s - %s - %s   (%s)", w859, w860, w863, w862) -> (resulting string=w861:string)  [unwired: 2 in, 1 out]
        n605 = control-ref of="This VI"() -> (w866:refnum<vi>)
        n606 = property class="VI"(reference=w866, "Front Panel.Title"=w861) -> ()  [unwired: 1 in, 2 out]
      }
      event "Refresh Calibrations", "Bridge settings.AVS_CalFolder": Value Change {
        # "Refresh the list of calibration files"
        n607 = event-data() -> ()  [unwired: 1 in, 3 out]
        n608 = control-ref of="Thermometer"() -> (w873:refnum<vi>)
        n609 = control-ref of="CurCalibrations"() -> (w867:refnum<vi>)
        n610 = control-ref of="AVS_CalFolder"() -> (w871:refnum<vi>)
        n611 = control-ref of="Select sensor 1"() -> (w872:refnum<vi>)
        n612 = control-ref of="Select sensor 1"() -> (w870:refnum<vi>)
        n613 = call "ReloadCalibrations.vi"("error in (no error)"=w869, "Quick convert sensors"=w870, "CurCalibrations"=w867, "Calibration files path"=w871, "Channel1 sensors"=w872, "Channels list"=w873) -> ("error out"=w868:errorcluster)  [unwired: 1 in]
      }
      event Value Change {
        w879 = refnum<vi> refnum  # XYGraph
        # "Show cursor on plot is \"Cursor\" or \"Delete points\" mode is enabled"
        # "!!NOTE:This routine assumes that XY graph is control #0 on tab page!!"
        n614 = event-data() -> ("NewVal"=w875:T7)  [unwired: 1 in, 5 out]
        n615 = property on="Channel Controls" class="TabCtl (strict)"() -> ("Pages"=w883:refnum<vi>[], "Value"=w882:T8)  [unwired: 2 in, 2 out]
        n616 = Index Array(array=w883, index=w882) -> (element=w881:refnum<vi>)
        n617 = property class="Page"(reference=w881) -> ("ControlsOnPage"=w876:refnum<vi>[])  [unwired: 1 in, 2 out]
        n618 = Index Array(array=w876, index=0) -> (element=w880:refnum<vi>)
        n619 = Type Cast(type=w879, x=w880) -> (*(type *) &x=w874:refnum<vi>)
        n620 = case shown="\"Erase range\"" w875 {
          tunnel: w874 -> [w884 w893 w901 w909]
          frame "No Selection", Default {
            n621 = property class="XYGraph"(reference=w884, "Active Cursor"=u32 0, "Cursor.Visible"=FALSE) -> (reference out=w887:refnum<vi>)  [unwired: 1 in, 1 out]
            n622 = property class="XYGraph"(reference=w887, "Active Cursor"=u32 1, "Cursor.Visible"=FALSE) -> ()  [unwired: 1 in, 2 out]
          }
          frame "Erase range" {
            n623 = property class="XYGraph"(reference=w893, "Active Cursor"=u32 0, "Cursor.Visible"=TRUE, "Cursor.Cursor Color"=u32 16777062, "Cursor.Cursor Index"=0, "ActPaletteTool"=0 ("Palette:Active Tool")) -> (reference out=w896:refnum<vi>)  [unwired: 1 in, 1 out]
            n624 = property class="XYGraph"(reference=w896, "Active Cursor"=u32 1, "Cursor.Visible"=TRUE, "Cursor.Cursor Color"=u32 6618880) -> ()  [unwired: 1 in, 2 out]
          }
          frame "Cursor mode" {
            n625 = property class="XYGraph"(reference=w901, "Active Cursor"=u32 0, "Cursor.Visible"=TRUE, "Cursor.Cursor Color"=u32 6618880, "ActPaletteTool"=0 ("Palette:Active Tool")) -> (reference out=w904:refnum<vi>)  [unwired: 1 in, 1 out]
            n626 = property class="XYGraph"(reference=w904, "Active Cursor"=u32 1, "Cursor.Visible"=FALSE) -> ()  [unwired: 1 in, 2 out]
          }
          frame "Erase point" {
            n627 = property class="XYGraph"(reference=w909, "Active Cursor"=u32 0, "Cursor.Visible"=TRUE, "Cursor.Cursor Color"=u32 16777062, "ActPaletteTool"=0 ("Palette:Active Tool")) -> (reference out=w912:refnum<vi>)  [unwired: 1 in, 1 out]
            n628 = property class="XYGraph"(reference=w912, "Active Cursor"=u32 1, "Cursor.Visible"=FALSE) -> ()  [unwired: 1 in, 2 out]
          }
        }
      }
      event "R-Plot 0", "R-Plot 1", "R-Plot 2", "R-Plot 3", "R-Plot 4", "R-Plot 5", "R-Plot 6", "R-Plot 7", "R-Plot 8", "R-Plot 9": Mouse Down? {
        # "Disabled"
        n629 = event-data() -> ("CtlRef"=w917:refnum<vi>, "Button"=w922:u16, "Mods.Double Click"=w919:bool)  [unwired: 1 in, 5 out]
        n630 = Equal?(x=u16 1, y=w922) -> (x = y?=w920:bool)
        n631 = And(x=w920, y=w919) -> (x .and. y?=w918:bool)
        n632 = disable-structure shown="Disabled" {
          disable-tunnel: w918 -> [w925 _]
          disable-tunnel: w917 -> [w924 _]
          disable-tunnel: "Mode Buttons" -> [w923 _]
          frame Disabled {
            n633 = case shown="True" w925 {
              tunnel: w923 -> [_ w927]
              tunnel: w924 -> [_ w926]
              frame False {
              }
              frame True {
                n634 = case shown="\"Erase range\"" w927 {
                  tunnel: w926 -> [_ w928]
                  frame "No Selection", Default {
                  }
                  frame "Erase range" {
                    n635 = property class="XYGraph (strict)"(reference=w928, "ActPaletteTool"=0 ("Palette:Active Tool"), "Active Cursor"=u32 0, "Cursor.Visible"=TRUE) -> ()  [unwired: 1 in, 2 out]
                  }
                }
              }
            }
          }
          frame Enabled {
          }
        }
        n636 = event-data() -> ()  [unwired: 5 in, 1 out]
      }
      event "R-Plot 0", "R-Plot 1", "R-Plot 2", "R-Plot 3", "R-Plot 4", "R-Plot 5", "R-Plot 6", "R-Plot 7", "R-Plot 8", "R-Plot 9": Mouse Down {
        # "Process (double) click on plots in special modes (\"Cursor\", \"Erase\")"
        n637 = event-data() -> ("CtlRef"=w934:refnum<vi>, "Coords"=w937:T69, "Button"=w933:u16, "Mods.Double Click"=w936:bool, "PlatMods"=w932:T70)  [unwired: 1 in, 3 out]
        n638 = property on="Mode Buttons" class="RadioBtnsControl (strict)"() -> ("Value"=w935:T7)  [unwired: 2 in, 2 out]
        n639 = case shown="1" w933 {
          tunnel: w937 -> [_ _ w942]
          tunnel: w936 -> [_ _ w941]
          tunnel: w935 -> [_ _ w940]
          tunnel: w934 -> [_ _ w939]
          tunnel: w932 -> [_ _ _]
          frame 2 {
          }
          frame Default {
          }
          frame 1 {
            n640 = case shown="\"Erase range\"" w940 {
              tunnel: w939 -> [_ w945 w966 w974]
              tunnel: w942 -> [_ w944 w965 w976]
              tunnel: w941 -> [_ w943 w967 w975]
              frame "No Selection", Default {
              }
              frame "Cursor mode" {
                n641 = case shown="True" w943 {
                  tunnel: w945 -> [_ w955]
                  tunnel: w944 -> [_ w953]
                  frame False {
                  }
                  frame True {
                    n642 = invoke class="XYGraph (strict)" method="Map Coords To XY"(reference=w955, "Coords"=w953) -> (reference out=w954:refnum<vi>, "XY"=w952:cluster{"X":dbl, "Y":dbl})  [unwired: 5 in, 5 out]
                    n643 = Unbundle By Name(w952) -> ("X"=w950:dbl)
                    n644 = local read "Data"() -> (w951:T28)
                    n645 = property class="XYGraph (strict)"(reference=w954, "Active Cursor"=u32 0, "Cursor.Cursor Position"=w952) -> ()  [unwired: 1 in, 2 out]
                    n646 = for {
                      tunnel: w951 -> [w964] mode=indexing
                      tunnel: w950 -> [w962]
                      tunnel: [w958] -> w949 mode=indexing
                      tunnel: [w957] -> w948 mode=indexing
                      n647 = Unbundle By Name(w964) -> ("R"=w961:dbl[], "T"=w960:dbl[], "Time"=w963:dbl[])
                      n648 = Threshold 1D Array(2:w962, 3:w963) -> (0:w959:dbl)  [unwired: 1 in]
                      n649 = Index Array(array=w961, index=w959) -> (element=w958:dbl)
                      n650 = Index Array(array=w960, index=w959) -> (element=w957:dbl)
                    }
                    n651 = Array To Cluster(array=w948) -> (cluster=w946:T61)
                    n652 = Array To Cluster(array=w949) -> (cluster=w947:T61)
                    n653 = property on="Time" class="DigNum (strict)"("Value"=w950) -> ()  [unwired: 2 in, 2 out]
                    n654 = property on="Small R" class="Clust (strict)"("Value"=w947) -> ()  [unwired: 2 in, 2 out]
                    n655 = property on="Small T" class="Clust (strict)"("Value"=w946) -> ()  [unwired: 2 in, 2 out]
                  }
                }
              }
              frame "Erase range" {
                n656 = case shown="False" w967 {
                  tunnel: w966 -> [w971 _]
                  tunnel: w965 -> [w970 _]
                  frame False {
                    n657 = invoke class="XYGraph (strict)" method="Map Coords To XY"(reference=w971, "Coords"=w970) -> (reference out=w973:refnum<vi>, "XY"=w968:cluster{"X":dbl, "Y":dbl})  [unwired: 5 in, 5 out]
                    n658 = property class="XYGraph (strict)"(reference=w973, "Active Cursor"=u32 0, "Cursor.Cursor Position"=w968, "Active Cursor"=u32 1, "Cursor.Cursor Position"=w968) -> ()  [unwired: 1 in, 2 out]
                  }
                  frame True {
                  }
                }
              }
              frame "Erase point" {
                n659 = case shown="True" w975 {
                  tunnel: w974 -> [w981 w996]
                  tunnel: w976 -> [w980 _]
                  frame False {
                    n660 = invoke class="XYGraph (strict)" method="Map Coords To XY"(reference=w981, "Coords"=w980) -> (reference out=w979:refnum<vi>, "XY"=w978:cluster{"X":dbl, "Y":dbl})  [unwired: 5 in, 5 out]
                    n661 = property class="XYGraph (strict)"(reference=w979, "Active Cursor"=u32 0, "Cursor.Cursor Position"=w978) -> ()  [unwired: 1 in, 2 out]
                  }
                  frame True {
                    n662 = property class="XYGraph (strict)"(reference=w996, "Active Cursor"=u32 0) -> ("Cursor.Cursor X"=w984:dbl)  [unwired: 1 in, 2 out]
                    n663 = local read "Channel Controls"() -> (w983:T8)
                    n664 = local read "Data"() -> (w982:T28)
                    n665 = Index Array(array=w982, index=w983) -> (element=w989:cluster{"R":dbl[], "T":dbl[], "Time":dbl[]})
                    n666 = Unbundle By Name(w989) -> ("R"=w985:dbl[], "T"=w986:dbl[], "Time"=w987:dbl[])
                    n667 = Threshold 1D Array(2:w984, 3:w987) -> (0:w988:dbl)  [unwired: 1 in]
                    n668 = Delete From Array(array=w985, index=w988) -> (array with subset deleted=w992:dbl[])  [unwired: 1 in, 1 out]
                    n669 = Delete From Array(array=w986, index=w988) -> (array with subset deleted=w991:dbl[])  [unwired: 1 in, 1 out]
                    n670 = Delete From Array(array=w987, index=w988) -> (array with subset deleted=w990:dbl[])  [unwired: 1 in, 1 out]
                    n671 = Bundle By Name(cluster=w989, "R"=w992, "T"=w991, "Time"=w990) -> (w993:cluster{"R":dbl[], "T":dbl[], "Time":dbl[]})
                    n672 = Replace Array Subset(array=w982, new element=w993, index=w983) -> (w994:T28)
                    n673 = local write "Data"(w994) -> ()
                  }
                }
              }
            }
            "LMB Down" <- TRUE ("Mouse down")
          }
        }
      }
      event "R-Plot 0", "R-Plot 1", "R-Plot 2", "R-Plot 3", "R-Plot 4", "R-Plot 5", "R-Plot 6", "R-Plot 7", "R-Plot 8", "R-Plot 9": Mouse Move {
        # "Process mouse movement over plots in special modes (\"Cursor\", \"Erase\")"
        n674 = event-data() -> ("CtlRef"=w998:refnum<vi>, "Coords"=w999:T69)  [unwired: 1 in, 3 out]
        n675 = property on="Mode Buttons" class="RadioBtnsControl (strict)"() -> ("Value"=w1002:T7)  [unwired: 2 in, 2 out]
        n676 = local read "LMB Down"() -> (w1003:bool)
        n677 = Equal?(x=w1002, y=Cursor_Controls."Erase range" ("Mode Buttons")) -> (x = y?=w1000:bool)
        n678 = And(x=w1003, y=w1000) -> (x .and. y?=w1001:bool)
        n679 = case shown="True" w1001 {
          tunnel: w999 -> [_ w1005]
          tunnel: w998 -> [_ w1004]
          frame False {
          }
          frame True {
            n680 = invoke class="XYGraph (strict)" method="Map Coords To XY"(reference=w1004, "Coords"=w1005) -> (reference out=w1008:refnum<vi>, "XY"=w1007:cluster{"X":dbl, "Y":dbl})  [unwired: 5 in, 5 out]
            n681 = property class="XYGraph (strict)"(reference=w1008, "Active Cursor"=u32 1, "Cursor.Cursor Position"=w1007) -> ()  [unwired: 1 in, 2 out]
          }
        }
      }
      event "R-Plot 0", "R-Plot 1", "R-Plot 2", "R-Plot 3", "R-Plot 4", "R-Plot 5", "R-Plot 6", "R-Plot 7", "R-Plot 8", "R-Plot 9": Mouse Up {
        n682 = event-data() -> ("CtlRef"=w1011:refnum<vi>, "Button"=w1009:u16)  [unwired: 1 in, 6 out]
        n683 = property on="Mode Buttons" class="RadioBtnsControl (strict)"() -> ("Value"=w1012:T7)  [unwired: 2 in, 2 out]
        n684 = property class="XYGraph (strict)"(reference=w1011) -> ("ActPaletteTool"=w1010:i32)  [unwired: 1 in, 2 out]
        n685 = case shown="1" w1009 {
          tunnel: w1012 -> [_ w1016]
          tunnel: w1011 -> [_ w1015]
          tunnel: w1010 -> [_ w1014]
          frame Default {
          }
          frame 1 {
            n686 = local read "LMB Down"() -> (w1013:bool)
            n687 = case shown="0" w1014 {
              tunnel: w1016 -> [_ w1021]
              tunnel: w1015 -> [_ w1020]
              tunnel: w1013 -> [_ w1018]
              frame Default {
                n688 = property on="Mode Buttons" class="RadioBtnsControl (strict)"("Val(Sgnl)"=T54."No Selection" ("Value (Signaling)")) -> ()  [unwired: 2 in, 2 out]
              }
              frame 0 {
                n689 = Equal?(x=w1021, y=T54."Erase range") -> (x = y?=w1024:bool)
                n690 = And(x=w1018, y=w1024) -> (x .and. y?=w1023:bool)
                n691 = case shown="True" w1023 {
                  tunnel: w1020 -> [_ w1047]
                  frame False {
                  }
                  frame True {
                    n692 = local read "Channel Controls"() -> (w1046:T8)
                    n693 = property class="XYGraph (strict)"(reference=w1047, "Active Cursor"=u32 0, "Active Cursor"=u32 1) -> ("Cursor.Cursor X"=w1044:dbl, "Cursor.Cursor X"=w1025:dbl)  [unwired: 1 in, 2 out]
                    n694 = local read "Data"() -> (w1041:T28)
                    n695 = Max & Min(x=w1044, y=w1025) -> (max(x,y)=w1034:dbl, min(x,y)=w1027:dbl)
                    n696 = Index Array(array=w1041, index=w1046) -> (element=w1037:cluster{"R":dbl[], "T":dbl[], "Time":dbl[]})
                    n697 = Unbundle By Name(w1037) -> ("R"=w1035:dbl[], "T"=w1036:dbl[], "Time"=w1033:dbl[])
                    n698 = Threshold 1D Array(2:w1034, 3:w1033) -> (0:w1031:dbl)  [unwired: 1 in]
                    n699 = Threshold 1D Array(2:w1027, 3:w1033) -> (0:w1032:dbl)  [unwired: 1 in]
                    n700 = Subtract(x=w1031, y=w1032) -> (x-y=w1030:dbl)
                    n701 = Delete From Array(array=w1035, length=w1030, index=w1032) -> (array with subset deleted=w1040:dbl[])  [unwired: 1 out]
                    n702 = Delete From Array(array=w1036, length=w1030, index=w1032) -> (array with subset deleted=w1039:dbl[])  [unwired: 1 out]
                    n703 = Delete From Array(array=w1033, length=w1030, index=w1032) -> (array with subset deleted=w1038:dbl[])  [unwired: 1 out]
                    n704 = Bundle By Name(cluster=w1037, "R"=w1040, "T"=w1039, "Time"=w1038) -> (w1042:cluster{"R":dbl[], "T":dbl[], "Time":dbl[]})
                    n705 = Replace Array Subset(array=w1041, new element=w1042, index=w1046) -> (w1043:T28)
                    n706 = local write "Data"(w1043) -> ()
                    n707 = property class="XYGraph (strict)"(reference=w1047, "Active Cursor"=u32 0, "Cursor.Cursor X"=w1027, "Active Cursor"=u32 1, "Cursor.Cursor X"=w1027) -> ()  [unwired: 1 in, 2 out]
                  }
                }
                n708 = local write "LMB Down"(FALSE ("Mouse down")) -> ()
              }
            }
          }
        }
      }
      event "R-Plot 0", "R-Plot 1", "R-Plot 2", "R-Plot 3", "R-Plot 4", "R-Plot 5", "R-Plot 6", "R-Plot 7", "R-Plot 8", "R-Plot 9": Mouse Leave {
        n709 = event-data() -> ()  [unwired: 1 in, 4 out]
        n710 = local write "LMB Down"(FALSE ("Mouse down")) -> ()
      }
      event "R-Plot 0", "R-Plot 1", "R-Plot 2", "R-Plot 3", "R-Plot 4", "R-Plot 5", "R-Plot 6", "R-Plot 7", "R-Plot 8", "R-Plot 9": Scale Range Change {
        w1050 = u8 0 ("X Scale.Scale Fit")
        # "Disable plot autoscaling if the user has changed the scale of the plot manualy"
        n711 = event-data() -> ("CtlRef"=w1049:refnum<vi>)  [unwired: 1 in, 7 out]
        n712 = property class="XYGraph (strict)"(reference=w1049, "XScale.ScaleFit"=w1050, "YScale.ScaleFit"=w1050) -> ()  [unwired: 1 in, 2 out]
      }
      event "R-Plot 0", "R-Plot 1", "R-Plot 2", "R-Plot 3", "R-Plot 4", "R-Plot 5", "R-Plot 6", "R-Plot 7", "R-Plot 8", "R-Plot 9": Shortcut Menu Activation? {
        w1058 = string[] ["Log Y"] ("item names")
        w1060 = string[] ["Zoom In to Last Data", "Autoscale XY"] ("item names")
        # "Add extra options to the plots context menu"
        n713 = event-data() -> ("MenuRef"=w1062:refnum<k9>, "CtlRef"=w1054:refnum<vi>)  [unwired: 1 in]
        n714 = Insert Menu Items(4:10, 7:w1060, 8:w1060, 9:w1062) -> (3:w1056:refnum<k9>)  [unwired: 2 in, 2 out]
        n715 = property class="XYGraph (strict)"(reference=w1054) -> ("YScale.Mapping Mode"=w1053:u8)  [unwired: 1 in, 2 out]
        n716 = Insert Menu Items(4:14, 7:w1058, 8:w1058, 9:w1056) -> (3:w1055:refnum<k9>)  [unwired: 2 in, 2 out]
        n717 = Not Equal To 0?(x=w1053) -> (x != 0?=w1052:bool)
        n718 = Set Menu Item Info(6:w1052, 7:"Log Y", 11:w1055) -> ()  [unwired: 4 in, 2 out]
        n719 = local read "LMB Down"() -> (w1059:bool)
        n720 = event-data("Discard?"=w1059) -> ()  [unwired: 1 in, 1 out]
      }
      event "R-Plot 0", "R-Plot 1", "R-Plot 2", "R-Plot 3", "R-Plot 4", "R-Plot 5", "R-Plot 6", "R-Plot 7", "R-Plot 8", "R-Plot 9": Shortcut Menu Selection (User) {
        # "Zoom in to last \"Miniplot points\". Zoom out a bit to have some space around the points"
        n721 = event-data() -> ("CtlRef"=w1066:refnum<vi>, "ItemTag"=w1064:string)  [unwired: 1 in]
        n722 = Type Cast(type=refnum<vi> refnum ("R-Plot 0"), x=w1066) -> (*(type *) &x=w1065:refnum<vi>)
        n723 = case shown="\"Zoom In to Last Data\"" w1064 {
          tunnel: w1065 -> [_ w1068 w1097 w1103]
          frame Default {
          }
          frame "Autoscale XY" {
            w1067 = u8 2 ("X Scale.Scale Fit")
            n724 = property class="XYGraph (strict)"(reference=w1068, "XScale.ScaleFit"=w1067, "YScale.ScaleFit"=w1067) -> ()  [unwired: 1 in, 2 out]
          }
          frame "Zoom In to Last Data" {
            w1093 = u8 0 ("Y Scale.Scale Fit")
            n725 = property on="Runtime Settings" class="Clust (strict)"() -> ("Value"=w1092:T27)  [unwired: 2 in, 2 out]
            n726 = property class="XYGraph (strict)"(reference=w1097) -> (reference out=w1094:refnum<vi>, "Value"=w1096:cluster{dbl[], dbl[]})  [unwired: 1 in, 1 out]
            n727 = Unbundle By Name(w1092) -> ("Data Memory 2"=w1091:dbl)
            n728 = Unbundle(w1096) -> (w1070:dbl[], w1095:dbl[])
            n729 = Multiply(x=w1091, y=60.0) -> (x*y=w1087:dbl)
            n730 = Reverse 1D Array(array=w1070) -> (reversed array=w1075:dbl[])
            n731 = Reverse 1D Array(array=w1095) -> (reversed array=w1083:dbl[])
            n732 = Index Array(array=w1075) -> (element=w1089:dbl)  [unwired: 1 in]
            n733 = Multiply(x=0.5, y=w1087) -> (x*y=w1088:dbl)
            n734 = Add(x=w1088, y=w1089) -> (x+y=w1086:dbl)
            n735 = Subtract(x=w1089, y=w1087) -> (x-y=w1084:dbl)
            n736 = call "Improved Threshold Detector.71.vi"("Threshold"=w1084, "Array"=w1070) -> ("Positive transition indices"=w1071:i32[])  [unwired: 8 in, 1 out]
            n737 = Index Array(array=w1071) -> (element=w1098:i32)  [unwired: 1 in]
            n738 = Array Size(array=w1070) -> (size(s)=w1073:i32)
            n739 = Index Array(array=w1070, index=w1098) -> (element=w1069:dbl)
            n740 = Subtract(x=w1073, y=w1098) -> (x-y=w1072:i32)
            n741 = Array Subset(array=w1083, length=w1072) -> (w1082:dbl[])  [unwired: 1 in]
            n742 = Array Max & Min(array=w1082) -> (max value=w1079:dbl, min value=w1078:dbl)  [unwired: 2 out]
            n743 = Subtract(x=w1079, y=w1078) -> (x-y=w1081:dbl)
            n744 = Divide(x=w1081, y=2.0) -> (x/y=w1077:dbl)
            n745 = Add(x=w1079, y=w1077) -> (x+y=w1074:dbl)
            n746 = Subtract(x=w1078, y=w1077) -> (x-y=w1076:dbl)
            n747 = property class="XYGraph (strict)"(reference=w1094, "XScale.ScaleFit"=w1093, "YScale.ScaleFit"=w1093, "XScale.Maximum"=w1086, "XScale.Minimum"=w1069, "YScale.Maximum"=w1074, "YScale.Minimum"=w1076) -> ()  [unwired: 1 in, 2 out]
          }
          frame "Log Y" {
            n748 = property class="XYGraph (strict)"(reference=w1103) -> (reference out=w1102:refnum<vi>, "YScale.Mapping Mode"=w1101:u8)  [unwired: 1 in, 1 out]
            n749 = Equal To 0?(x=w1101) -> (x = 0?=w1100:bool)
            n750 = Boolean To (0,1)(Boolean=w1100) -> (0, 1=w1099:i16)
            n751 = property class="XYGraph (strict)"(reference=w1102, "YScale.Mapping Mode"=w1099) -> ()  [unwired: 1 in, 2 out]
          }
        }
      }
      event "uPlots.uPlot 0", "uPlots.uPlot 1", "uPlots.uPlot 2", "uPlots.uPlot 3", "uPlots.uPlot 4", "uPlots.uPlot 5", "uPlots.uPlot 6", "uPlots.uPlot 7", "uPlots.uPlot 8", "uPlots.uPlot 9": Mouse Down {
        # "Switch to big plot on double click on small plot"
        n752 = event-data() -> ("Mods.Double Click"=w1105:bool, "CtlRef"=w1104:refnum<vi>)  [unwired: 1 in]
        n753 = case shown="True" w1105 {
          tunnel: w1104 -> [_ w1108]
          frame False {
          }
          frame True {
            n754 = property class="XYGraph (strict)"(reference=w1108) -> ("Label.Text"=w1109:string)  [unwired: 1 in, 2 out]
            n755 = Reverse String(1:w1109) -> (0:w1110:string)
            n756 = Decimal String To Number(string=w1110, default (0L)=8 ("default (0 I32)")) -> (number=w1107:i32)  [unwired: 1 in, 1 out]
            n757 = property on="Channel Controls" class="TabCtl (strict)"("Val(Sgnl)"=w1107) -> ()  [unwired: 2 in, 2 out]
          }
        }
      }
      event "Erase all": Value Change {
        # "Clear data array.\nReset PID."
        n758 = event-data() -> ()  [unwired: 1 in, 6 out]
        n759 = local read "Channel Controls"() -> (w1113:T8)
        n760 = local read "Data"() -> (w1114:T28)
        n761 = Replace Array Subset(array=w1114, new element=cluster{"R":dbl[], "T":dbl[], "Time":dbl[]} {"R"=[], "T"=[], "Time"=[]} ("new element/subarray"), index=w1113) -> (w1112:T28)
        n762 = local write "Data"(w1112) -> ()
        n763 = disable-structure shown="Disabled" {
          frame Disabled {
            n764 = Initialize Array(cluster{"R":dbl[], "T":dbl[], "Time":dbl[]} {"R"=[], "T"=[], "Time"=[]}, 10 ("dimension size")) -> ()  [unwired: 1 out]
          }
          frame Enabled {
          }
        }
      }
      event "Clear all plots": Value Change {
        n765 = event-data() -> ()  [unwired: 1 in, 6 out]
        n766 = Initialize Array(cluster{"R":dbl[], "T":dbl[], "Time":dbl[]} {"R"=[], "T"=[], "Time"=[]}, 10 ("dimension size")) -> (w1118:cluster{"R":dbl[], "T":dbl[], "Time":dbl[]}[])
        n767 = local write "Data"(w1118) -> ()
      }
      event "Bridge settings.AVS type": Value Change {
        # "Select bridge type (AVS/zBridge). Show/hide corresponding controls."
        n768 = event-data() -> ("NewVal"=w1121:T60)  [unwired: 1 in, 5 out]
        n769 = flat-sequence {
          tunnel: w1121 -> [w1130]
          frame #0 {
            w1126 = u8 0 ("Disabled")
            w1129 = u8 0 ("Disabled")
            w1128 = FALSE ("Visible")
            w1127 = u8 2 ("Disabled")
            n770 = property on="AVS_SPort" class="VISAName"("Visible"=w1128, "Disabled"=w1127) -> ()  [unwired: 2 in, 2 out]
            n771 = property on="zBridge settings" class="Bool"("Visible"=w1128, "Disabled"=w1127) -> ()  [unwired: 2 in, 2 out]
            n772 = property on="Tab Control 5" class="TabCtl (strict)"("Disabled"=w1126) -> ()  [unwired: 2 in, 2 out]
            n773 = property on="Address" class="VISAName"("Visible"=w1128, "Disabled"=w1127) -> ()  [unwired: 2 in, 2 out]
            n774 = property on="Tab Control" class="TabCtl (strict)"("Disabled"=w1126) -> ()  [unwired: 2 in, 2 out]
            n775 = property on="Read AVS channels from" class="DigNum (strict)"("Disabled"=w1129) -> ()  [unwired: 2 in, 2 out]
            n776 = property on="Last Channel" class="DigNum (strict)"("Disabled"=w1129) -> ()  [unwired: 2 in, 2 out]
            n777 = property on="Stabilisation Delay" class="DigNum (strict)"("Disabled"=w1129) -> ()  [unwired: 2 in, 2 out]
            n778 = property on="Averages" class="DigNum (strict)"("Disabled"=w1129) -> ()  [unwired: 2 in, 2 out]
            n779 = property on="Delay Between Scans" class="DigNum (strict)"("Disabled"=w1129) -> ()  [unwired: 2 in, 2 out]
            n780 = call "Build ranges list.vi"("Values"="-1\r\n0\r\n1\r\n2\r\n3\r\n4\r\n5\r\n6\r\n7", "Strings"="n.a.\r\nopen\r\n2 Ohm\r\n20 Ohm\r\n200 Ohm\r\n2k Ohm\r\n20k Ohm\r\n200k Ohm\r\n2M Ohm") -> ("Strings and Values"=w1125:cluster{"String":string, "Value":i32}[])  [unwired: 4 in]
            n781 = property on="Range 0" class="Ring (strict)"("StringsAndValues[]"=w1125) -> ()  [unwired: 2 in, 2 out]
            n782 = property on="Range 0" class="Ring (strict)"("StringsAndValues[]"=w1125) -> ()  [unwired: 2 in, 2 out]
            n783 = property on="Range 0" class="Ring (strict)"("StringsAndValues[]"=w1125) -> ()  [unwired: 2 in, 2 out]
            n784 = property on="Range 0" class="Ring (strict)"("StringsAndValues[]"=w1125) -> ()  [unwired: 2 in, 2 out]
            n785 = property on="Range 0" class="Ring (strict)"("StringsAndValues[]"=w1125) -> ()  [unwired: 2 in, 2 out]
            n786 = property on="Range 0" class="Ring (strict)"("StringsAndValues[]"=w1125) -> ()  [unwired: 2 in, 2 out]
            n787 = property on="Range 0" class="Ring (strict)"("StringsAndValues[]"=w1125) -> ()  [unwired: 2 in, 2 out]
            n788 = property on="Range 0" class="Ring (strict)"("StringsAndValues[]"=w1125) -> ()  [unwired: 2 in, 2 out]
          }
          frame #1 {
            n789 = case shown="\"AVS48SI (RS232 interface)\"" w1130 {
              frame "AVS47A (GPIB interface)" {
                n790 = local write "Scan Parameters"(enum32{"Page 1", "Page 2"}."Page 1" ("Scan Parameters")) -> ()
                n791 = property on="Address" class="VISAName"("Visible"=TRUE, "Disabled"=u8 0) -> ()  [unwired: 2 in, 2 out]
              }
              frame "AVS47B (RS232 interface)" {
                w1134 = u8 2 ("Disabled")
                n792 = local write "Scan Parameters"(enum32{"Page 1", "Page 2"}."Page 1" ("Scan Parameters")) -> ()
                n793 = property on="AVS_SPort" class="VISAName"("Visible"=TRUE, "Disabled"=u8 0) -> ()  [unwired: 2 in, 2 out]
                n794 = property on="Read AVS channels from" class="DigNum (strict)"("Disabled"=w1134) -> ()  [unwired: 2 in, 2 out]
                n795 = property on="Last Channel" class="DigNum (strict)"("Disabled"=w1134) -> ()  [unwired: 2 in, 2 out]
              }
              frame "AVS48SI (RS232 interface)" {
                w1141 = u8 2 ("Disabled")
                n796 = property on="Read AVS channels from" class="DigNum (strict)"("Disabled"=w1141) -> ()  [unwired: 2 in, 2 out]
                n797 = property on="Last Channel" class="DigNum (strict)"("Disabled"=w1141) -> ()  [unwired: 2 in, 2 out]
                n798 = property on="AVS_SPort" class="VISAName"("Visible"=TRUE, "Disabled"=u8 0) -> ()  [unwired: 2 in, 2 out]
                n799 = local write "Scan Parameters"(enum32{"Page 1", "Page 2"}."Page 1" ("Scan Parameters")) -> ()
                n800 = call "Build ranges list.vi"("Values"="-1\r\n0\r\n1\r\n2\r\n3\r\n4\r\n5\r\n6\r\n7", "Strings"="n.a.\r\n3 Ohm\r\n30 Ohm\r\n300 Ohm\r\n3k Ohm\r\n30k Ohm\r\n300k Ohm\r\n3M Ohm\r\n30m Ohm") -> ("Strings and Values"=w1139:cluster{"String":string, "Value":i32}[])  [unwired: 4 in]
                n801 = property on="Range 0" class="Ring (strict)"("StringsAndValues[]"=w1139) -> ()  [unwired: 2 in, 2 out]
                n802 = property on="Range 0" class="Ring (strict)"("StringsAndValues[]"=w1139) -> ()  [unwired: 2 in, 2 out]
                n803 = property on="Range 0" class="Ring (strict)"("StringsAndValues[]"=w1139) -> ()  [unwired: 2 in, 2 out]
                n804 = property on="Range 0" class="Ring (strict)"("StringsAndValues[]"=w1139) -> ()  [unwired: 2 in, 2 out]
                n805 = property on="Range 0" class="Ring (strict)"("StringsAndValues[]"=w1139) -> ()  [unwired: 2 in, 2 out]
                n806 = property on="Range 0" class="Ring (strict)"("StringsAndValues[]"=w1139) -> ()  [unwired: 2 in, 2 out]
                n807 = property on="Range 0" class="Ring (strict)"("StringsAndValues[]"=w1139) -> ()  [unwired: 2 in, 2 out]
                n808 = property on="Range 0" class="Ring (strict)"("StringsAndValues[]"=w1139) -> ()  [unwired: 2 in, 2 out]
              }
              frame "AVS Emulation" {
                n809 = local write "Scan Parameters"(enum32{"Page 1", "Page 2"}."Page 1" ("Scan Parameters")) -> ()
              }
              frame "Impedance Bridge" {
                w1148 = u8 2 ("Disabled")
                n810 = local write "Scan Parameters"(enum32{"Page 1", "Page 2"}."Page 2" ("Scan Parameters")) -> ()
                n811 = property on="zBridge settings" class="Bool"("Visible"=TRUE, "Disabled"=u8 0) -> ()  [unwired: 2 in, 2 out]
                n812 = property on="Read AVS channels from" class="DigNum (strict)"("Disabled"=w1148) -> ()  [unwired: 2 in, 2 out]
                n813 = property on="Last Channel" class="DigNum (strict)"("Disabled"=w1148) -> ()  [unwired: 2 in, 2 out]
                n814 = property on="Stabilisation Delay" class="DigNum (strict)"("Disabled"=w1148) -> ()  [unwired: 2 in, 2 out]
                n815 = property on="Averages" class="DigNum (strict)"("Disabled"=w1148) -> ()  [unwired: 2 in, 2 out]
                n816 = property on="Delay Between Scans" class="DigNum (strict)"("Disabled"=w1148) -> ()  [unwired: 2 in, 2 out]
              }
              frame "Disabled", Default {
                w1150 = u8 2 ("Disabled")
                n817 = property on="Tab Control 5" class="TabCtl (strict)"("Disabled"=w1150) -> ()  [unwired: 2 in, 2 out]
                n818 = property on="Tab Control" class="TabCtl (strict)"("Disabled"=w1150) -> ()  [unwired: 2 in, 2 out]
              }
            }
          }
        }
      }
      event "Runtime Settings.Plot type": Value Change {
        # "Iterate through first 10 pages (plots only)"
        # "Switch between RxTime and TxTime plots"
        n819 = event-data() -> ("NewVal"=w1160:enum16{"R vs Time", "T vs Time"})  [unwired: 1 in, 5 out]
        n820 = Unbundle By Name(w1152) -> ("Reset PID loop"=w1151:refnum<user-event>)
        n821 = Equal To 0?(x=w1160) -> (x = 0?=w1159:bool)
        n822 = Select(t=u32 10532351, s=w1159, f=u32 16711680) -> (s? t:f=w1156:u32)
        n823 = property on="uPlots" class="Clust (strict)"() -> ("Controls[]"=w1154:refnum<vi>[])  [unwired: 2 in, 2 out]
        n824 = property on="Channel Controls" class="TabCtl (strict)"() -> ("Pages"=w1161:refnum<vi>[])  [unwired: 2 in, 2 out]
        n825 = for {
          N: 10 -> [_]
          tunnel: w1161 -> [w1171] mode=indexing
          tunnel: w1156 -> [w1164]
          tunnel: w1154 -> [w1162] mode=indexing
          # "!!NOTE:This routine assumes that graph is control #0 on page!!"
          n826 = property class="Page"(reference=w1171) -> ("ControlsOnPage"=w1169:refnum<vi>[])  [unwired: 1 in, 2 out]
          n827 = Type Cast(type=refnum<vi> refnum ("R-Plot 0"), x=w1162) -> (*(type *) &x=w1163:refnum<vi>)
          n828 = Index Array(array=w1169, index=0) -> (element=w1167:refnum<vi>)
          n829 = Type Cast(type=refnum<vi> refnum ("R-Plot 0"), x=w1167) -> (*(type *) &x=w1166:refnum<vi>)
          n830 = property class="XYGraph (strict)"(reference=w1166, "Plot.Plot Color"=w1164, "Plot.Fill/Pt. Color"=w1164) -> ()  [unwired: 1 in, 2 out]
          n831 = property class="XYGraph (strict)"(reference=w1163, "Plot.Plot Color"=w1164, "Plot.Fill/Pt. Color"=w1164) -> ()  [unwired: 1 in, 2 out]
        }
        n832 = Generate User Event(user event=w1151, event data cluster="" ("event data")) -> ()  [unwired: 2 in, 2 out]
      }
      event "Runtime Settings.Read AVS channels from", "Runtime Settings.Last Channel": Value Change {
        # "Change enabled channels for the AVS bridge"
        n833 = event-data() -> ()  [unwired: 1 in, 6 out]
        n834 = Unbundle By Name(w1173) -> ("UpdateChannelInfo"=w1172:refnum<user-event>)
        n835 = Generate User Event(user event=w1172, event data cluster=bool[] [] ("event data")) -> ()  [unwired: 2 in, 2 out]
      }
      event "Runtime Settings.Filter graphs:": Value Change {
        # "Graph filtering controls"
        n836 = event-data() -> ("NewVal"=w1175:bool)  [unwired: 1 in, 5 out]
        n837 = call "IsDisabled.vi"("Enabled?"=w1175) -> ("Numeric"=w1176:i16)
        n838 = property on="Y_min" class="DigNum (strict)"("Disabled"=w1176) -> ()  [unwired: 2 in, 2 out]
        n839 = property on="Y_max" class="DigNum (strict)"("Disabled"=w1176) -> ()  [unwired: 2 in, 2 out]
      }
      event "Channel Controls": Value Change {
        # "Show hide bottom Impedance/Temperature panel depending on the current tab page"
        n840 = event-data() -> ("NewVal"=w1178:T8)  [unwired: 1 in, 5 out]
        n841 = case shown="\"All\", \"PID loop\"" w1178 {
          tunnel: [TRUE ("Visible") FALSE ("Visible")] -> w1177
          frame Default {
            n842 = property on="Mode Buttons" class="RadioBtnsControl (strict)"() -> ("Value"=w1180:T7)  [unwired: 2 in, 2 out]
            n843 = property on="Data History" class="TabCtl (strict)"("Value"=enum32{"History", "Settings"}."History" ("Data History")) -> ()  [unwired: 2 in, 2 out]
            n844 = property on="Mode Buttons" class="RadioBtnsControl (strict)"("Val(Sgnl)"=w1180) -> ()  [unwired: 2 in, 2 out]
          }
          frame "All", "PID loop" {
            n845 = property on="Data History" class="TabCtl (strict)"("Value"=enum32{"History", "Settings"}."Settings" ("Data History")) -> ()  [unwired: 2 in, 2 out]
          }
        }
        n846 = property on="Graph controls" class="TabCtl (strict)"("Visible"=w1177) -> ()  [unwired: 2 in, 2 out]
      }
      event Value Change {
        # "Calibration changed - update calibrations list"
        n847 = event-data() -> ()  [unwired: 1 in, 6 out]
        n848 = property on="Thermometer" class="Clust (strict)"() -> ("Controls[]"=w1186:refnum<vi>[])  [unwired: 2 in, 2 out]
        n849 = Array Size(array=w1186) -> (size(s)=w1187:i32)
        n850 = for {
          N: w1187 -> [_]
          tunnel: w1186 -> [w1191] mode=indexing
          tunnel: [w1188] -> w1185 mode=indexing
          w1190 = refnum<vi> refnum  # Ring
          n851 = Type Cast(type=w1190, x=w1191) -> (*(type *) &x=w1189:refnum<vi>)
          n852 = property class="Ring"(reference=w1189) -> ("RingText.Text"=w1188:string)  [unwired: 1 in, 2 out]
        }
        n853 = Array To Cluster(array=w1185) -> (cluster=→"CurCalibrations":T33)
      }
      event "Data logging": Value Change {
        # "Log file settings changed. Generate new log file name"
        n854 = event-data() -> ()  [unwired: 1 in, 3 out]
        n855 = local read "Data logging"() -> (w1199:T37)
        n856 = Unbundle By Name(w1199) -> ("Run description"=w1193:string, "Filenames suffix"=w1194:string, "AVS_Path"=w1200:path, "AVS_FName"=w1198:string, "CAL_FName"=w1197:string)
        n857 = local write "LogFileCreationTime"(timestamp(2742897600 s since 1904-01-01)) -> ()
        n858 = call "MGI Make String Filesafe.vi"("String In"=w1193) -> ("Filesafe String Out"=w1192:string)
        n859 = call "GeneratePaths.vi"("Filename Suffix"=w1194, "Run description"=w1192, "AVS_Path"=w1200, "AVS_FName"=w1198, "CAL_Path"=w1200, "CAL_FName"=w1197) -> ("Generated Log path"=w1196:path, "Generated Calib path"=w1195:path)  [unwired: 8 in]
        n860 = local write "Log path"(w1196) -> ()
        n861 = local write "Calib path"(w1195) -> ()
      }
      event "Convert": Mouse Down; "QuickR": Value Change {
        # "Quick convert R->T"
        n862 = event-data() -> ()  [unwired: 1 in, 4 out]
        n863 = property on="Select sensor 1" class="Ring (strict)"() -> ("Strings []"=w1204:string[], "Value"=w1205:u16)  [unwired: 2 in, 2 out]
        n864 = property on="AVS_CalFolder" class="Path"() -> ("Value"=w1202:path)  [unwired: 2 in, 2 out]
        n865 = Index Array(array=w1204, index=w1205) -> (element=w1203:string)
        n866 = call "SelectSensor-txt no ext.vi"("Path"=w1202, "Resistance"="QuickR", "Select sensor"=w1203) -> ("Temperature"=→"T7":dbl)  [unwired: 1 out]
      }
      event "T Sweep.Current": Value Change {
        # "Current/ Setpoint value is changed"
        n867 = event-data() -> ("NewVal"=→"I3_SetPnt":dbl)  [unwired: 1 in, 5 out]
        n868 = Unbundle By Name(w1209) -> ("Reset PID loop"=w1208:refnum<user-event>)
        n869 = Generate User Event(user event=w1208, event data cluster="" ("event data")) -> ()  [unwired: 2 in, 2 out]
      }
      event "Automode 2": Value Change {
        n870 = event-data() -> ("NewVal"=w1212:bool)  [unwired: 1 in, 5 out]
        n871 = case shown="True" w1212 {
          frame False {
          }
          frame True {
            # "Set timer to zero (01-01-1904) so the first point is set immediately, w/o wainting for time delay."
            # "If automatic mode is enabled- fire TempStabilized event to record current R,T,I values and start sweeping through TCS channels arrays"
            n872 = disable-structure shown="Disabled" {
              frame Disabled {
                n873 = Generate User Event(event data cluster="" ("event data")) -> ()  [unwired: 3 in, 2 out]
                "Time Old" <- 0.0 ("Timer")
              }
              frame Enabled {
              }
            }
          }
        }
      }
      event Value Change {
        w1215 = FALSE ("Value (Signaling)")
        # "Changed Channel1 automatic mode"
        n874 = event-data() -> ("NewVal"=w1217:T39)  [unwired: 1 in, 5 out]
        n875 = Unbundle By Name(w1219) -> ("TempStabilized"=w1218:refnum<user-event>)
        n876 = property on="Mode1 ON" class="Bool (strict)"("Val(Sgnl)"=w1215) -> ()  [unwired: 2 in, 2 out]
        n877 = property on="Mode2 ON" class="Bool (strict)"("Val(Sgnl)"=w1215) -> ()  [unwired: 2 in, 2 out]
        n878 = case shown="\"Manual\"" w1217 {
          tunnel: [FALSE ("Automatic mode ON") TRUE ("Automatic mode ON") TRUE ("Automatic mode ON")] -> w1220
          tunnel: w1218 -> [_ w1230 _]
          tunnel: [0 1 2] -> w1216
          frame "Manual" {
            # "Set manual mode currents \nequal to last automode \nvalues."
            n879 = local read "I_in"() -> (w1223:T23[])
            n880 = Index Array(array=w1223) -> (element #1=w1227:T23, element #2=w1226:T23, element #3=w1225:T23, element #4=w1224:T23)  [unwired: 4 in]
            n881 = property on="I" class="DigNum (strict)"("Val(Sgnl)"=w1227) -> ()  [unwired: 2 in, 2 out]
            n882 = property on="I" class="DigNum (strict)"("Val(Sgnl)"=w1226) -> ()  [unwired: 2 in, 2 out]
            n883 = property on="I" class="DigNum (strict)"("Val(Sgnl)"=w1225) -> ()  [unwired: 2 in, 2 out]
            n884 = property on="I" class="DigNum (strict)"("Val(Sgnl)"=w1224) -> ()  [unwired: 2 in, 2 out]
          }
          frame "Mode 1" {
            # "Set automatic mode currents equal to last manual values."
            n885 = local read "I"() -> (w1233:dbl[])
            n886 = Multiply(x=1000.0, y=w1233) -> (x*y=w1231:dbl[])
            n887 = local write "I_in"(w1231) -> ()
            n888 = Generate User Event(user event=w1230, event data cluster=FALSE ("event data")) -> ()  [unwired: 2 in, 2 out]
          }
          frame "Mode2" {
            # "Set automatic mode currents equal to last manual values."
            n889 = local read "I"() -> (w1238:dbl[])
            n890 = Multiply(x=1000.0, y=w1238) -> (x*y=w1236:dbl[])
            n891 = local write "I_in"(w1236) -> ()
          }
        }
        "Automatic mode 1" <- w1220
        "Automatic mode 2" <- w1220
        "Automatic mode 3" <- w1220
        "Automatic mode 0" <- w1220
        n892 = property on="CS modes" class="TabCtl (strict)"("Value"=w1216) -> ()  [unwired: 2 in, 2 out]
      }
      event "Mode1 ON", "Mode2 ON": Value Change {
        n893 = event-data() -> ("NewVal"=w1241:bool)  [unwired: 1 in, 5 out]
        n894 = case shown="True" w1241 {
          frame False {
          }
          frame True {
            w1242 = TRUE
            # "Switch on the current sources."
            n895 = property on="ON" class="Bool (strict)"() -> ("Value"=w1246:bool)  [unwired: 2 in, 2 out]
            n896 = property on="ON" class="Bool (strict)"() -> ("Value"=w1245:bool)  [unwired: 2 in, 2 out]
            n897 = property on="ON" class="Bool (strict)"() -> ("Value"=w1244:bool)  [unwired: 2 in, 2 out]
            n898 = property on="ON" class="Bool (strict)"() -> ("Value"=w1243:bool)  [unwired: 2 in, 2 out]
            n899 = Exclusive Or(1:w1246, 2:w1242) -> (0:w1250:bool)
            n900 = Exclusive Or(1:w1245, 2:w1242) -> (0:w1248:bool)
            n901 = Exclusive Or(1:w1244, 2:w1242) -> (0:w1247:bool)
            n902 = Exclusive Or(1:w1243, 2:w1242) -> (0:w1249:bool)
            n903 = property on="Toggle ON/OFF" class="Bool (strict)"("Value"=w1250) -> ()  [unwired: 2 in, 2 out]
            n904 = property on="Toggle ON/OFF" class="Bool (strict)"("Value"=w1248) -> ()  [unwired: 2 in, 2 out]
            n905 = property on="Toggle ON/OFF" class="Bool (strict)"("Value"=w1247) -> ()  [unwired: 2 in, 2 out]
            n906 = property on="Toggle ON/OFF" class="Bool (strict)"("Value"=w1249) -> ()  [unwired: 2 in, 2 out]
          }
        }
      }
      event "Next step": Value Change {
        # "Go to next step in CS auto mode."
        n907 = event-data() -> ()  [unwired: 1 in, 6 out]
        n908 = Unbundle By Name(w1252) -> ("TempStabilized"=w1251:refnum<user-event>)
        n909 = flat-sequence {
          tunnel: w1251 -> [w1254]
          frame #0 {
            n910 = call "Current Time(double).vi"() -> ("Current Time (double)"=w1253:dbl)  [unwired: 6 in, 1 out]
            n911 = local write "Time Old"(w1253) -> ()
          }
          frame #1 {
            n912 = Generate User Event(user event=w1254, event data cluster=TRUE ("event data")) -> ()  [unwired: 2 in, 2 out]
          }
        }
      }
      event "Data logging.External VI path": Value Change {
        # "Set path for the external VI to call on TempStabilised event"
        n913 = event-data() -> ("NewVal"=w1257:path)  [unwired: 1 in, 5 out]
        n914 = vi-ref "OnTempStabilizedRef.vi"() -> (w1258:refnum<vi>)
        n915 = Open VI Reference(type specifier VI Refnum (for type only)=w1258, vi path=w1257) -> (vi reference=w1256:refnum<vi>)  [unwired: 4 in, 1 out]
        n916 = local write "vi reference"(w1256) -> ()
      }
      event "Autorange": Value Change {
        # "Disabled"
        n917 = event-data() -> ("NewVal"=w1259:bool)  [unwired: 1 in, 5 out]
        n918 = Boolean To (0,1)(Boolean=w1259) -> (0, 1=w1262:i16)
        n919 = Multiply(x=i16 2, y=w1262) -> (x*y=w1260:i16)
        n920 = property on="Ranges" class="Clust (strict)"("Disabled"=w1260) -> ()  [unwired: 2 in, 2 out]
      }
      event "Current source settings.CS type": Value Change {
        # "Set CS type"
        n921 = event-data() -> ("NewVal"=w1263:T55)  [unwired: 1 in, 5 out]
        n922 = flat-sequence {
          tunnel: w1263 -> [w1290]
          frame #0 {
            w1275 = u8 2 ("Disabled")
            w1270 = u8 0 ("Disabled")
            w1285 = TRUE ("Visible")
            n923 = control-ref of="Current indicators"() -> (w1271:refnum<vi>)
            n924 = control-ref of="I0"() -> (w1282:refnum<vi>)
            n925 = control-ref of="I1"() -> (w1274:refnum<vi>)
            n926 = control-ref of="C_I0"() -> (w1281:refnum<vi>)
            n927 = control-ref of="C_I0 2"() -> (w1273:refnum<vi>)
            n928 = control-ref of="I2"() -> (w1269:refnum<vi>)
            n929 = control-ref of="I3"() -> (w1268:refnum<vi>)
            n930 = control-ref of="CS Mode"() -> (w1272:refnum<vi>)
            n931 = control-ref of="Map Channel 0 to 2"() -> (w1280:refnum<vi>)
            n932 = property class="TabCtl (strict)"(reference=w1271, "Disabled"=w1270) -> ()  [unwired: 1 in, 2 out]
            n933 = property class="Clust (strict)"(reference=w1282, "Disabled"=w1270) -> ()  [unwired: 1 in, 2 out]
            n934 = property class="Clust (strict)"(reference=w1274, "Disabled"=w1270) -> ()  [unwired: 1 in, 2 out]
            n935 = property class="Clust (strict)"(reference=w1269, "Disabled"=w1270) -> ()  [unwired: 1 in, 2 out]
            n936 = property class="Clust (strict)"(reference=w1268, "Disabled"=w1270) -> ()  [unwired: 1 in, 2 out]
            n937 = property class="Clust (strict)"(reference=w1281, "Disabled"=w1270) -> ()  [unwired: 1 in, 2 out]
            n938 = property class="Clust (strict)"(reference=w1273, "Disabled"=w1270) -> ()  [unwired: 1 in, 2 out]
            n939 = property class="Enum (strict)"(reference=w1280, "Disabled"=w1270) -> ()  [unwired: 1 in, 2 out]
            n940 = property class="Enum (strict)"(reference=w1272, "Disabled"=w1270) -> ()  [unwired: 1 in, 2 out]
            n941 = control-ref of="TCS_Port"() -> (w1284:refnum<vi>)
            n942 = property on="Tab Control 2" class="TabCtl (strict)"() -> ("Pages"=w1264:refnum<vi>[])  [unwired: 2 in, 2 out]
            n943 = Index Array(array=w1264, index=1) -> (element=w1265:refnum<vi>)
            n944 = control-ref of="Toggle Gated"() -> (w1276:refnum<vi>)
            n945 = control-ref of="Toggle Gated"() -> (w1277:refnum<vi>)
            n946 = control-ref of="Toggle Gated"() -> (w1278:refnum<vi>)
            n947 = control-ref of="Toggle Gated"() -> (w1279:refnum<vi>)
            n948 = control-ref of="QCS/PCS Device"() -> (w1287:refnum<vi>)
            n949 = control-ref of="I0 output to"() -> (w1286:refnum<vi>)
            n950 = property class="Page"(reference=w1265, "PageVis"=TRUE ("Page Visible")) -> ()  [unwired: 1 in, 2 out]
            n951 = property class="Bool (strict)"(reference=w1276, "Disabled"=w1275) -> ()  [unwired: 1 in, 2 out]
            n952 = property class="Bool (strict)"(reference=w1277, "Disabled"=w1275) -> ()  [unwired: 1 in, 2 out]
            n953 = property class="Bool (strict)"(reference=w1278, "Disabled"=w1275) -> ()  [unwired: 1 in, 2 out]
            n954 = property class="Bool (strict)"(reference=w1279, "Disabled"=w1275) -> ()  [unwired: 1 in, 2 out]
            n955 = property class="DigNum (strict)"(reference=w1287, "Visible"=w1285) -> ()  [unwired: 1 in, 2 out]
            n956 = property class="Enum (strict)"(reference=w1286, "Visible"=w1285) -> ()  [unwired: 1 in, 2 out]
            n957 = property class="VISAName"(reference=w1284, "Visible"=FALSE) -> ()  [unwired: 1 in, 2 out]
          }
          frame #1 {
            n958 = case shown="\"QCS v1\"" w1290 {
              tunnel: [refnum<class "TCS.lvclass"> refnum ("TCS.lvclass") refnum<class "QCS.lvclass"> refnum ("QCS.lvclass") w1310 w1324 refnum<class "PCS.lvclass"> refnum ("PCS.lvclass")] -> w1289
              tunnel: [w1291 w1309 u16 255 ("Value") u16 255 ("Value") w1329] -> w1288
              frame "TCS" {
                w1294 = u8 2 ("Disabled")
                w1307 = u8 0 ("Disabled")
                n959 = control-ref of="TCS_Port"() -> (w1297:refnum<vi>)
                n960 = control-ref of="Toggle Gated"() -> (w1306:refnum<vi>)
                n961 = control-ref of="Toggle Gated"() -> (w1305:refnum<vi>)
                n962 = control-ref of="Toggle Gated"() -> (w1304:refnum<vi>)
                n963 = control-ref of="Toggle Gated"() -> (w1303:refnum<vi>)
                n964 = control-ref of="QCS/PCS Device"() -> (w1299:refnum<vi>)
                n965 = control-ref of="I0"() -> (w1302:refnum<vi>)
                n966 = control-ref of="C_I0"() -> (w1295:refnum<vi>)
                n967 = control-ref of="Map Channel 0 to 2"() -> (w1296:refnum<vi>)
                n968 = property class="Bool (strict)"(reference=w1306, "Disabled"=w1307) -> ()  [unwired: 1 in, 2 out]
                n969 = property class="Bool (strict)"(reference=w1305, "Disabled"=w1307) -> ()  [unwired: 1 in, 2 out]
                n970 = property class="Bool (strict)"(reference=w1304, "Disabled"=w1307) -> ()  [unwired: 1 in, 2 out]
                n971 = property class="Bool (strict)"(reference=w1303, "Disabled"=w1307) -> ()  [unwired: 1 in, 2 out]
                n972 = property class="Clust (strict)"(reference=w1295, "Disabled"=w1294) -> ()  [unwired: 1 in, 2 out]
                n973 = property class="Clust (strict)"(reference=w1302, "Disabled"=u8 2) -> ()  [unwired: 1 in, 2 out]
                n974 = property class="DigNum (strict)"(reference=w1299, "Visible"=FALSE) -> ()  [unwired: 1 in, 2 out]
                n975 = property class="VISAName"(reference=w1297, "Visible"=TRUE) -> ()  [unwired: 1 in, 2 out]
                n976 = property class="Enum (strict)"(reference=w1296, "Disabled"=w1294) -> ()  [unwired: 1 in, 2 out]
                n977 = property on="TCS_Port" class="VISAName"() -> ("Value"=w1292:refnum<visa-resource-name>)  [unwired: 2 in, 2 out]
                n978 = call "VISA to RS232 Port Nr.vi"("VISA Resource Name"=w1292) -> ("Port Number"=w1291:u8)  [unwired: 1 in]
              }
              frame "QCS v1" {
                n979 = property on="QCS/PCS Device" class="DigNum (strict)"() -> ("Value"=w1309:u16)  [unwired: 2 in, 2 out]
              }
              frame "CS Emulation" {
                w1310 = refnum<class "CS Emulation.lvclass"> refnum  # CS Emulation.lvclass
                n980 = control-ref of="QCS/PCS Device"() -> (w1313:refnum<vi>)
                n981 = property class="DigNum (strict)"(reference=w1313, "Visible"=FALSE) -> ()  [unwired: 1 in, 2 out]
              }
              frame "Disabled", Default {
                w1314 = u8 2 ("Disabled")
                w1324 = refnum<class "CS Emulation.lvclass"> refnum  # CS Emulation.lvclass
                n982 = control-ref of="Current indicators"() -> (w1323:refnum<vi>)
                n983 = control-ref of="I0"() -> (w1318:refnum<vi>)
                n984 = control-ref of="I1"() -> (w1317:refnum<vi>)
                n985 = control-ref of="I2"() -> (w1316:refnum<vi>)
                n986 = control-ref of="I3"() -> (w1315:refnum<vi>)
                n987 = control-ref of="QCS/PCS Device"() -> (w1327:refnum<vi>)
                n988 = property class="DigNum (strict)"(reference=w1327, "Visible"=FALSE) -> ()  [unwired: 1 in, 2 out]
                n989 = property class="Clust (strict)"(reference=w1318, "Disabled"=w1314) -> ()  [unwired: 1 in, 2 out]
                n990 = property class="Clust (strict)"(reference=w1317, "Disabled"=w1314) -> ()  [unwired: 1 in, 2 out]
                n991 = property class="Clust (strict)"(reference=w1316, "Disabled"=w1314) -> ()  [unwired: 1 in, 2 out]
                n992 = property class="Clust (strict)"(reference=w1315, "Disabled"=w1314) -> ()  [unwired: 1 in, 2 out]
                n993 = property class="TabCtl (strict)"(reference=w1323, "Disabled"=w1314) -> ()  [unwired: 1 in, 2 out]
                n994 = property on="Tab Control 2" class="TabCtl (strict)"() -> ("Pages"=w1322:refnum<vi>[])  [unwired: 2 in, 2 out]
                n995 = Index Array(array=w1322, index=1) -> (element=w1321:refnum<vi>)
                n996 = property class="Page"(reference=w1321, "PageVis"=FALSE ("Page Visible")) -> ()  [unwired: 1 in, 2 out]
              }
              frame "PCS (n.a.)" {
                w1330 = u8 2 ("Disabled")
                n997 = control-ref of="I0"() -> (w1336:refnum<vi>)
                n998 = control-ref of="I1"() -> (w1335:refnum<vi>)
                n999 = control-ref of="C_I0"() -> (w1334:refnum<vi>)
                n1000 = control-ref of="C_I0 2"() -> (w1333:refnum<vi>)
                n1001 = control-ref of="CS Mode"() -> (w1332:refnum<vi>)
                n1002 = control-ref of="Map Channel 0 to 2"() -> (w1331:refnum<vi>)
                n1003 = property class="Clust (strict)"(reference=w1334, "Disabled"=w1330) -> ()  [unwired: 1 in, 2 out]
                n1004 = property class="Clust (strict)"(reference=w1333, "Disabled"=w1330) -> ()  [unwired: 1 in, 2 out]
                n1005 = property class="Clust (strict)"(reference=w1336, "Disabled"=w1330) -> ()  [unwired: 1 in, 2 out]
                n1006 = property class="Clust (strict)"(reference=w1335, "Disabled"=w1330) -> ()  [unwired: 1 in, 2 out]
                n1007 = property class="Enum (strict)"(reference=w1332, "Disabled"=w1330) -> ()  [unwired: 1 in, 2 out]
                n1008 = property class="Enum (strict)"(reference=w1331, "Disabled"=w1330) -> ()  [unwired: 1 in, 2 out]
                n1009 = property on="QCS/PCS Device" class="DigNum (strict)"() -> ("Value"=w1329:u16)  [unwired: 2 in, 2 out]
              }
            }
            "CS ref" <- w1289
            n1010 = property on="HW Address" class="DigNum (strict)"("Value"=w1288) -> ()  [unwired: 2 in, 2 out]
          }
        }
      }
      event "Current source settings.QCS/PCS Device": Value Change {
        # "Set CS port"
        n1011 = event-data() -> ("NewVal"=w1337:u16)  [unwired: 1 in, 5 out]
        n1012 = property on="CS type" class="Enum (strict)"() -> ("Value"=w1338:T55)  [unwired: 2 in, 2 out]
        n1013 = case shown="\"QCS v1\"" w1338 {
          tunnel: w1337 -> [_ w1341 _]
          frame Default {
          }
          frame "QCS v1" {
            n1014 = Variant To Data(type=u32 255 ("HW Address"), Variant=w1341) -> (data=w1339:u32)  [unwired: 1 in, 1 out]
            n1015 = property on="HW Address" class="DigNum (strict)"("Value"=w1339) -> ()  [unwired: 2 in, 2 out]
          }
          frame "CS Emulation" {
            n1016 = property on="HW Address" class="DigNum (strict)"("Value"=u32 255 ("HW Address")) -> ()  [unwired: 2 in, 2 out]
          }
        }
      }
      event "Current source settings.TCS_Port": Value Change {
        # "Set TCS port"
        n1017 = event-data() -> ("NewVal"=w1343:refnum<visa-resource-name>)  [unwired: 1 in, 5 out]
        n1018 = property on="CS type" class="Enum (strict)"() -> ("Value"=w1344:T55)  [unwired: 2 in, 2 out]
        n1019 = case shown="\"TCS\"" w1344 {
          tunnel: w1343 -> [w1347 _]
          frame "TCS" {
            n1020 = Type Cast(type=refnum<visa-resource-name> refnum ("Value"), x=w1347) -> (*(type *) &x=w1346:refnum<visa-resource-name>)
            n1021 = call "VISA to RS232 Port Nr.vi"("VISA Resource Name"=w1346) -> ("Port Number"=w1348:u8)  [unwired: 1 in]
            n1022 = property on="HW Address" class="DigNum (strict)"("Value"=w1348) -> ()  [unwired: 2 in, 2 out]
          }
          frame Default {
          }
        }
      }
      event "I3 as temp.I3 as temp 2": Value Change {
        # "Enable/disable the PID loop"
        n1023 = event-data() -> ("NewVal"=w1362:bool)  [unwired: 1 in, 5 out]
        n1024 = Unbundle By Name(w1350) -> ("Reset PID loop"=w1349:refnum<user-event>)
        n1025 = call "IsDisabled.vi"("Enabled?"=w1362) -> ("Numeric"=w1365:i16)
        n1026 = Generate User Event(user event=w1349, event data cluster="" ("event data")) -> ()  [unwired: 2 in, 2 out]
        n1027 = property on="PID setup" class="Clust (strict)"("Disabled"=w1365) -> ()  [unwired: 2 in, 2 out]
        n1028 = property on="FB on" class="Enum (strict)"() -> ("Value"=w1359:enum16{"Resistance", "Temperature"})  [unwired: 2 in, 2 out]
        n1029 = property on="FB on 2" class="Enum (strict)"() -> ("Value"=w1358:enum16{"0", "1", "2", "3"})  [unwired: 2 in, 2 out]
        n1030 = property on="I3 as temp 2" class="Bool (strict)"() -> ("Value"=w1352:bool)  [unwired: 2 in, 2 out]
        n1031 = Initialize Array(FALSE, 4 ("dimension size")) -> (w1354:bool[])
        n1032 = And(x=TRUE ("new element/subarray"), y=w1352) -> (x .and. y?=w1351:bool)
        n1033 = Index Array(array=string[] ["%#_g uA", "%#_g mK"], index=w1359) -> (element=w1361:string)
        n1034 = Replace Array Subset(array=w1354, new element=w1351, index=w1358) -> (w1357:bool[])
        n1035 = local write "T Channel"(w1357) -> ()
        n1036 = Select(t=w1361, s=w1362, f="%#_g uA") -> ()  [unwired: 1 out]
      }
      event "Load Data": Value Change {
        # "Load data from log files"
        n1037 = event-data() -> ()  [unwired: 1 in, 6 out]
        n1038 = property on="AVS_Path" class="Path"() -> ("Value"=w1368:path)  [unwired: 2 in, 2 out]
        n1039 = call "File Dialog4"("start path"=w1368) -> ("selected paths"=w1367:path[], "cancelled"=w1366:bool)  [unwired: 11 in, 2 out]
        n1040 = case shown="False" w1366 {
          tunnel: w1367 -> [w1382 _]
          frame False {
            n1041 = property on="AVS type" class="Enum (strict)"() -> ("Value"=w1372:T60)  [unwired: 2 in, 2 out]
            n1042 = case shown="Default" w1372 {
              tunnel: [2 ("index")] -> w1371
              tunnel: [10 ("length")] -> w1369
              tunnel: [12 ("index")] -> w1370
              frame Default {
              }
            }
            n1043 = for {
              tunnel: w1382 -> [w1406] mode=indexing
              shift-right: [w1404] -> w1379
              shift-left: string[][] [] ("all rows") -> [w1405]
              # "skip header"
              n1044 = call <vilib>:"Read From Spreadsheet File (string).vi"("file path (dialog if empty)"=w1406) -> ("all rows"=w1402:string[][])  [unwired: 6 in, 4 out]
              n1045 = Array Subset(array=w1402, index (row)=4 ("index")) -> (w1401:string[][])  [unwired: 3 in]
              n1046 = Insert Into Array(array=w1405, new element=w1401) -> (w1404:string[][])  [unwired: 2 in]
            }
            n1047 = Index Array(array=w1379, index (col)=1 ("disabled index (col)")) -> (element=w1376:string[])  [unwired: 1 in]
            n1048 = Array Subset(array=w1379, index (col)=w1371, length (col)=w1369) -> (w1378:string[][])  [unwired: 2 in]
            n1049 = Array Subset(array=w1379, index (col)=w1370, length (col)=w1369) -> (w1377:string[][])  [unwired: 2 in]
            n1050 = Transpose 2D Array(2D array=w1378) -> (transposed array=w1374:string[][])
            n1051 = Transpose 2D Array(2D array=w1377) -> (transposed array=w1373:string[][])
            n1052 = for {
              tunnel: w1374 -> [w1398] mode=indexing
              tunnel: w1373 -> [w1397] mode=indexing
              tunnel: w1376 -> [w1399]
              tunnel: [w1396] -> w1375 mode=indexing
              # "Sort data by date and remove duplicate points"
              n1053 = Fract/Exp String To Number(string=w1398) -> (number=w1393:dbl[])  [unwired: 3 in, 1 out]
              n1054 = Fract/Exp String To Number(string=w1399) -> (number=w1395:dbl[])  [unwired: 3 in, 1 out]
              n1055 = Fract/Exp String To Number(string=w1397) -> (number=w1394:dbl[])  [unwired: 3 in, 1 out]
              n1056 = call "Sort 1D Array (DBL)__ogtk.vi"("Array in"=w1395) -> ("Sorted Pointers"=w1400:i32[], "Sorted Array out"=w1388:dbl[])  [unwired: 9 in]
              n1057 = call "Reorder 1D Array2 (DBL)__ogtk.vi"("indices"=w1400, "array"=w1393) -> ("reordered array"=w1392:dbl[])  [unwired: 9 in]
              n1058 = call "Reorder 1D Array2 (DBL)__ogtk.vi"("indices"=w1400, "array"=w1394) -> ("reordered array"=w1390:dbl[])  [unwired: 9 in]
              n1059 = call "Remove Duplicates from 1D Array (DBL)__ogtk.vi"("Input Array"=w1392) -> ("Output Array"=w1391:dbl[], "indices of removed elements"=w1386:i32[])
              n1060 = call "Delete Elements from 1D Array (DBL)__ogtk.vi"("indices"=w1386, "array"=w1390) -> ("array w/ subset deleted"=w1389:dbl[])  [unwired: 8 in, 1 out]
              n1061 = call "Delete Elements from 1D Array (DBL)__ogtk.vi"("indices"=w1386, "array"=w1388) -> ("array w/ subset deleted"=w1387:dbl[])  [unwired: 8 in, 1 out]
              n1062 = Bundle("Output Array"=w1391, "array w/ subset deleted"=w1389, "array w/ subset deleted"=w1387) -> (w1396:T71)  [unwired: 1 in]
            }
            n1063 = local write "Data"(w1375) -> ()
          }
          frame True {
          }
        }
      }
      event "Save Data 2": Value Change {
        # "Load data from log files"
        n1064 = event-data() -> ()  [unwired: 1 in, 6 out]
        n1065 = property on="AVS_Path" class="Path"() -> ("Value"=w1411:path)  [unwired: 2 in, 2 out]
        n1066 = call "File Dialog"("start path"=w1411, "pattern (all files)"="*.dat", "pattern label"="Log files") -> ("selected path"=w1409:path, "cancelled"=w1410:bool)  [unwired: 9 in, 2 out]
        n1067 = case shown="False" w1410 {
          tunnel: w1409 -> [w1416 _]
          frame False {
            (unwired) 30 ("dimension size")
            n1068 = local read "Data"() -> (w1417:T28)
            n1069 = for {
              tunnel: w1417 -> [w1430] mode=indexing
              tunnel: [w1421] -> w1415 mode=indexing
              shift-right: [w1419] -> w1413
              shift-left: string[][] [] -> [w1420]
              n1070 = Unbundle By Name(w1430) -> ("Time"=w1427:dbl[], "R"=w1426:dbl[], "T"=w1422:dbl[])
              n1071 = property on="Data logging" class="Clust (strict)"() -> ("Value"=w1429:T37)  [unwired: 2 in, 2 out]
              n1072 = Unbundle By Name(w1429) -> ("Date/Time Format"=w1428:string)
              n1073 = Array Size(array=w1422) -> (size(s)=w1421:i32)
              n1074 = for {
                tunnel: w1428 -> [w1433]
                tunnel: [w1432] -> w1425 mode=indexing
                tunnel: w1427 -> [w1431] mode=indexing
                n1075 = Format Date/Time String(time format string (%c)=w1433, seconds (now)=w1431) -> (date/time string=w1432:string)  [unwired: 1 in]
              }
              n1076 = Number To Fractional String(number=w1426) -> (F-format string=w1424:string[])  [unwired: 3 in]
              n1077 = Number To Fractional String(number=w1422) -> (F-format string=w1423:string[])  [unwired: 3 in]
              n1078 = Build Array(w1425, w1424, w1423) -> (w1418:string[][])
              n1079 = Build Array (concatenate)(w1420, w1418) -> (w1419:string[][])
            }
            n1080 = Array Max & Min(array=w1415) -> ()  [unwired: 4 out]
            n1081 = call "Write To Spreadsheet File (string) w Error.vi"("transpose? (no:F)"=TRUE, "2D data"=w1413, "file path (dialog if empty)"=w1416) -> ()  [unwired: 7 in, 2 out]
          }
          frame True {
          }
        }
      }
      event "Plot-save-screen": Value Change {
        n1082 = event-data() -> ()  [unwired: 1 in, 6 out]
        n1083 = property on="AVS_Path" class="Path"() -> ("Value"=w1438:path)  [unwired: 2 in, 2 out]
        n1084 = call "File Dialog7"("start path"=w1438, "pattern (all files)"="*.dat", "pattern label"="Log files") -> ("selected path"=w1436:path, "cancelled"=w1437:bool)  [unwired: 9 in, 2 out]
        n1085 = case shown="False" w1437 {
          tunnel: w1436 -> [w1463 _]
          frame False {
            # "!!NOTE:This routine assumes that XY graph is \ncontrol #0 on tab page!!"
            n1086 = property on="Channel Controls" class="TabCtl (strict)"() -> ("Pages"=w1461:refnum<vi>[], "Value"=w1460:T8)  [unwired: 2 in, 2 out]
            n1087 = Index Array(array=w1461, index=w1460) -> (element=w1459:refnum<vi>)
            n1088 = property class="Page"(reference=w1459) -> ("ControlsOnPage"=w1456:refnum<vi>[])  [unwired: 1 in, 2 out]
            n1089 = control-ref of="R-Plot 0"() -> (w1454:refnum<vi>)
            n1090 = Index Array(array=w1456, index=0) -> (element=w1458:refnum<vi>)
            n1091 = Type Cast(type=w1454, x=w1458) -> (*(type *) &x=w1455:refnum<vi>)
            n1092 = property class="XYGraph (strict)"(reference=w1455) -> ("Value"=w1453:cluster{dbl[], dbl[]}, "XScale.Maximum"=w1452:dbl, "XScale.Minimum"=w1451:dbl)  [unwired: 1 in, 2 out]
            n1093 = Unbundle(w1453) -> (w1450:dbl[], w1449:dbl[])
            n1094 = call "MGI Threshold 1D Array Extended.vi"("Threshold Y"=w1452, "Y Value[]"=w1450) -> ("Extended Fractional Index"=w1440:dbl)  [unwired: 1 in]
            n1095 = call "MGI Threshold 1D Array Extended.vi"("Threshold Y"=w1451, "Y Value[]"=w1450) -> ("Extended Fractional Index"=w1439:dbl)  [unwired: 1 in]
            n1096 = Subtract(x=w1440, y=w1439) -> (x-y=w1462:dbl)
            n1097 = Array Subset(array=w1450, index=w1439, length=w1462) -> (w1444:dbl[])
            n1098 = Array Subset(array=w1449, index=w1439, length=w1462) -> (w1442:dbl[])
            n1099 = property on="Data logging" class="Clust (strict)"() -> ("Value"=w1446:T37)  [unwired: 2 in, 2 out]
            n1100 = Unbundle By Name(w1446) -> ("Date/Time Format"=w1445:string)
            n1101 = Number To Fractional String(number=w1442) -> (F-format string=w1441:string[])  [unwired: 3 in]
            n1102 = for {
              tunnel: w1445 -> [w1466]
              tunnel: [w1465] -> w1443 mode=indexing
              tunnel: w1444 -> [w1464] mode=indexing
              n1103 = Format Date/Time String(time format string (%c)=w1466, seconds (now)=w1464) -> (date/time string=w1465:string)  [unwired: 1 in]
            }
            n1104 = Build Array(w1443, w1441) -> (w1448:string[][])
            n1105 = call <vilib>:"Write To Spreadsheet File (string).vi"("transpose? (no:F)"=TRUE, "2D data"=w1448, "file path (dialog if empty)"=w1463) -> ()  [unwired: 5 in, 1 out]
          }
          frame True {
          }
        }
      }
      event "Plot-Save All": Value Change {
        n1106 = event-data() -> ()  [unwired: 1 in, 6 out]
        n1107 = property on="AVS_Path" class="Path"() -> ("Value"=w1471:path)  [unwired: 2 in, 2 out]
        n1108 = call "File Dialog8"("start path"=w1471, "pattern (all files)"="*.dat", "pattern label"="Log files") -> ("selected path"=w1469:path, "cancelled"=w1470:bool)  [unwired: 9 in, 2 out]
        n1109 = case shown="False" w1470 {
          tunnel: w1469 -> [w1489 _]
          frame False {
            # "!!NOTE:This routine assumes that XY graph is \ncontrol #0 on tab page!!"
            n1110 = property on="Channel Controls" class="TabCtl (strict)"() -> ("Pages"=w1488:refnum<vi>[], "Value"=w1487:T8)  [unwired: 2 in, 2 out]
            n1111 = Index Array(array=w1488, index=w1487) -> (element=w1486:refnum<vi>)
            n1112 = property class="Page"(reference=w1486) -> ("ControlsOnPage"=w1483:refnum<vi>[])  [unwired: 1 in, 2 out]
            n1113 = control-ref of="R-Plot 0"() -> (w1481:refnum<vi>)
            n1114 = Index Array(array=w1483, index=0) -> (element=w1485:refnum<vi>)
            n1115 = Type Cast(type=w1481, x=w1485) -> (*(type *) &x=w1482:refnum<vi>)
            n1116 = property class="XYGraph (strict)"(reference=w1482) -> ("Value"=w1480:cluster{dbl[], dbl[]})  [unwired: 1 in, 2 out]
            n1117 = Unbundle(w1480) -> (w1473:dbl[], w1472:dbl[])
            n1118 = property on="Data logging" class="Clust (strict)"() -> ("Value"=w1477:T37)  [unwired: 2 in, 2 out]
            n1119 = Unbundle By Name(w1477) -> ("Date/Time Format"=w1476:string)
            n1120 = Number To Fractional String(number=w1472) -> (F-format string=w1474:string[])  [unwired: 3 in]
            n1121 = for {
              tunnel: w1476 -> [w1492]
              tunnel: [w1491] -> w1475 mode=indexing
              tunnel: w1473 -> [w1490] mode=indexing
              n1122 = Format Date/Time String(time format string (%c)=w1492, seconds (now)=w1490) -> (date/time string=w1491:string)  [unwired: 1 in]
            }
            n1123 = Build Array(w1475, w1474) -> (w1479:string[][])
            n1124 = call <vilib>:"Write To Spreadsheet File (string).vi"("transpose? (no:F)"=TRUE, "2D data"=w1479, "file path (dialog if empty)"=w1489) -> ()  [unwired: 5 in, 1 out]
          }
          frame True {
          }
        }
      }
      event "Currents changed": Value Change {
        # "New values for currents were entered by user/automode-> write new data to CS"
        n1125 = event-data() -> ()  [unwired: 1 in, 6 out]
        n1126 = local read "CS ref"() -> (w1497:refnum<class "CS.lvclass">)
        n1127 = property on="CS status" class="Clust (strict)"() -> ("Value"=w1494:errorcluster)  [unwired: 2 in, 2 out]
        n1128 = call-dynamic "Read.vi"("CS in"=w1497, "error in (no error)"=w1494, "Optional"=TRUE ("Unused")) -> ("CS out"=w1496:refnum<class "CS.lvclass">, "error out"=w1493:errorcluster)  [unwired: 11 in, 4 out]
        n1129 = local write "CS ref"(w1496) -> ()
        n1130 = property on="CS status" class="Clust (strict)"("Value"=w1493) -> ()  [unwired: 2 in, 2 out]
      }
      event "I0 output to": Value Change {
        # "Switch QCS channel 0 to aux output"
        n1131 = event-data() -> ("OldVal"=w1504:T38, "NewVal"=w1499:T38)  [unwired: 1 in, 4 out]
        n1132 = To Long Integer(number=w1499) -> (32bit integer=→"Map Channel 0 to 2":i32)
        n1133 = local read "CS ref"() -> (w1502:refnum<class "CS.lvclass">)
        n1134 = property on="CS status" class="Clust (strict)"() -> ("Value"=w1503:errorcluster)  [unwired: 2 in, 2 out]
        n1135 = call-dynamic "Switch Output Channel.vi"("error in (no error)"=w1503, "New Channel"=w1499, "Old Channel"=w1504, "CS in"=w1502) -> ("error out"=w1500:errorcluster, "CS out"=w1501:refnum<class "CS.lvclass">)  [unwired: 6 in]
        n1136 = local write "CS ref"(w1501) -> ()
        n1137 = property on="CS status" class="Clust (strict)"("Value"=w1500) -> ()  [unwired: 2 in, 2 out]
      }
      event "T Sweep.Start": Value Change {
        # "Setup and Start Current/Temperature sweep for CS channel 3"
        n1138 = event-data() -> ("CtlRef"=w1505:refnum<vi>, "NewVal"=w1506:bool)  [unwired: 1 in, 4 out]
        n1139 = case shown="False" w1506 {
          tunnel: w1505 -> [w1507 w1510]
          frame False {
            n1140 = property class="Bool (strict)"(reference=w1507, "Caption.Text"="Start") -> ()  [unwired: 1 in, 2 out]
          }
          frame True {
            n1141 = property on="Start value" class="DigNum (strict)"() -> ("Value"=w1511:dbl)  [unwired: 2 in, 2 out]
            n1142 = property class="Bool (strict)"(reference=w1510, "Caption.Text"="Stop") -> ()  [unwired: 1 in, 2 out]
            n1143 = property on="Current" class="DigNum (strict)"("Val(Sgnl)"=w1511) -> ()  [unwired: 2 in, 2 out]
          }
        }
      }
      event "T Sweep.I_next": Value Change {
        # "Go to next step in Current/Temperature sweep for CS channel 3"
        n1144 = event-data() -> ()  [unwired: 1 in, 6 out]
        n1145 = property on="I_next" class="Bool (strict)"("Value"=FALSE) -> ()  [unwired: 2 in, 2 out]
        n1146 = call "Current Time(double).vi"() -> ("Current Time (double)"=w1512:dbl)  [unwired: 6 in, 1 out]
        n1147 = local write "Time Old"(w1512) -> ()
        n1148 = property on="Current" class="DigNum (strict)"() -> ("Value"=w1513:dbl)  [unwired: 2 in, 2 out]
        n1149 = property on="Step" class="DigNum (strict)"() -> ("Value"=w1518:dbl)  [unwired: 2 in, 2 out]
        n1150 = Add(x=w1513, y=w1518) -> (x+y=w1517:dbl)
        n1151 = property on="End value" class="DigNum (strict)"() -> ("Value"=w1516:dbl)  [unwired: 2 in, 2 out]
        n1152 = property on="Start value" class="DigNum (strict)"() -> ("Value"=w1515:dbl)  [unwired: 2 in, 2 out]
        n1153 = In Range and Coerce(upper limit=w1516, x=w1517, lower limit=w1515) -> (coerced(x)=w1514:dbl)  [unwired: 1 out]
        n1154 = property on="Current" class="DigNum (strict)"("Val(Sgnl)"=w1514) -> ()  [unwired: 2 in, 2 out]
      }
      event "T Sweep.I_prev": Value Change {
        # "Go to previous step in Current/Temperature sweep for CS channel 3"
        n1155 = event-data() -> ()  [unwired: 1 in, 6 out]
        n1156 = call "Current Time(double).vi"() -> ("Current Time (double)"=w1520:dbl)  [unwired: 6 in, 1 out]
        n1157 = property on="I_prev" class="Bool (strict)"("Value"=FALSE) -> ()  [unwired: 2 in, 2 out]
        n1158 = local write "Time Old"(w1520) -> ()
        n1159 = property on="Current" class="DigNum (strict)"() -> ("Value"=w1522:dbl)  [unwired: 2 in, 2 out]
        n1160 = property on="Step" class="DigNum (strict)"() -> ("Value"=w1527:dbl)  [unwired: 2 in, 2 out]
        n1161 = Subtract(x=w1522, y=w1527) -> (x-y=w1526:dbl)
        n1162 = property on="End value" class="DigNum (strict)"() -> ("Value"=w1525:dbl)  [unwired: 2 in, 2 out]
        n1163 = property on="Start value" class="DigNum (strict)"() -> ("Value"=w1524:dbl)  [unwired: 2 in, 2 out]
        n1164 = In Range and Coerce(upper limit=w1525, x=w1526, lower limit=w1524) -> (coerced(x)=w1523:dbl)  [unwired: 1 out]
        n1165 = property on="Current" class="DigNum (strict)"("Val(Sgnl)"=w1523) -> ()  [unwired: 2 in, 2 out]
      }
      event "Reset PID": Value Change {
        # "Reset the PID loop"
        n1166 = event-data() -> ()  [unwired: 1 in, 6 out]
        n1167 = Unbundle By Name(w1529) -> ("Reset PID loop"=w1528:refnum<user-event>)
        n1168 = Generate User Event(user event=w1528, event data cluster="" ("event data")) -> ()  [unwired: 2 in, 2 out]
      }
      event User Event {
        # "Reset the PID loop"
        n1169 = event-data() -> ()  [unwired: 1 in, 5 out]
        n1170 = local write "Error"(0.0 ("T_error")) -> ()
      }
      event "Minimize", "Minimize 2": Value Change {
        (unwired) 29 ("Splitter Position")
        (unwired) 534 ("Numeric 2")
        # "Shrink/restore the program window"
        # "726"
        # "222"
        # "1243"
        # "816"
        n1171 = event-data() -> ()  [unwired: 1 in, 6 out]
        n1172 = case shown="False" "Minimize" {
          tunnel: "Minimize 2" -> [_ w1559]
          frame True {
            (unwired) T52."Disabled" ("Value")
            n1173 = property on="CS type" class="Enum (strict)"() -> ("Value"=w1545:T55)  [unwired: 2 in, 2 out]
            n1174 = property on="AVS type" class="Enum (strict)"() -> ("Value"=w1540:T60)  [unwired: 2 in, 2 out]
            n1175 = Equal?(x=w1540, y=T52."Disabled" ("Value")) -> (x = y?=w1538:bool)
            n1176 = Equal?(x=w1545, y=T55."Disabled" ("Value")) -> (x = y?=w1544:bool)
            n1177 = property on="Data History" class="TabCtl (strict)"("Value"=enum32{"History", "Settings"}."History" ("Data History")) -> ()  [unwired: 2 in, 2 out]
            n1178 = Exclusive Or(1:w1538, 2:w1544) -> (0:w1537:bool)
            n1179 = property on="Mode Buttons" class="RadioBtnsControl (strict)"("Disabled"=u8 2, "Val(Sgnl)"=T54."No Selection" ("Value (Signaling)")) -> ()  [unwired: 2 in, 2 out]
            n1180 = property class="VI"() -> ("Front Panel.PanelBounds"=w1547:T72)  [unwired: 2 in, 2 out]
            n1181 = Select(t=i16 105 ("y"), s=w1537, f=i16 169 ("y")) -> (s? t:f=w1541:i16)
            n1182 = Unbundle By Name(w1547) -> ("Left"=w1553:i16, "Top"=w1550:i16)
            n1183 = property on="Splitter 3" class="Splitter"("Position"=29 ("Splitter Position")) -> (error out=w1539:errorcluster)  [unwired: 2 in, 1 out]
            n1184 = Add(x=i16 806 ("right"), y=w1553) -> (x+y=w1552:i16)
            n1185 = Add(x=w1550, y=w1541) -> (x+y=w1549:i16)
            n1186 = Bundle By Name(cluster=w1547, "Right"=w1552, "Bottom"=w1549) -> (w1554:T72)
            n1187 = case shown="True" w1538 {
              tunnel: w1539 -> [_ w1557]
              frame False {
              }
              frame True {
                n1188 = property on="Splitter 4" class="Splitter"(error in=w1557, "Position"=32 ("Splitter Position")) -> ()  [unwired: 1 in, 2 out]
              }
            }
            n1189 = property class="VI"("Front Panel.PanelBounds"=w1554) -> ()  [unwired: 2 in, 2 out]
          }
          frame False {
            n1190 = property class="VI"() -> ("Front Panel.PanelBounds"=w1566:T72)  [unwired: 2 in, 2 out]
            n1191 = property on="Channel Controls" class="TabCtl (strict)"() -> ("Value"=w1574:T8)  [unwired: 2 in, 2 out]
            n1192 = Unbundle By Name(w1566) -> ("Left"=w1572:i16, "Top"=w1570:i16)
            n1193 = property on="Channel Controls" class="TabCtl (strict)"("Val(Sgnl)"=w1574) -> ()  [unwired: 2 in, 2 out]
            n1194 = Select(t=i16 806 ("right"), s=w1559, f=i16 1206 ("right")) -> (s? t:f=w1563:i16)
            n1195 = Add(x=w1563, y=w1572) -> (x+y=w1571:i16)
            n1196 = Add(x=w1570, y=i16 702) -> (x+y=w1568:i16)
            n1197 = Bundle By Name(cluster=w1566, "Right"=w1571, "Bottom"=w1568) -> (w1573:T72)
            n1198 = property on="Mode Buttons" class="RadioBtnsControl (strict)"("Disabled"=u8 0) -> ()  [unwired: 2 in, 2 out]
            n1199 = property class="VI"("Front Panel.PanelBounds"=w1573) -> (error out=w1560:errorcluster)  [unwired: 2 in, 1 out]
            n1200 = property on="Splitter 3" class="Splitter"(error in=w1560, "Position"=559 ("Splitter Position")) -> (error out=w1564:errorcluster)  [unwired: 1 in, 1 out]
            n1201 = property on="Splitter 4" class="Splitter"(error in=w1564, "Position"=635 ("Splitter Position")) -> ()  [unwired: 1 in, 2 out]
          }
        }
        n1202 = property on="Splitter 2" class="Splitter"("Position"=805 ("Splitter Position")) -> ()  [unwired: 2 in, 2 out]
      }
      event "Copy to Clipboard": Value Change {
        # "Copy current values to the clipboard"
        n1203 = event-data() -> ()  [unwired: 1 in, 6 out]
        n1204 = property on="Data array" class="Arr (strict)"() -> ("Value"=w1579:dbl[])  [unwired: 2 in, 2 out]
        n1205 = property on="T_array" class="Arr (strict)"() -> ("Value"=w1578:dbl[])  [unwired: 2 in, 2 out]
        n1206 = Build Array(w1579, w1578) -> (w1577:dbl[][])
        n1207 = Transpose 2D Array(2D array=w1577) -> (transposed array=w1576:dbl[][])
        n1208 = Array To Spreadsheet String(delimiter (Tab)="\t", array=w1576, 3:"%.4g" ("format string")) -> (spreadsheet string=w1582:string)
        n1209 = invoke class="App" method="Clipboard.Write"("Param 0"=w1582) -> ()  [unwired: 3 in, 4 out]
      }
      event "Show PID graph?": Value Change {
        # "Display plots with the PID parameters vs time for debugging"
        n1210 = event-data() -> ("NewVal"=w1583:bool)  [unwired: 1 in, 5 out]
        n1211 = property on="Channel Controls" class="TabCtl (strict)"() -> ("Pages"=w1586:refnum<vi>[])  [unwired: 2 in, 2 out]
        n1212 = Reverse 1D Array(array=w1586) -> (reversed array=w1585:refnum<vi>[])
        n1213 = Index Array(array=w1585) -> (element=w1584:refnum<vi>)  [unwired: 1 in]
        n1214 = property class="Page"(reference=w1584, "PageVis"=w1583) -> ()  [unwired: 1 in, 2 out]
      }
      event "I0.uA", "I1.uA", "I2.uA", "I3.uA": Mouse Up {
        # "Show curent edit filed on double clicking the current indicator. Set the field to the actual current value."
        n1215 = event-data() -> ("Mods.Double Click"=w1588:bool, "CtlRef"=w1587:refnum<vi>)  [unwired: 1 in, 5 out]
        n1216 = case shown="True" w1588 {
          tunnel: w1587 -> [_ w1599]
          frame False {
          }
          frame True {
            w1595 = TRUE ("Visible")
            n1217 = property class="Str"(reference=w1599) -> ("Owner"=w1598:refnum<vi>)  [unwired: 1 in, 2 out]
            n1218 = control-ref of="uA 0"() -> (w1605:refnum<vi>)
            n1219 = control-ref of="uA 1"() -> (w1608:refnum<vi>)
            n1220 = control-ref of="uA 2"() -> (w1607:refnum<vi>)
            n1221 = control-ref of="uA 3"() -> (w1606:refnum<vi>)
            n1222 = control-ref of="I0"() -> (w1596:refnum<vi>)
            n1223 = control-ref of="I1"() -> (w1602:refnum<vi>)
            n1224 = control-ref of="I2"() -> (w1601:refnum<vi>)
            n1225 = control-ref of="I3"() -> (w1594:refnum<vi>)
            n1226 = property on="I" class="Arr (strict)"() -> ("Value"=w1593:dbl[])  [unwired: 2 in, 2 out]
            n1227 = Type Cast(type=w1594, x=w1598) -> (*(type *) &x=w1597:refnum<vi>)
            n1228 = Build Array(w1605, w1608, w1607, w1606) -> (w1604:refnum<vi>[])
            n1229 = Build Array(w1596, w1602, w1601, w1594) -> (w1600:refnum<vi>[])
            n1230 = Search 1D Array(1D array=w1600, element=w1597) -> (index of element=w1592:i32)  [unwired: 1 in]
            n1231 = Index Array(array=w1593, index=w1592) -> (element=w1591:dbl)
            n1232 = Index Array(array=w1604, index=w1592) -> (element=w1603:refnum<vi>)
            n1233 = Multiply(x=1000.0, y=w1591) -> (x*y=w1590:dbl)
            n1234 = property on="Property Node" class="DigNum (strict)"(reference=w1603, "Value"=w1590, "Visible"=w1595, "Key Focus"=w1595) -> ()  [unwired: 1 in, 2 out]
          }
        }
      }
      event "I0.current flows", "I1.current flows", "I2.current flows", "I3.current flows": Mouse Up {
        # "Toggle the current channel by double clickin on the \"On\" led in the current indicator."
        n1235 = event-data() -> ("CtlRef"=w1609:refnum<vi>, "Mods.Double Click"=w1610:bool)  [unwired: 1 in, 5 out]
        n1236 = case shown="True" w1610 {
          tunnel: w1609 -> [_ w1619]
          frame False {
          }
          frame True {
            n1237 = control-ref of="current flows"() -> (w1624:refnum<vi>)
            n1238 = control-ref of="current flows"() -> (w1623:refnum<vi>)
            n1239 = control-ref of="current flows"() -> (w1622:refnum<vi>)
            n1240 = control-ref of="current flows"() -> (w1621:refnum<vi>)
            n1241 = control-ref of="Toggle ON/OFF"() -> (w1618:refnum<vi>)
            n1242 = control-ref of="Toggle ON/OFF"() -> (w1616:refnum<vi>)
            n1243 = control-ref of="Toggle ON/OFF"() -> (w1615:refnum<vi>)
            n1244 = control-ref of="Toggle ON/OFF"() -> (w1617:refnum<vi>)
            n1245 = Build Array(w1624, w1623, w1622, w1621) -> (w1620:refnum<vi>[])
            n1246 = Build Array(w1618, w1616, w1615, w1617) -> (w1614:refnum<vi>[])
            n1247 = Search 1D Array(1D array=w1620, element=w1619) -> (index of element=w1613:i32)  [unwired: 1 in]
            n1248 = Index Array(array=w1614, index=w1613) -> (element=w1612:refnum<vi>)
            n1249 = property class="Bool (strict)"(reference=w1612, "Val(Sgnl)"=TRUE ("Value (Signaling)")) -> ()  [unwired: 1 in, 2 out]
          }
        }
      }
      event "uA 0", "uA 1", "uA 2", "uA 3": Value Change {
        w1626 = refnum<vi> refnum  # Numeric
        w1630 = refnum<vi> refnum  # Enum
        # "User has entered the current by double clicking on the current indicators at the bottom. \nSet range to \"Auto\" and interpret the entered value as [uA]"
        # "!!NOTE:This routine assumes that Current and Range are controls #2 & #3 in current control cluster"
        n1250 = event-data() -> ("CtlRef"=w1638:refnum<vi>, "NewVal"=w1625:u32)  [unwired: 1 in, 4 out]
        n1251 = control-ref of="C_I0"() -> (w1647:refnum<vi>)
        n1252 = control-ref of="C_I0 2"() -> (w1645:refnum<vi>)
        n1253 = control-ref of="C_I0 3"() -> (w1646:refnum<vi>)
        n1254 = control-ref of="C_I0 4"() -> (w1648:refnum<vi>)
        n1255 = control-ref of="uA 0"() -> (w1640:refnum<vi>)
        n1256 = control-ref of="uA 1"() -> (w1643:refnum<vi>)
        n1257 = control-ref of="uA 2"() -> (w1642:refnum<vi>)
        n1258 = control-ref of="uA 3"() -> (w1641:refnum<vi>)
        n1259 = Build Array(w1647, w1645, w1646, w1648) -> (w1644:refnum<vi>[])
        n1260 = Build Array(w1640, w1643, w1642, w1641) -> (w1639:refnum<vi>[])
        n1261 = Search 1D Array(1D array=w1639, element=w1638) -> (index of element=w1637:i32)  [unwired: 1 in]
        n1262 = Index Array(array=w1644, index=w1637) -> (element=w1636:refnum<vi>)
        n1263 = property class="Clust (strict)"(reference=w1636) -> ("Controls[]"=w1635:refnum<vi>[])  [unwired: 1 in, 2 out]
        n1264 = Index Array(array=w1635, index #1=3 ("index"), index #2=2 ("index")) -> (element #1=w1632:refnum<vi>, element #2=w1628:refnum<vi>)
        n1265 = Type Cast(type=w1626, x=w1628) -> (*(type *) &x=w1627:refnum<vi>)
        n1266 = Type Cast(type=w1630, x=w1632) -> (*(type *) &x=w1631:refnum<vi>)
        n1267 = property on="Property Node" class="Num"(reference=w1627, "Value"=w1625) -> ()  [unwired: 1 in, 2 out]
        n1268 = property on="Property Node" class="Enum"(reference=w1631, "Value"=T56."Auto") -> ()  [unwired: 1 in, 2 out]
      }
      event "Ranges": Value Change {
        # "If user has changed the exitation, update the AVS bridge settings."
        n1269 = event-data() -> ("NewVal"=w1650:T29)  [unwired: 1 in, 5 out]
        n1270 = property on="Exc&Ranges" class="Clust (strict)"() -> ("Value"=w1649:T15)  [unwired: 2 in, 2 out]
        n1271 = call "Combine Excitation&Range.vi"("Ranges"=w1650, "Exc&Ranges In"=w1649) -> ("Exc&Ranges Out"=w1651:T73)
        n1272 = property on="Exc&Ranges" class="Clust (strict)"("Value"=w1651) -> ()  [unwired: 2 in, 2 out]
      }
      event Panel Close? {
        # "Ask for confirmation is user is trying to close the program"
        n1273 = event-data() -> ()  [unwired: 1 in, 4 out]
        n1274 = Two Button Dialog(message="Are you sure you want to quit the program?") -> (T button?=w1653:bool)  [unwired: 2 in]
        n1275 = Not(x=w1653) -> (.not. x?=w1654:bool)
        n1276 = event-data("Discard?"=w1654) -> ()  [unwired: 1 in, 1 out]
      }
      event "Save config": Mouse Up {
        (unwired) T58."HKEY_CURRENT_USER" ("root key (HKEY_LOCAL_MACHINE) 2")
        # "Save parameters to the configuration file"
        n1277 = event-data() -> ()  [unwired: 1 in, 8 out]
        n1278 = control-ref of="CS Names"() -> (w1665:refnum<vi>)
        n1279 = control-ref of="AVS names"() -> (w1664:refnum<vi>)
        n1280 = control-ref of="CurCalibrations"() -> (w1658:refnum<vi>)
        n1281 = control-ref of="I3 as temp"() -> (w1656:refnum<vi>)
        n1282 = control-ref of="Automode Settings 2"() -> (w1655:refnum<vi>)
        n1283 = control-ref of="Active"() -> (w1657:refnum<vi>)
        n1284 = control-ref of="Bridge settings"() -> (w1671:refnum<vi>)
        n1285 = control-ref of="Runtime Settings"() -> (w1672:refnum<vi>)
        n1286 = control-ref of="Current source settings"() -> (w1670:refnum<vi>)
        n1287 = control-ref of="Thermometer"() -> (w1673:refnum<vi>)
        n1288 = control-ref of="PID setup"() -> (w1674:refnum<vi>)
        n1289 = control-ref of="Data logging"() -> (w1669:refnum<vi>)
        n1290 = call "Current VIs Parent Directory__ogtk.vi"() -> ("Parent Directory (+ Relative)"=w1661:path)  [unwired: 5 in]
        n1291 = call "File Dialog3"("start path"=w1661, "pattern (all files)"="*.ini") -> ("selected path"=w1659:path)  [unwired: 10 in, 3 out]
        n1292 = Build Array(w1657, w1671, w1672, w1670, w1669, w1673, w1674, w1665, w1664, w1658, w1656, w1655) -> (w1667:refnum<vi>[])
        n1293 = call "Save Load Settings to File by Ref with path.vi"("Array of Cluster References"=w1667, "subkey"="SOFTWARE\\Leiden Cryogenics\\TC" ("subkey 2"), "Action"=enum8{"Load", "Save"}."Save", "error in (no error)"=w1663, "configuration file path"=w1659) -> ("error out"=w1662:errorcluster)  [unwired: 4 in]
      }
      event "Load config": Mouse Up {
        # "Load parameters from the configuration file"
        n1294 = event-data() -> ()  [unwired: 1 in, 8 out]
        n1295 = Unbundle By Name(w1676) -> ("UpdateCalibrations"=w1675:refnum<user-event>)
        n1296 = flat-sequence {
          tunnel: [w1701] -> w1686
          tunnel: w1682 -> [w1696]
          tunnel: [w1687] -> w1677
          tunnel: w1686 -> [w1717]
          tunnel: [w1717] -> w1685
          tunnel: [w1715] -> w1678
          tunnel: w1677 -> [w1715]
          tunnel: [w1722] -> w1684
          tunnel: w1685 -> [w1721]
          tunnel: [w1719] -> w1679
          tunnel: w1678 -> [w1719]
          tunnel: w1684 -> [w1728]
          tunnel: [w1728] -> w1683
          tunnel: [w1726] -> w1680
          tunnel: w1679 -> [w1726]
          tunnel: w1683 -> [w1732]
          tunnel: [w1731] -> w1681
          tunnel: w1680 -> [w1730]
          tunnel: w1675 -> [w1729]
          frame #0 {
            (unwired) T58."HKEY_CURRENT_USER" ("root key (HKEY_LOCAL_MACHINE) 2")
            n1297 = call "Current VIs Parent Directory__ogtk.vi"() -> ("Parent Directory (+ Relative)"=w1693:path)  [unwired: 5 in]
            n1298 = control-ref of="Active"() -> (w1690:refnum<vi>)
            n1299 = control-ref of="Bridge settings"() -> (w1702:refnum<vi>)
            n1300 = control-ref of="Runtime Settings"() -> (w1698:refnum<vi>)
            n1301 = control-ref of="Current source settings"() -> (w1699:refnum<vi>)
            n1302 = control-ref of="Data logging"() -> (w1700:refnum<vi>)
            n1303 = control-ref of="PID setup"() -> (w1697:refnum<vi>)
            n1304 = control-ref of="CS Names"() -> (w1695:refnum<vi>)
            n1305 = control-ref of="AVS names"() -> (w1694:refnum<vi>)
            n1306 = control-ref of="CurCalibrations"() -> (w1691:refnum<vi>)
            n1307 = control-ref of="I3 as temp"() -> (w1689:refnum<vi>)
            n1308 = control-ref of="Automode Settings 2"() -> (w1688:refnum<vi>)
            n1309 = call "File Dialog2"("start path"=w1693, "pattern (all files)"="*.ini") -> ("selected path"=w1687:path)  [unwired: 10 in, 3 out]
            n1310 = Build Array(w1690, w1702, w1698, w1699, w1700, w1697, w1695, w1694, w1691, w1689, w1688) -> (w1704:refnum<vi>[])
            n1311 = call "Save Load Settings to File by Ref with path.vi"("Array of Cluster References"=w1704, "subkey"="SOFTWARE\\Leiden Cryogenics\\TC" ("subkey 2"), "Action"=enum8{"Load", "Save"}."Load", "error in (no error)"=w1696, "configuration file path"=w1687) -> ("error out"=w1706:errorcluster)  [unwired: 4 in]
            n1312 = disable-structure shown="Disabled" {
              disable-tunnel: w1706 -> [w1709 w1714]
              disable-tunnel: [w1707 w1714] -> w1701
              frame Disabled {
                n1313 = property on="AVS type" class="Enum (strict)"(error in=w1709) -> (error out=w1710:errorcluster, "Value"=w1712:T60)  [unwired: 1 in, 1 out]
                n1314 = Equal To 0?(x=w1712) -> (x = 0?=w1713:bool)
                n1315 = property on="Address" class="VISAName"(error in=w1710, "Visible"=w1713) -> (error out=w1711:errorcluster)  [unwired: 1 in, 1 out]
                n1316 = Not(x=w1713) -> (.not. x?=w1708:bool)
                n1317 = property on="AVS_SPort" class="VISAName"(error in=w1711, "Visible"=w1708) -> (error out=w1707:errorcluster)  [unwired: 1 in, 1 out]
              }
              frame Enabled {
              }
            }
          }
          frame #1 {
            n1318 = Wait (ms)(milliseconds to wait=250) -> ()  [unwired: 1 out]
          }
          frame #2 {
            n1319 = control-ref of="Thermometer"() -> (w1720:refnum<vi>)
            n1320 = control-ref of="CurCalibrations"() -> (w1718:refnum<vi>)
            n1321 = control-ref of="AVS_CalFolder"() -> (w1724:refnum<vi>)
            n1322 = control-ref of="Select sensor 1"() -> (w1725:refnum<vi>)
            n1323 = control-ref of="Select sensor 1"() -> (w1723:refnum<vi>)
            n1324 = call "ReloadCalibrations.vi"("error in (no error)"=w1721, "Quick convert sensors"=w1723, "CurCalibrations"=w1718, "Calibration files path"=w1724, "Channel1 sensors"=w1725, "Channels list"=w1720) -> ("error out"=w1722:errorcluster)  [unwired: 1 in]
          }
          frame #3 {
            n1325 = Wait (ms)(milliseconds to wait=250) -> ()  [unwired: 1 out]
          }
          frame #4 {
            n1326 = disable-structure shown="Disabled" {
              disable-tunnel: w1732 -> [w1735 w1741]
              disable-tunnel: [w1734 w1743] -> w1731
              disable-tunnel: w1730 -> [w1733 _]
              disable-tunnel: w1729 -> [_ w1740]
              frame Enabled {
                (unwired) T58."HKEY_CURRENT_USER" ("root key (HKEY_LOCAL_MACHINE) 2")
                n1327 = control-ref of="Thermometer"() -> (w1738:refnum<vi>)
                n1328 = Build Array(w1738) -> (w1737:refnum<vi>[])
                n1329 = call "Save Load Settings to File by Ref with path.vi"("Array of Cluster References"=w1737, "subkey"="SOFTWARE\\Leiden Cryogenics\\TC" ("subkey 2"), "Action"=enum8{"Load", "Save"}."Load", "error in (no error)"=w1735, "configuration file path"=w1733) -> ("error out"=w1734:errorcluster)  [unwired: 4 in]
              }
              frame Disabled {
                n1330 = Generate User Event(user event=w1740, event data cluster="" ("event data"), error in=w1741) -> (error out=w1743:errorcluster)  [unwired: 1 in, 1 out]
              }
            }
          }
        }
      }
      event "zBridge settings": Value Change {
        # "Show parameters menu. (only for zBridge)"
        n1331 = event-data() -> ()  [unwired: 1 in, 6 out]
        n1332 = disable-structure shown="Disabled" {
          frame Enabled {
            w1748 = 0 ("Page")
            n1333 = local read "zConfig"() -> (w1744:path)
            n1334 = local read "zDll"() -> (w1745:path)
            n1335 = call "SetParFilePath.vi"("path"=w1744, "zDll"=w1745) -> ("error out"=w1746:errorcluster, "zDll out"=w1747:path)  [unwired: 8 in]
            n1336 = call "ParamMenu.vi"("error in (no error)"=w1746, "Subpage"=w1748, "Page"=w1748, "path in"=w1747) -> ()  [unwired: 6 in, 2 out]
          }
          frame Disabled {
            n1337 = local read "zConfig"() -> (w1751:path)
            n1338 = local read "zDll"() -> (w1749:path)
            n1339 = call "SetParFilePath.vi"("path"=w1751, "zDll"=w1749) -> ("zDll out"=w1750:path)  [unwired: 8 in, 1 out]
            n1340 = call "zBridgeSettings_1page.vi"("zDll"=w1750) -> ()  [unwired: 10 in, 1 out]
          }
        }
      }
      event "Edit Calibrations": Value Change {
        # "Show calibration files editor. Works with .cal and .cal2 files only"
        n1341 = event-data() -> ("NewVal"=w1762:T11)  [unwired: 1 in, 5 out]
        n1342 = Unbundle By Name(w1753) -> ("UpdateCalibrations"=w1752:refnum<user-event>)
        n1343 = Cluster To Array(cluster=w1762) -> (array=w1761:bool[])
        n1344 = local read "CurCalibrations"() -> (w1756:T33)
        n1345 = Search 1D Array(1D array=w1761, element=TRUE) -> (index of element=w1759:i32)  [unwired: 1 in]
        n1346 = Cluster To Array(cluster=w1756) -> (array=w1755:string[])
        n1347 = Index Array(array=w1755, index=w1759) -> (element=w1758:string)
        n1348 = property on="AVS_CalFolder" class="Path"() -> ("Value"=w1757:path)  [unwired: 2 in, 2 out]
        n1349 = call "Edit Calibration Coefficients.vi"("Calibration Name"=w1758, "Calibration folder"=w1757) -> ("Cancelled?"=w1754:bool)  [unwired: 1 out]
        n1350 = case shown="False" w1754 {
          tunnel: w1752 -> [w1763 _]
          frame False {
            n1351 = Generate User Event(user event=w1763, event data cluster="" ("event data")) -> ()  [unwired: 2 in, 2 out]
          }
          frame True {
          }
        }
      }
      event "Edit calibration": Value Change {
        # "Show calibration files editor for quick convert R->T. Works with .cal and .cal2 files only"
        n1352 = event-data() -> ()  [unwired: 1 in, 6 out]
        n1353 = Unbundle By Name(w1766) -> ("UpdateCalibrations"=w1765:refnum<user-event>)
        n1354 = property on="Select sensor 1" class="Ring (strict)"() -> ("Strings []"=w1769:string[], "Value"=w1770:u16)  [unwired: 2 in, 2 out]
        n1355 = Index Array(array=w1769, index=w1770) -> (element=w1768:string)
        n1356 = property on="AVS_CalFolder" class="Path"() -> ("Value"=w1771:path)  [unwired: 2 in, 2 out]
        n1357 = call "Edit Calibration Coefficients.vi"("Calibration Name"=w1768, "Calibration folder"=w1771) -> ("Cancelled?"=w1767:bool)  [unwired: 1 out]
        n1358 = case shown="False" w1767 {
          tunnel: w1765 -> [w1772 _]
          frame False {
            n1359 = Generate User Event(user event=w1772, event data cluster="" ("event data")) -> ()  [unwired: 2 in, 2 out]
          }
          frame True {
          }
        }
      }
      event "zBridge params.AVS Name 0", "zBridge params.AVS Name 1", "zBridge params.AVS Name 2", "zBridge params.AVS Name 3", "zBridge params.AVS Name 4", "zBridge params.AVS Name 5", "zBridge params.AVS Name 6", "zBridge params.AVS Name 7", "zBridge params.AVS Name 8", "zBridge params.AVS Name 9": Mouse Down {
        # "Show parameters menu for the channel by double clicking on \"Channel parameters\". (only for zBridge)"
        n1360 = event-data() -> ("CtlRef"=w1776:refnum<vi>, "Mods.Double Click"=w1775:bool, "PlatMods.Alt"=w1774:bool)  [unwired: 1 in, 5 out]
        n1361 = case shown="True" w1775 {
          tunnel: w1776 -> [w1779 w1784]
          tunnel: w1774 -> [_ w1783]
          frame True {
            n1362 = control-ref of="zBridge params"() -> (w1781:refnum<vi>)
            n1363 = property class="Clust (strict)"(reference=w1781) -> ("Controls[]"=w1780:refnum<vi>[])  [unwired: 1 in, 2 out]
            n1364 = Search 1D Array(1D array=w1780, element=w1779) -> (index of element=w1777:i32)  [unwired: 1 in]
            n1365 = local read "zDll"() -> (w1782:path)
            n1366 = call "ParamMenu.vi"("Subpage"=w1777, "Page"=0, "path in"=w1782) -> ()  [unwired: 7 in, 2 out]
          }
          frame False {
            n1367 = case shown="True" w1783 {
              tunnel: w1784 -> [_ w1785]
              frame False {
              }
              frame True {
                n1368 = disable-structure shown="Enabled" {
                  disable-tunnel: w1785 -> [w1788 w1792]
                  frame Disabled {
                    # "Show information window.\nTends to crash the acquisition!"
                    n1369 = control-ref of="zBridge params"() -> (w1790:refnum<vi>)
                    n1370 = property class="Clust (strict)"(reference=w1790) -> ("Controls[]"=w1789:refnum<vi>[])  [unwired: 1 in, 2 out]
                    n1371 = local read "zDll"() -> (w1787:path)
                    n1372 = Search 1D Array(1D array=w1789, element=w1788) -> (index of element=w1786:i32)  [unwired: 1 in]
                    n1373 = call "Show Info Window.vi"("Data set number"=w1786, "zDll"=w1787) -> ()  [unwired: 8 in, 2 out]
                  }
                  frame Enabled {
                    # "Show information window."
                    n1374 = control-ref of="zBridge params"() -> (w1794:refnum<vi>)
                    n1375 = property class="Clust (strict)"(reference=w1794) -> ("Controls[]"=w1793:refnum<vi>[])  [unwired: 1 in, 2 out]
                    n1376 = Search 1D Array(1D array=w1793, element=w1792) -> (index of element=w1791:i32)  [unwired: 1 in]
                    n1377 = call "Scan Parameters Window.vi"("index"=w1791) -> ()  [unwired: 11 in]
                  }
                }
              }
            }
          }
        }
      }
      event "Active.active Channel 0", "Active.active Channel 1", "Active.active Channel 2", "Active.active Channel 3", "Active.active Channel 4", "Active.active Channel 5", "Active.active Channel 6", "Active.active Channel 7", "Active.active Channel 8", "Active.active Channel 9": Mouse Down {
        # "Switch channels On/Off by double clicking on \"Active\" LED. (only for zBridge and AVS47B)"
        n1378 = event-data() -> ("CtlRef"=w1797:refnum<vi>, "Mods.Double Click"=w1795:bool)  [unwired: 1 in, 6 out]
        n1379 = property on="AVS type" class="Enum (strict)"() -> ("Value"=w1796:T60)  [unwired: 2 in, 2 out]
        n1380 = case shown="True" w1795 {
          tunnel: w1797 -> [_ w1799]
          tunnel: w1796 -> [_ w1803]
          frame False {
          }
          frame True {
            n1381 = control-ref of="Active"() -> (w1802:refnum<vi>)
            n1382 = property class="Clust (strict)"(reference=w1802) -> ("Controls[]"=w1800:refnum<vi>[])  [unwired: 1 in, 2 out]
            n1383 = property class="Bool (strict)"(reference=w1799) -> ("Value"=w1798:bool)  [unwired: 1 in, 2 out]
            n1384 = Search 1D Array(1D array=w1800, element=w1799) -> (index of element=w1801:i32)  [unwired: 1 in]
            n1385 = case shown="Default" w1803 {
              tunnel: w1801 -> [_ w1808 w1809]
              tunnel: w1800 -> [_ w1807 _]
              tunnel: w1798 -> [_ w1804 _]
              frame Default {
              }
              frame "AVS47B (RS232 interface)" {
                n1386 = Index Array(array=w1807, index=w1808) -> (element=w1806:refnum<vi>)
                n1387 = Not(x=w1804) -> (.not. x?=w1805:bool)
                n1388 = property class="Ctl"(reference=w1806, "Value"=w1805) -> ()  [unwired: 1 in, 2 out]
              }
              frame "Impedance Bridge" {
                w1811 = Byte_Params."Active" ("Enum")
                # "Invert Active flag"
                n1389 = local read "zDll"() -> (w1814:path)
                n1390 = call "GetByteParam.vi"("ParNo"=w1811, "SetNo"=w1809, "zDll"=w1814) -> ("return type"=w1813:u8)  [unwired: 6 in, 2 out]
                n1391 = Decrement(x=w1813) -> (x-1=w1812:i8)
                n1392 = Absolute Value(x=w1812) -> (abs(x)=w1810:i8)
                n1393 = call "SetByteParam.vi"("SetNo"=w1809, "ParNo"=w1811, "Data"=w1810, "zDll"=w1814) -> ()  [unwired: 6 in, 2 out]
              }
            }
          }
        }
      }
      event "Small R.R1 2", "Small R.R1 2", "Small R.R1 2", "Small R.R1 2", "Small R.R1 2", "Small R.R1 2", "Small R.R1 2", "Small R.R1 2", "Small R.R1 2", "Small R.R1 2", "Small T.R1", "Small T.R1", "Small T.R1", "Small T.R1", "Small T.R1", "Small T.R1", "Small T.R1", "Small T.R1", "Small T.R1", "Small T.R1": Mouse Down {
        n1394 = event-data() -> ()  [unwired: 1 in, 8 out]
      }
      event Value Change {
        n1395 = event-data() -> ("NewVal"=w1819:enum16{"0", "1", "2", "3"})  [unwired: 1 in, 5 out]
        n1396 = Unbundle By Name(w1817) -> ("Reset PID loop"=w1816:refnum<user-event>)
        n1397 = Generate User Event(user event=w1816, event data cluster="" ("event data")) -> ()  [unwired: 2 in, 2 out]
        n1398 = property on="I3 as temp 2" class="Bool (strict)"() -> ("Value"=w1821:bool)  [unwired: 2 in, 2 out]
        n1399 = Initialize Array(FALSE, 4 ("dimension size")) -> (w1823:bool[])
        n1400 = And(x=TRUE ("new element/subarray"), y=w1821) -> (x .and. y?=w1820:bool)
        n1401 = Replace Array Subset(array=w1823, new element=w1820, index=w1819) -> (→"T Channel":bool[])
        n1402 = Index Array(array=string[] ["%#_g uA", "%#_g mK"], index=w1819) -> ()  [unwired: 1 out]
      }
      event Value Change {
        # "Update channel names on the small bottom panel when the names are changed."
        n1403 = event-data() -> ("NewVal"=→"AVS names small":T10)  [unwired: 1 in, 5 out]
      }
      event "I_list": Value Change {
        n1404 = event-data() -> ("NewVal"=w1832:T23[][])  [unwired: 1 in, 5 out]
        n1405 = local read "I_list_idx"() -> (w1831:i32)
        n1406 = Decrement(x=w1831) -> (x-1=w1830:i32)
        n1407 = Array Size(array=w1832) -> (size(s)=w1834:i32[])
        n1408 = Index Array(array=w1834) -> (element=→"I_list_idx_max":i32)  [unwired: 1 in]
        n1409 = Index Array(array=w1832, index (row)=w1830) -> (element=→"I_list[i]":T23[])  [unwired: 1 in]
      }
      event "I_list": Shortcut Menu Activation? {
        n1410 = event-data() -> ()  [unwired: 1 in, 7 out]
        n1411 = event-data() -> ()  [unwired: 2 in, 1 out]
      }
      event "I_list": Shortcut Menu Selection (App) {
        n1412 = event-data() -> ("ItemTag"=w1835:string)  [unwired: 1 in, 7 out]
        n1413 = case shown="\"APP_SC_COPY_DATA\"" w1835 {
          frame Default {
          }
          frame "APP_SC_PASTE_DATA" {
            n1414 = invoke class="App" method="Clipboard.Read"() -> ("Read Clipbrd"=w1838:string)  [unwired: 3 in, 2 out]
            n1415 = Spreadsheet String To Array(format string="%d", spreadsheet string=w1838) -> (array=w1836:dbl[][])  [unwired: 2 in]
            n1416 = local write "I_list"(w1836) -> ()
          }
          frame "APP_SC_COPY_DATA" {
            n1417 = local read "I_list"() -> (w1841:T23[][])
            n1418 = Array To Spreadsheet String(array=w1841, 3:"%d" ("format string")) -> (spreadsheet string=w1839:string)  [unwired: 1 in]
            n1419 = invoke class="App" method="Clipboard.Write"("Param 0"=w1839) -> ()  [unwired: 3 in, 4 out]
          }
        }
      }
      event "I_tofirst": Value Change {
        n1420 = event-data() -> ("OldVal"=w1842:bool)  [unwired: 1 in, 5 out]
        n1421 = local write "I_tofirst"(w1842) -> ()
        n1422 = property on="I_list_idx" class="DigNum (strict)"("Val(Sgnl)"=1 ("Value (Signaling)")) -> ()  [unwired: 2 in, 2 out]
      }
      event "I_next": Value Change {
        n1423 = event-data() -> ("OldVal"=w1844:bool)  [unwired: 1 in, 5 out]
        n1424 = local write "I_next"(w1844) -> ()
        n1425 = local read "I_list_idx"() -> (w1846:i32)
        n1426 = Increment(x=w1846) -> (x+1=w1845:i32)
        n1427 = property on="I_list_idx" class="DigNum (strict)"("Val(Sgnl)"=w1845) -> ()  [unwired: 2 in, 2 out]
      }
      event "I_prev": Value Change {
        n1428 = event-data() -> ("OldVal"=w1847:bool)  [unwired: 1 in, 5 out]
        n1429 = local write "I_prev"(w1847) -> ()
        n1430 = local read "I_list_idx"() -> (w1849:i32)
        n1431 = Decrement(x=w1849) -> (x-1=w1848:i32)
        n1432 = property on="I_list_idx" class="DigNum (strict)"("Val(Sgnl)"=w1848) -> ()  [unwired: 2 in, 2 out]
      }
      event "I_Clear": Value Change {
        n1433 = event-data() -> ()  [unwired: 1 in, 6 out]
        n1434 = flat-sequence {
          frame #0 {
            n1435 = local write "I_list"(T23[][] [] ("I_list")) -> ()
          }
          frame #1 {
            n1436 = property on="I_tofirst" class="Bool (strict)"("Val(Sgnl)"=TRUE ("Value (Signaling)")) -> ()  [unwired: 2 in, 2 out]
          }
        }
      }
      event "I_list_idx": Value Change {
        w1872 = 10  # Lines to scroll
        n1437 = event-data() -> ("NewVal"=w1855:i32)  [unwired: 1 in, 5 out]
        n1438 = Array Size(array="I_list") -> (size(s)=w1858:i32[])
        n1439 = Index Array(array=w1858) -> (element=w1856:i32)  [unwired: 1 in]
        n1440 = call "Current Time(double).vi"() -> ("Current Time (double)"=w1852:dbl)  [unwired: 6 in, 1 out]
        n1441 = local write "I_list_idx_max"(w1856) -> ()
        n1442 = local write "Time Old"(w1852) -> ()
        n1443 = In Range and Coerce(upper limit=w1856, x=w1855, lower limit=1) -> (coerced(x)=w1853:i32)  [unwired: 1 out]
        "I_list_idx" <- w1853
        n1444 = Decrement(x=w1853) -> (x-1=w1854:i32)
        n1445 = Initialize Array(FALSE, w1872) -> (w1873:bool[])
        n1446 = Index Array(array="I_list", index (row)=w1854) -> (element=w1875:T23[])  [unwired: 1 in]
        n1447 = local write "I_list[i]"(w1875) -> ()
        n1448 = Subtract(x=w1854, y=w1872) -> (x-y=w1862:i32)
        n1449 = Increment(x=w1862) -> (x+1=w1861:i32)
        n1450 = Decrement(x=w1872) -> (x-1=w1870:i32)
        n1451 = In Range and Coerce(upper limit=inf, x=w1861, lower limit=0) -> (coerced(x)=w1860:dbl)  [unwired: 1 out]
        n1452 = In Range and Coerce(upper limit=w1870, x=w1854, lower limit=0) -> (coerced(x)=w1867:i32)  [unwired: 1 out]
        n1453 = control-ref of="I_list"() -> (w1865:refnum<vi>)
        n1454 = Build Array(w1860, 0 ("element")) -> (w1866:dbl[])
        n1455 = Replace Array Subset(array=w1873, new element=TRUE ("new element/subarray"), index=w1867) -> (→"I_selection":bool[])
        n1456 = property class="Arr (strict)"(reference=w1865, "Index Values"=w1866) -> ()  [unwired: 1 in, 2 out]
      }
      event "Save to file": Value Change {
        n1457 = event-data() -> ()  [unwired: 1 in, 6 out]
        n1458 = call "File Dialog6"() -> ("selected path"=w1878:path, "cancelled"=w1877:bool)  [unwired: 12 in, 2 out]
        n1459 = case shown="False" w1877 {
          tunnel: w1878 -> [w1879 _]
          frame False {
            n1460 = local read "I_list"() -> (w1881:T23[][])
            n1461 = call <vilib>:"Write To Spreadsheet File (DBL).vi"("format (%.3f)"="%.1f", "2D data"=w1881, "file path (dialog if empty)"=w1879) -> ()  [unwired: 5 in, 1 out]
          }
          frame True {
          }
        }
      }
      event "Load from file": Value Change {
        n1462 = event-data() -> ()  [unwired: 1 in, 6 out]
        n1463 = call "File Dialog5"() -> ("selected path"=w1882:path, "cancelled"=w1883:bool)  [unwired: 12 in, 2 out]
        n1464 = case shown="False" w1883 {
          tunnel: w1882 -> [w1884 _]
          frame False {
            n1465 = call <vilib>:"Read From Spreadsheet File (DBL).vi"("file path (dialog if empty)"=w1884) -> ("all rows"=w1885:dbl[][])  [unwired: 6 in, 4 out]
            n1466 = local write "I_list"(w1885) -> ()
          }
          frame True {
          }
        }
      }
      event "Write to log": Value Change {
        n1467 = event-data() -> ()  [unwired: 1 in, 6 out]
        n1468 = Unbundle By Name(w1887) -> ("TempStabilized"=w1886:refnum<user-event>)
        n1469 = Generate User Event(user event=w1886, event data cluster=FALSE ("event data")) -> ()  [unwired: 2 in, 2 out]
      }
      event "Set Color": Value Change {
        n1470 = event-data() -> ()  [unwired: 1 in, 6 out]
        n1471 = property on="ColorBox" class="TabCtl (strict)"("Visible"=TRUE) -> ()  [unwired: 2 in, 2 out]
      }
      event "ColorBox": Mouse Move {
        n1472 = event-data() -> ("Coords"=w1892:T69)  [unwired: 1 in]
        n1473 = call <vilib>:"Picture to Pixmap.vi"("picture"="Colors") -> ("image data"=w1898:T68)  [unwired: 9 in, 1 out]
        n1474 = property on="Colors" class="Pict"() -> ("Position"=w1891:T75)  [unwired: 2 in, 2 out]
        n1475 = call <vilib>:"Unflatten Pixmap.vi"("image data"=w1898) -> ("24-bit pixmap"=w1893:u32[][])  [unwired: 4 in, 6 out]
        n1476 = Subtract(x=w1892, y=w1891) -> (x-y=w1896:T69)
        n1477 = Unbundle(w1896) -> ("Horizontal"=w1895:i32, "Vertical"=w1894:i32)
        n1478 = Index Array(array=w1893, index (row)=w1894, index (col)=w1895) -> (element=→"Color":u32)
      }
      event "ColorBox": Mouse Down {
        n1479 = event-data() -> ()  [unwired: 1 in, 8 out]
        n1480 = property on="ColorBox" class="TabCtl (strict)"("Visible"=FALSE) -> ()  [unwired: 2 in, 2 out]
      }
      event "Add Range": Value Change {
        n1481 = event-data() -> ()  [unwired: 1 in, 6 out]
        n1482 = call "Currents-Temp list  - add new range.vi"("List in"="I_list 2", "Array"="Array") -> ("Sorted list out"=w1901:dbl[][])  [unwired: 3 in, 1 out]
        n1483 = local write "I_list 2"(w1901) -> ()
      }
      event "I_list 2": Shortcut Menu Selection (User) {
        n1484 = event-data() -> ("CtlRef"=w1905:refnum<vi>, "Coords"=w1904:T69, "ItemPath"=w1903:string)  [unwired: 1 in]
        n1485 = case shown="\"Paste Data\"" w1903 {
          tunnel: w1905 -> [_ w1910 _ w1916 w1917]
          tunnel: w1904 -> [_ w1909 _ _ _]
          frame Default {
          }
          frame "Erase Range" {
            (unwired) TRUE
            n1486 = call "Get Clicked Array Index.vi"("Coords"=w1909, "Array 2"=w1910) -> ("Row"=w1908:i32)  [unwired: 8 in, 1 out]
            n1487 = local read "I_list 2"() -> (w1907:dbl[][])
            n1488 = call "Currents-Temp list - delete range.vi"("Numeric"=w1908, "I_list 2"=w1907) -> ("I_list"=w1906:dbl[][])  [unwired: 2 in]
            n1489 = local write "I_list 2"(w1906) -> ()
          }
          frame "Clear List" {
            n1490 = call "Currents-Temp list - check ranges.vi"() -> ("I_list out"=w1911:dbl[][])  [unwired: 5 in]
            n1491 = local write "I_list 2"(w1911) -> ()
          }
          frame "Copy Data" {
            n1492 = property class="Arr (strict)"(reference=w1916) -> ("Value"=w1912:dbl[][])  [unwired: 1 in, 2 out]
            n1493 = Array To Spreadsheet String(delimiter (Tab)="\t", array=w1912, 3:"%.4g" ("format string")) -> (spreadsheet string=w1915:string)
            n1494 = invoke class="App" method="Clipboard.Write"("Param 0"=w1915) -> ()  [unwired: 3 in, 4 out]
          }
          frame "Paste Data" {
            n1495 = invoke class="App" method="Clipboard.Read"() -> ("Read Clipbrd"=w1918:string)  [unwired: 3 in, 2 out]
            n1496 = Spreadsheet String To Array(delimiter (Tab)="\t", format string="%.4g", spreadsheet string=w1918) -> (array=w1921:dbl[][])  [unwired: 1 in]
            n1497 = property class="Arr (strict)"(reference=w1917, "Value"=w1921) -> ()  [unwired: 1 in, 2 out]
          }
        }
      }
    }
    "General" <- w25
  }
  n1498 = while {
    stop <- w1922 stop-if-true
    # "Main loop"
    n1499 = property on="start 2" class="Bool (strict)"() -> ("Value"=w1924:bool)  [unwired: 2 in, 2 out]
    n1500 = Wait (ms)(milliseconds to wait=u32 200) -> ()  [unwired: 1 out]
    n1501 = case shown="True" w1924 {
      frame False {
        n1502 = Wait (ms)(milliseconds to wait=u32 250) -> ()  [unwired: 1 out]
      }
      frame True {
        n1503 = while {
          i -> [w1936]
          stop <- "Stop" stop-if-true
          # "AVS/zBridge read-out"
          n1504 = case shown="False" "Pause" {
            tunnel: w1936 -> [w1939 _]
            frame False {
              # "for the first measurement set Stab.Time=12 s to do autoranging"
              n1505 = property on="Runtime Settings" class="Clust (strict)"() -> ("Value"=w1961:T27)  [unwired: 2 in, 2 out]
              n1506 = Unbundle By Name(w1961) -> ("Stabilisation Delay"=w1953:dbl, "Averages"=w1946:u16, "Last Channel"=w1960:i8, "Read AVS channels from"=w1959:i8)
              n1507 = local read "Active"() -> (w1944:T21)
              n1508 = property on="AVS type" class="Enum (strict)"() -> ("Value"=w1957:T60)  [unwired: 2 in, 2 out]
              n1509 = call "Split Exc&Range.vi"("Excitations 2"="Exc&Ranges") -> ("Excitations"=w1950:T29, "Ranges"=w1945:T76)  [unwired: 4 in]
              n1510 = property on="AVS VISA session" class="VISAName"() -> ("Value"=w1958:refnum<visa-resource-name>)  [unwired: 2 in, 2 out]
              n1511 = Cluster To Array(cluster=w1944) -> (array=w1943:bool[])
              n1512 = call "If First Iteration.vi"("Iteration"=w1939, "Value In"=w1953, "Default"=12.0) -> ("Value Out"=w1952:dbl)
              n1513 = case shown="\"AVS Emulation\"" w1957 {
                tunnel: w1958 -> [w1971 w1982 _ _ _]
                tunnel: w1952 -> [w1967 w1985 w1991 _ _]
                tunnel: w1946 -> [w1968 w1984 _ _ _]
                tunnel: w1960 -> [w1969 w1980 _ _ _]
                tunnel: w1959 -> [w1970 w1981 _ _ _]
                tunnel: w1950 -> [w1972 w1976 _ _ _]
                tunnel: [w1963 w1975 errorcluster {"status"=FALSE, "code"=0, "source"=""} ("error out") w2012 errorcluster {"status"=FALSE, "code"=0, "source"=""} ("error out")] -> w1949
                tunnel: w1945 -> [w1965 w1978 w1992 w2013 w2017]
                tunnel: "Autorange" -> [w1966 w1979 _ _ _]
                tunnel: [w1964 w1977 w1992 w2013 w2017] -> w1942
                tunnel: [w1962 w1974 w1990 w2006 dbl[] [] ("Data array")] -> w1947
                tunnel: w1943 -> [_ w1973 _ _ _]
                tunnel: "Data array" -> [_ _ _ w2002 _]
                frame "AVS47A (GPIB interface)" {
                  # "AVS 47 (GPIB)"
                  n1514 = call "AVS47IB_do_single_scan.vi"("AVS Port"=w1971, "Stabilization Delay"=w1967, "Autorange"=w1966, "Number of Averages"=w1968, "Last Channel"=w1969, "First Channel"=w1970, "Excitations"=w1972, "Ranges"=w1965) -> ("error out"=w1963:errorcluster, "R"=w1962:dbl[], "Ranges"=w1964:T77)  [unwired: 3 in, 2 out]
                }
                frame "AVS47B (RS232 interface)" {
                  # "AVS 47B (RS232)"
                  n1515 = Type Cast(type=refnum<visa-resource-name> refnum ("dup VISA session"), x=w1982) -> (*(type *) &x=w1986:refnum<visa-resource-name>)
                  n1516 = call "Scanner.vi"("STABILIZATION  DELAY"=w1985, "FIRST CH TO SCAN"=w1981, "LAST CH TO SCAN"=w1980, "Autorange"=w1979, "AVERAGE COUNT"=w1984, "Excitation"=w1976, "Range"=w1978, "VISA resource"=w1986, "array"=w1973) -> ("RI"=w1974:dbl[], "Range out"=w1977:T78, "error out 2"=w1975:errorcluster)  [unwired: 1 in, 3 out]
                }
                frame "AVS Emulation" {
                  n1517 = local read "I_in"() -> (w1988:T23[])
                  n1518 = Multiply(x=w1991, y=u32 1000 ("milliseconds to wait")) -> (x*y=w2000:dbl)
                  n1519 = Wait (ms)(milliseconds to wait=w2000) -> ()  [unwired: 1 out]
                  n1520 = Index Array(array=w1988, index=3) -> ()  [unwired: 1 out]
                  n1521 = property on="I" class="Arr (strict)"() -> ("Value"=w1999:dbl[])  [unwired: 2 in, 2 out]
                  n1522 = Multiply(x=1000.0, y=w1999) -> (x*y=w1994:dbl[])
                  n1523 = Index Array(array=w1994, index #1=2 ("index"), index #2=3 ("index")) -> (element #1=w1995:dbl, element #2=w1996:dbl)
                  n1524 = call "AVS Emulate.vi"("I_mc"=w1996, "I_still"=w1995, "Sampling time"=w1991) -> ("R"=w1990:dbl[])  [unwired: 1 out]
                }
                frame "Impedance Bridge" {
                  n1525 = local read "Bridge status"() -> (w2007:errorcluster)
                  n1526 = local read "zDll"() -> (w2014:path)
                  n1527 = call "Read Data from Single Channel.vi"("error in (no error)"=w2007, "zDll"=w2014) -> ("error out"=w2012:errorcluster, "Value"=w2011:dbl, "Scan parameters/Error string"=→"Par/Err":string, "Set number"=w2004:u8, "Error code"=→"Error code":u8, "Unit"=→"Unit":string, "ScanParameters out"=w2005:T79)  [unwired: 3 in]
                  "Set #" <- w2004
                  n1528 = call "ScanParameters FGV.vi"("Action"=Action."Write", "index"=w2004, "ScanParameters in"=w2005) -> ()  [unwired: 8 in, 1 out]
                  n1529 = Replace Array Subset(array=w2002, new element=w2011, index=w2004) -> (w2006:dbl[])
                }
                frame "Disabled", Default {
                }
              }
              "Bridge status" <- w1949
              n1530 = property on="Data array" class="Arr (strict)"("Val(Sgnl)"=w1947) -> ()  [unwired: 2 in, 2 out]
              n1531 = property on="Ranges" class="Clust (strict)"("Val(Sgnl)"=w1942) -> ()  [unwired: 2 in, 2 out]
              n1532 = property on="Delay" class="DigNum (strict)"() -> ("Value"=w1941:u32)  [unwired: 2 in, 2 out]
              n1533 = Multiply(x=u32 1000, y=w1941) -> (x*y=w1956:u32)
              n1534 = Wait (ms)(milliseconds to wait=w1956) -> ()  [unwired: 1 out]
            }
            frame True {
            }
          }
        }
        n1535 = while {
          stop <- w2019 stop-if-true
          (unwired) errorcluster {"status"=FALSE, "code"=0, "source"=""} ("Value")
          # "Current source control"
          n1536 = property on="CS status" class="Clust (strict)"() -> ("Value"=w2018:errorcluster)  [unwired: 2 in, 2 out]
          n1537 = stacked-sequence {
            seq-local: [w2047 _ _ _] -> [_ w2056 _ _]
            seq-local: [w2046 _ _ _] -> [_ w2055 _ _]
            seq-local: [_ w2056 _ _] -> [_ _ w2066 _]
            seq-local: [_ w2054 _ _] -> [_ _ w2065 _]
            tunnel: w2018 -> [w2045 _ _ _]
            frame #0 {
              # "Write 0 instead of the actual \ncurrent value to log if there \nis no current flowing."
              # "Read current CS status"
              n1538 = local read "CS ref"() -> (w2035:refnum<class "CS.lvclass">)
              n1539 = property on="TCS port" class="Ring (strict)" props=["Value"]() -> ()  [unwired: 2 in, 3 out]
              n1540 = call-dynamic "Read.vi"("CS in"=w2035, "error in (no error)"=w2045, "Optional"=FALSE) -> ("CS out"=w2047:refnum<class "CS.lvclass">, "I0"=w2038:T80, "I1"=w2039:T80, "I2"=w2040:T80, "I3"=w2041:T80, "error out"=w2046:errorcluster)  [unwired: 11 in]
              n1541 = Unbundle By Name(w2038) -> ("Current (string)"=w2033:string, "I?"=w2032:bool)
              n1542 = Unbundle By Name(w2039) -> ("Current (string)"=w2048:string, "I?"=w2031:bool)
              "Current1flow" <- w2031
              n1543 = Unbundle By Name(w2040) -> ("Current (string)"=w2036:string, "I?"=w2030:bool)
              n1544 = Unbundle By Name(w2041) -> ("Current (string)"=w2049:string, "I?"=w2029:bool)
              n1545 = call "CS Data Converter.vi"("CS Data"=w2038) -> ("CS Indicator"=→"I0":T81)
              n1546 = call "CS Data Converter.vi"("CS Data"=w2039) -> ("CS Indicator"=→"I1":T81)
              n1547 = call "CS Data Converter.vi"("CS Data"=w2040) -> ("CS Indicator"=→"I2":T81)
              n1548 = call "CS Data Converter.vi"("CS Data"=w2041) -> ("CS Indicator"=→"I3":T81)
              n1549 = Fract/Exp String To Number(string=w2033) -> (number=w2037:dbl)  [unwired: 3 in, 1 out]
              n1550 = Fract/Exp String To Number(string=w2048) -> (number=w2044:dbl)  [unwired: 3 in, 1 out]
              n1551 = Fract/Exp String To Number(string=w2036) -> (number=w2043:dbl)  [unwired: 3 in, 1 out]
              n1552 = Fract/Exp String To Number(string=w2049) -> (number=w2042:dbl)  [unwired: 3 in, 1 out]
              n1553 = Build Array(w2032, w2031, w2030, w2029) -> (w2028:bool[])
              n1554 = Not(x=w2028) -> (.not. x?=w2024:bool[])
              n1555 = Build Array(w2037, w2044, w2043, w2042) -> (w2027:dbl[])
              "I" <- w2027
              n1556 = for {
                tunnel: w2024 -> [w2053] mode=indexing
                tunnel: w2027 -> [w2052] mode=indexing
                tunnel: dbl[] [0.0, 0.0, 0.0, 0.0] ("t") -> [w2051] mode=indexing
                tunnel: [w2050] -> w2025 mode=indexing
                n1557 = Select(t=w2051, s=w2053, f=w2052) -> (s? t:f=w2050:dbl)
              }
              "Actual I" <- w2025
            }
            frame #1 {
              n1558 = Wait (ms)(milliseconds to wait=100) -> ()  [unwired: 1 out]
              n1559 = call <vilib>:"Clear Errors.vi"("error in (no error)"=w2055) -> ("error out"=w2054:errorcluster)  [unwired: 6 in]
            }
            frame #2 {
              # "Only send data to CS if\nnew value was entered"
              # "Set CS status"
              n1560 = call "CS OnOff & Gated and Current & Range.vi"("I in"="C_I0") -> ("OnOff & Gated"=w2077:T82, "Current & Range"=w2062:T83, "I out"=w2070:T84)  [unwired: 2 in]
              n1561 = call "CS OnOff & Gated and Current & Range.vi"("I in"="C_I0 2") -> ("OnOff & Gated"=w2076:T82, "Current & Range"=w2061:T83, "I out"=w2067:T84)  [unwired: 2 in]
              n1562 = call "CS OnOff & Gated and Current & Range.vi"("I in"="C_I0 3") -> ("OnOff & Gated"=w2073:T82, "Current & Range"=w2060:T83, "I out"=w2068:T84)  [unwired: 2 in]
              n1563 = call "CS OnOff & Gated and Current & Range.vi"("I in"="C_I0 4") -> ("OnOff & Gated"=w2072:T82, "Current & Range"=w2059:T83, "I out"=w2069:T84)  [unwired: 2 in]
              n1564 = local write "C_I0 2"(w2067) -> ()
              n1565 = local write "C_I0 3"(w2068) -> ()
              n1566 = local write "C_I0 4"(w2069) -> ()
              n1567 = local write "C_I0"(w2070) -> ()
              n1568 = local read "I_in"() -> (w2058:T23[])
              n1569 = Equal To 0?(x="CS Mode") -> (x = 0?=w2063:bool)
              n1570 = call "CS_set_channels.vi"("CS in"=w2066, "Current & Range0"=w2062, "Current & Range1"=w2061, "Current & Range 2"=w2060, "Current & Range3"=w2059, "error out"=w2065, "I 2"=w2058, "Auto?"=w2063) -> ("CS.lvclass out"=w2082:refnum<class "CS.lvclass">, "Current Changed?"=w2079:bool, "error out 2"=w2083:errorcluster)  [unwired: 9 in]
              n1571 = call-dynamic "Set Mode.vi"("CS.lvclass in"=w2082, "On&G 0"=w2077, "On&G 1"=w2076, "On&G 2"=w2073, "On&G 3"=w2072, "error in (no error)"=w2083) -> ("CS.lvclass out"=w2080:refnum<class "CS.lvclass">, "error out"=w2081:errorcluster)  [unwired: 12 in]
              n1572 = case shown="False" w2079 {
                selector: w2079 -> [_ w2084]
                frame False {
                }
                frame True {
                  n1573 = property on="Currents changed" class="Bool (strict)"("Val(Sgnl)"=w2084) -> ()  [unwired: 2 in, 2 out]
                }
              }
              n1574 = local write "CS ref"(w2080) -> ()
              n1575 = property on="CS status" class="Clust (strict)"("Value"=w2081) -> ()  [unwired: 2 in, 2 out]
            }
            frame #3 {
              n1576 = Wait (ms)(milliseconds to wait=100) -> ()  [unwired: 1 out]
            }
          }
          n1577 = local read "Stop"() -> (w2019:bool)
        }
        n1578 = while {
          stop <- w1928 stop-if-true
          # "zBridge status read-out"
          n1579 = property on="AVS type" class="Enum (strict)"() -> ("Value"=w1926:T60)  [unwired: 2 in, 2 out]
          n1580 = case shown="\"Impedance Bridge\"" w1926 {
            frame Default {
            }
            frame "Impedance Bridge" {
              n1581 = local read "Bridge status"() -> (w1933:errorcluster)
              n1582 = local read "zDll"() -> (w1934:path)
              n1583 = call "ScanStatus.vi"("error in (no error)"=w1933, "zDll"=w1934) -> ("error out"=w1932:errorcluster, "Status"=w1930:i32, "Channel"=w1931:i32)  [unwired: 7 in]
              n1584 = local write "Bridge status"(w1932) -> ()
              n1585 = call "zBridge Format Status.vi"("Status"=w1930, "Channel"=w1931) -> ("Status"=→"Status":T85, "Active channel"=→"Active channel":T86)  [unwired: 2 in]
            }
          }
          n1586 = Wait (ms)(milliseconds to wait=u32 200) -> ()  [unwired: 1 out]
          n1587 = local read "Stop"() -> (w1928:bool)
        }
      }
    }
    n1588 = local read "Stop"() -> (w1922:bool)
  }
  n1589 = disable-structure shown="Disabled" {
    frame Disabled {
      w2099 = string[] ["Paste Data from Clipboard"] ("item names")
      (unwired) enum32{"Page 1"}."Page 1" ("Tab Control 4")
      n1590 = call "Scan Data FGV.vi"() -> ()  [unwired: 11 in, 1 out]
      n1591 = property on="AVS Channel" class="DigNum (strict)"() -> ("Value"=w2087:i32)  [unwired: 2 in, 2 out]
      n1592 = local read item#-1() -> ()  [unwired: 1 out]
      n1593 = local read "I_in"() -> (w2094:T23[])
      n1594 = local read "Active"() -> ()  [unwired: 1 in]
      n1595 = Index Array(array=w2094) -> (element #1=w2090:T23, element #2=w2091:T23, element #3=w2092:T23, element #4=w2093:T23)  [unwired: 4 in]
      n1596 = property class="XYGraph (strict)" props=["YScale", "Mapping Mode"]() -> ()  [unwired: 2 in, 3 out]
      n1597 = property on="I" class="DigNum (strict)"("Val(Sgnl)"=w2090) -> ()  [unwired: 2 in, 2 out]
      n1598 = property on="I" class="DigNum (strict)"("Val(Sgnl)"=w2091) -> ()  [unwired: 2 in, 2 out]
      n1599 = property on="I" class="DigNum (strict)"("Val(Sgnl)"=w2092) -> ()  [unwired: 2 in, 2 out]
      n1600 = property on="I" class="DigNum (strict)"("Val(Sgnl)"=w2093) -> ()  [unwired: 2 in, 2 out]
      n1601 = Insert Menu Items(4:4, 7:w2099, 8:w2099) -> ()  [unwired: 3 in, 3 out]
      n1602 = Equal?(y=w2087) -> (x = y?=w2086:bool)  [unwired: 1 in]
      n1603 = Equal?(x=w2087, y=-1) -> (x = y?=w2089:bool)
      n1604 = Or(x=w2086, y=w2089) -> ()  [unwired: 1 out]
      n1605 = property on="ON" class="Boolean (strict)"() -> ("Value"=w2106:bool)  [unwired: 2 in, 2 out]
      n1606 = control-ref of="Active"() -> ()  [unwired: 1 out]
      n1607 = Exclusive Or(1:w2106, 2:TRUE ("x")) -> (0:w2105:bool)
      n1608 = property on="Toggle ON/OFF" class="Bool (strict)"("Value"=w2105) -> ()  [unwired: 2 in, 2 out]
      n1609 = control-ref of="I_list"() -> (w2101:refnum<vi>)
      n1610 = property class="Arr (strict)"(reference=w2101) -> ("Index Values"=w2102:u32[])  [unwired: 1 in, 2 out]
      n1611 = Index Array(array=w2102) -> (element=w2103:u32)  [unwired: 1 in]
      n1612 = property on="Tab Control 2" class="TabCtl (strict)"() -> ("Pages"=w2107:refnum<vi>[])  [unwired: 2 in, 2 out]
      n1613 = property on="I_list_idx" class="DigNum (strict)"("Val(Sgnl)"=w2103) -> ()  [unwired: 2 in, 2 out]
      n1614 = Index Array(array=w2107, index=1) -> (element=w2108:refnum<vi>)
      n1615 = Generate User Event(event data cluster="" ("event data")) -> ()  [unwired: 3 in, 2 out]
      n1616 = property class="Page"(reference=w2108, "PageVis"=TRUE ("Page Visible")) -> ()  [unwired: 1 in, 2 out]
      n1617 = property on="FB on" class="Enum (strict)" props=["Value"]() -> ()  [unwired: 2 in, 3 out]
      n1618 = local read "Error"() -> ()  [unwired: 1 out]
      n1619 = local read "Int"() -> ()  [unwired: 1 out]
      n1620 = local read item#-1() -> ()  [unwired: 1 out]
      n1621 = Initialize Array(0.0 ("element"), 4 ("dimension size")) -> (w2095:dbl[])
      n1622 = call "MGI Get Slope at Point.vi"() -> ()  [unwired: 11 in, 1 out]
      n1623 = local write "I_in"(w2095) -> ()
      n1624 = call "Write To Spreadsheet File (string) w Error.vi"() -> ()  [unwired: 10 in, 2 out]
    }
    frame Enabled {
    }
  }
